vi "StrainElectrical.vi"(4 "Use Switching Matrix":bool=TRUE, 6 "Use Parameter Analyzer":bool=TRUE, 8 "Use Stress Control":bool=TRUE, 9 "Switching Matrix VISA Session":refnum<visa-resource-name>="GPIB0::18::INSTR", 10 "Pameter Analyzer VISA Session":refnum<visa-resource-name>="GPIB0::27::INSTR", 11 "Stress Controller VISA Session":refnum<visa-resource-name>="COM7") -> ()   [LabVIEW 2014]
uses:
  Measurements/Instrument Sequence/Instrument Steps.ctl
  Measurements/Instrument Sequence/Action.ctl
  Measurements/Instrument Sequence/Instrument List.ctl
  Measurements/Plot Data/Chooseplot.ctl
  support/Instrument Status.ctl
  Measurements/Instrument Sequence/Instrument Stequence - Which Program.ctl
  Hardware Control/Spectrometer/Spectrometer Config.ctl
  Hardware Control/Spectrometer/Laser Settings.ctl
  Hardware Control/Spectrometer/Laser.ctl
  Hardware Control/Spectrometer/Filter.ctl
  Hardware Control/Spectrometer/Grating Detector Settings.ctl
  Hardware Control/Spectrometer/Grating.ctl
  Hardware Control/Spectrometer/Detector.ctl
  Hardware Control/Spectrometer/Acquisition Settings.ctl
  Hardware Control/Spectrometer/Spectrometer Refnum.ctl
  Measurements/Plot Data/Optical Spectrum Plot Refnum.ctl
  Hardware Control/Switches and Mirrors/SwitchesMirrors Config.ctl
  Hardware Control/Switches and Mirrors/SwitchesMirrors Status.ctl
  Hardware Control/Camera/Camera Config.ctl
  Hardware Control/Camera/Camera Settings.ctl
  Hardware Control/Stress Control/StressControl Config.ctl
  Hardware Control/Stress Control/StressControl Refnums.ctl
  Hardware Control/Parameter Analyzer/Parameter Analyzer Config.ctl
  Hardware Control/Parameter Analyzer/Parameter Analyzer Integration Parameters.ctl
  Hardware Control/Parameter Analyzer/Parameter Analyzer SMU Sweeping.ctl
  Hardware Control/Parameter Analyzer/Parameter Analyzer Sweep Spacing.ctl
  Hardware Control/Parameter Analyzer/Parameter Analyzer SMU Range.ctl
  Hardware Control/Parameter Analyzer/Parameter Analyzer SMU Sampling.ctl
  Hardware Control/Parameter Analyzer/Parameter Analyzer Sampling Parameters.ctl
  Hardware Control/Parameter Analyzer/Parameter Analyzer Stop Sampling Conditions.ctl
  Hardware Control/Parameter Analyzer/Parameter Analyzer Refnums.ctl
  Measurements/Plot Data/Electrical Data Plot Refnums.ctl
  Hardware Control/Switching Matrix/Switching Matrix Config.ctl
  Hardware Control/Switching Matrix/Switching Matrix Refnums.ctl
  Hardware Control/XYZ Stage/XYZ Config.ctl
  Hardware Control/XYZ Stage/XYZ Connection Settings.ctl
  Hardware Control/XYZ Stage/XYZ Stage Control.ctl
  Hardware Control/XYZ Stage/XYZ Coordinate Control.ctl
  Hardware Control/Autofocus/AutoFocus Config.ctl
  Hardware Control/Autofocus/ZScan.ctl
  <vilib>/Analysis/Matrix/Datatypes/RealMatrix.ctl
  Measurements/Instrument Sequence/Instrument Sequence Refnums.ctl
  Measurements/Strain Measurement/Strain Measurement Config.ctl
  Measurements/Strain Measurement/Strain Measurement Refnums.ctl
  Measurements/Plot Data/PlotData Config.ctl
  Measurements/Plot Data/Measurement.ctl
  Measurements/Plot Data/WhichInstrument.ctl
  Hardware Control/Parameter Analyzer/Electrical Data.ctl
  Hardware Control/Spectrometer/Spectral Data.ctl
  Measurements/Plot Data/PlotData Refnums.ctl
  support/User Event - Stop/User Event - Stop.lvlib
  support/Message Queue/Message Queue.lvlib
  <vilib>/Analysis/Matrix/NI_Matrix.lvlib
panel:
  out "Strain Measurement - Device ID":string caption="Device ID"
  out "Strain Measurement - Device Information":string caption="Device Information"
  out "Instrument Sequence - Status":T2={"Parameter Analyzer"=TRUE, "Switching Matrix"=FALSE, "Stress Control"=FALSE} caption="Instrument Status"
  in  "Opto Electro Mechanics Functions":T3(tab)
  out "Strain Measurement - Steps":T4 caption="Instrument Sequence"
  in  "Strain Measurement - New Sequence":bool
  in  "Strain Measurement - Add Step":bool
  in  "Strain Measurement - Delete Step":bool
  in  "Strain Measurement - Save Sequence":bool
  in  "Strain Measurement - Load Sequence":bool
  in  "Measurement Choice":T7(tab)
  in  "Instrument Sequence - Start":bool
  in  "Instrument Sequence - Pause":bool
  in  "Instrument Sequence - Stop":bool
  in  "Strain Measurement - Start":bool
  in  "Strain Measurement - Pause":bool
  in  "Strain Measurement - Stop":bool
  out "Strain Measurement - Sequence Progress":cluster{i32[], "Y":dbl[]}[](graph)=[{[], "Y"=[]}, {[0], "Y"=[0.0]}, {[1, 2, 3, 4], "Y"=[0.0, 0.0, 0.0, 0.0]}] caption="Measurement Progress"
  in  "Strain Measurement - Stress Sequence Parameters":T8 caption="Stress Parameters" {"# Points" max=1390}
  out "PlotData - Configuration":string caption="Configuration"
  in  "PlotData - Strain Sequence":i32(slide) caption="Strain Sequence" scale=0.0..84.0
  in  "PlotData - Instrument Sequence":i32(slide) caption="Instrument Sequence" scale=0.0..5.0
  out "PlotData - Choose Plot":T9
  in  "PlotData - Electrical Plot List":T10(tab)
  out "PlotData - Current Plot":cluster{"Time":dbl[], "SMU4":dbl[]}[](graph)=[{"Time"=[0.0, 0.30000000000000004, 0.6000000000000001, 0.9, 1.2000000000000002, 1.5, 1.8, 2.1, 2.4000000000000004, 2.7, 3.0, 3.3000000000000003, 3.6, 3.9000000000000004, 4.2, 4.5, 4.800000000000001, 5.1000000000000005, 5.4, 5.7, 6.0, 6.300000000000001, 6.6000000000000005, 6.9, 7.2, 7.5, 7.800000000000001, 8.1, 8.4, 8.700000000000001, 9.0, 9.3, 9.600000000000001, 9.9, 10.200000000000001, 10.5, 10.8, 11.100000000000001, 11.4, 11.700000000000001, 12.0, 12.3, 12.600000000000001, 12.9, 13.200000000000001, 13.5, 13.8, 14.100000000000001, 14.4, 14.700000000000001, 15.0, 15.3, 15.600000000000001, 15.9, 16.2, 16.5, 16.8, 17.1, 17.400000000000002, 17.7], "SMU4"=[9.99995e-06, 9.99995e-06, 9.99995e-06, 9.99997e-06, 9.99997e-06, 9.99997e-06, 9.99997e-06, 9.999980000000001e-06, 9.99997e-06, 9.999980000000001e-06, 9.99997e-06, 9.999980000000001e-06, 9.99997e-06, 9.99997e-06, 9.99997e-06, 9.99996e-06, 9.99996e-06, 9.99996e-06, 9.99996e-06, 9.99997e-06, 9.99997e-06, 9.999980000000001e-06, 9.99997e-06, 9.99997e-06, 9.99997e-06, 9.99997e-06, 9.99997e-06, 9.999980000000001e-06, 9.999980000000001e-06, 9.99996e-06, 9.99997e-06, 9.99996e-06, 9.99997e-06, 9.99997e-06, 9.99997e-06, 9.99997e-06, 9.999980000000001e-06, 9.99997e-06, 9.999980000000001e-06, 9.999980000000001e-06, 9.99997e-06, 9.99997e-06, 9.99997e-06, 9.99996e-06, 9.99996e-06, 9.99997e-06, 9.99997e-06, 9.99996e-06, 9.99996e-06, 9.99997e-06, 9.99997e-06, 9.99997e-06, 9.99997e-06, 9.99997e-06, 9.99996e-06, 9.99997e-06, 9.99997e-06, 9.99997e-06, 9.99997e-06, 9.99996e-06]}, {"Time"=[0.0, 0.30000000000000004, 0.6000000000000001, 0.9, 1.2000000000000002, 1.5, 1.8, 2.1, 2.4000000000000004, 2.7, 3.0, 3.3000000000000003, 3.6, 3.9000000000000004, 4.2, 4.5, 4.800000000000001, 5.1000000000000005, 5.4, 5.7, 6.0, 6.300000000000001, 6.6000000000000005, 6.9, 7.2, 7.5, 7.800000000000001, 8.1, 8.4, 8.700000000000001, 9.0, 9.3, 9.600000000000001, 9.9, 10.200000000000001, 10.5, 10.8, 11.100000000000001, 11.4, 11.700000000000001, 12.0, 12.3, 12.600000000000001, 12.9, 13.200000000000001, 13.5, 13.8, 14.100000000000001, 14.4, 14.700000000000001, 15.0, 15.3, 15.600000000000001, 15.9, 16.2, 16.5, 16.8, 17.1, 17.400000000000002, 17.7], "SMU4"=[-1.00004e-05, -1.000039e-05, -1.000039e-05, -1.0000409999999999e-05, -1.000039e-05, -1.000039e-05, -1.00004e-05, -1.000043e-05, -1.000042e-05, -1.0000409999999999e-05, -1.000039e-05, -1.000039e-05, -1.0000409999999999e-05, -1.00004e-05, -1.000038e-05, -1.000038e-05, -1.000039e-05, -1.000037e-05, -1.000038e-05, -1.000039e-05, -1.000039e-05, -1.000039e-05, -1.000039e-05, -1.000039e-05, -1.00004e-05, -1.000037e-05, -1.000038e-05, -1.000039e-05, -1.00004e-05, -1.00004e-05, -1.00004e-05, -1.000037e-05, -1.000037e-05, -1.000037e-05, -1.000036e-05, -1.000039e-05, -1.000038e-05, -1.000037e-05, -1.000036e-05, -1.000037e-05, -1.000038e-05, -1.000037e-05, -1.000038e-05, -1.000036e-05, -1.000037e-05, -1.000037e-05, -1.000037e-05, -1.000039e-05, -1.000038e-05, -1.000036e-05, -1.000037e-05, -1.000039e-05, -1.000036e-05, -1.000037e-05, -1.000038e-05, -1.00004e-05, -1.0000409999999999e-05, -1.000038e-05, -1.000038e-05, -1.00004e-05]}]
  out "PlotData - Voltage Plot":cluster{"Time":dbl[], "SMU4":dbl[]}[](graph)=[{"Time"=[0.0, 0.30000000000000004, 0.6000000000000001, 0.9, 1.2000000000000002, 1.5, 1.8, 2.1, 2.4000000000000004, 2.7, 3.0, 3.3000000000000003, 3.6, 3.9000000000000004, 4.2, 4.5, 4.800000000000001, 5.1000000000000005, 5.4, 5.7, 6.0, 6.300000000000001, 6.6000000000000005, 6.9, 7.2, 7.5, 7.800000000000001, 8.1, 8.4, 8.700000000000001, 9.0, 9.3, 9.600000000000001, 9.9, 10.200000000000001, 10.5, 10.8, 11.100000000000001, 11.4, 11.700000000000001, 12.0, 12.3, 12.600000000000001, 12.9, 13.200000000000001, 13.5, 13.8, 14.100000000000001, 14.4, 14.700000000000001, 15.0, 15.3, 15.600000000000001, 15.9, 16.2, 16.5, 16.8, 17.1, 17.400000000000002, 17.7], "SMU4"=[9.99995e-06, 9.99995e-06, 9.99995e-06, 9.99997e-06, 9.99997e-06, 9.99997e-06, 9.99997e-06, 9.999980000000001e-06, 9.99997e-06, 9.999980000000001e-06, 9.99997e-06, 9.999980000000001e-06, 9.99997e-06, 9.99997e-06, 9.99997e-06, 9.99996e-06, 9.99996e-06, 9.99996e-06, 9.99996e-06, 9.99997e-06, 9.99997e-06, 9.999980000000001e-06, 9.99997e-06, 9.99997e-06, 9.99997e-06, 9.99997e-06, 9.99997e-06, 9.999980000000001e-06, 9.999980000000001e-06, 9.99996e-06, 9.99997e-06, 9.99996e-06, 9.99997e-06, 9.99997e-06, 9.99997e-06, 9.99997e-06, 9.999980000000001e-06, 9.99997e-06, 9.999980000000001e-06, 9.999980000000001e-06, 9.99997e-06, 9.99997e-06, 9.99997e-06, 9.99996e-06, 9.99996e-06, 9.99997e-06, 9.99997e-06, 9.99996e-06, 9.99996e-06, 9.99997e-06, 9.99997e-06, 9.99997e-06, 9.99997e-06, 9.99997e-06, 9.99996e-06, 9.99997e-06, 9.99997e-06, 9.99997e-06, 9.99997e-06, 9.99996e-06]}, {"Time"=[0.0, 0.30000000000000004, 0.6000000000000001, 0.9, 1.2000000000000002, 1.5, 1.8, 2.1, 2.4000000000000004, 2.7, 3.0, 3.3000000000000003, 3.6, 3.9000000000000004, 4.2, 4.5, 4.800000000000001, 5.1000000000000005, 5.4, 5.7, 6.0, 6.300000000000001, 6.6000000000000005, 6.9, 7.2, 7.5, 7.800000000000001, 8.1, 8.4, 8.700000000000001, 9.0, 9.3, 9.600000000000001, 9.9, 10.200000000000001, 10.5, 10.8, 11.100000000000001, 11.4, 11.700000000000001, 12.0, 12.3, 12.600000000000001, 12.9, 13.200000000000001, 13.5, 13.8, 14.100000000000001, 14.4, 14.700000000000001, 15.0, 15.3, 15.600000000000001, 15.9, 16.2, 16.5, 16.8, 17.1, 17.400000000000002, 17.7], "SMU4"=[-1.00004e-05, -1.000039e-05, -1.000039e-05, -1.0000409999999999e-05, -1.000039e-05, -1.000039e-05, -1.00004e-05, -1.000043e-05, -1.000042e-05, -1.0000409999999999e-05, -1.000039e-05, -1.000039e-05, -1.0000409999999999e-05, -1.00004e-05, -1.000038e-05, -1.000038e-05, -1.000039e-05, -1.000037e-05, -1.000038e-05, -1.000039e-05, -1.000039e-05, -1.000039e-05, -1.000039e-05, -1.000039e-05, -1.00004e-05, -1.000037e-05, -1.000038e-05, -1.000039e-05, -1.00004e-05, -1.00004e-05, -1.00004e-05, -1.000037e-05, -1.000037e-05, -1.000037e-05, -1.000036e-05, -1.000039e-05, -1.000038e-05, -1.000037e-05, -1.000036e-05, -1.000037e-05, -1.000038e-05, -1.000037e-05, -1.000038e-05, -1.000036e-05, -1.000037e-05, -1.000037e-05, -1.000037e-05, -1.000039e-05, -1.000038e-05, -1.000036e-05, -1.000037e-05, -1.000039e-05, -1.000036e-05, -1.000037e-05, -1.000038e-05, -1.00004e-05, -1.0000409999999999e-05, -1.000038e-05, -1.000038e-05, -1.00004e-05]}]
  out "PlotData - dI/dV-V Characteristic":cluster{"V3":dbl[], "I1":dbl[]}[](graph) caption="Differential Resistance"
  out "PlotData - IV Characteristic":cluster{"V3":dbl[], "I1":dbl[]}[](graph) caption="Current Voltage Characteristic"
  out "PlotData - Optical Spectrum":cluster{"data":dbl[], "data":dbl[]}(graph)
  in  "Acquisition Mode":enum32{"Sweeping Mode", "Sampling Mode"}(tab)
  in  "SMU 4 - Sweeping":T11={"Start / Offset"=0.0, "Stop / Ratio"=1.0, "Step \n(linear only)"=0.01, "Compliance"=0.1, "Power \nCompliance"=0.0, "Mode"=4, "Function"=4, "Sweep Mode"=FALSE} caption="SMU 4" {"Function" items=["Disabled", "Var 1", "Var 2", "Var 1'", "Constant"]; "Mode" items=["V", "I", "V pulse", "I  pulse", "Common"]; "Power \nCompliance" format="%^.2e"; "Compliance" format="%^.2e"; "Step \n(linear only)" format="%^.4e"; "Stop / Ratio" format="%^.4e"; "Start / Offset" format="%^.4e"}
  in  "SMU 3 - Sweeping":T11={"Start / Offset"=0.0, "Stop / Ratio"=1.0, "Step \n(linear only)"=0.01, "Compliance"=0.1, "Power \nCompliance"=0.0, "Mode"=1, "Function"=4, "Sweep Mode"=FALSE} caption="SMU 3" {"Function" items=["Disabled", "Var 1", "Var 2", "Var 1'", "Constant"]; "Mode" items=["V", "I", "V pulse", "I  pulse", "Common"]; "Power \nCompliance" format="%^.2e"; "Compliance" format="%^.2e"; "Step \n(linear only)" format="%^.4e"; "Stop / Ratio" format="%^.4e"; "Start / Offset" format="%^.4e"}
  in  "SMU 2 - Sweeping":T11={"Start / Offset"=0.0, "Stop / Ratio"=1.0, "Step \n(linear only)"=0.01, "Compliance"=0.1, "Power \nCompliance"=0.0, "Mode"=1, "Function"=4, "Sweep Mode"=FALSE} caption="SMU 2" {"Function" items=["Disabled", "Var 1", "Var 2", "Var 1'", "Constant"]; "Mode" items=["V", "I", "V pulse", "I  pulse", "Common"]; "Power \nCompliance" format="%^.2e"; "Compliance" format="%^.2e"; "Step \n(linear only)" format="%^.4e"; "Stop / Ratio" format="%^.4e"; "Start / Offset" format="%^.4e"}
  in  "SMU 1 - Sweeping":T11={"Start / Offset"=0.0, "Stop / Ratio"=0.15, "Step \n(linear only)"=0.01, "Compliance"=0.1, "Power \nCompliance"=0.0, "Mode"=0, "Function"=1, "Sweep Mode"=TRUE} caption="SMU 1" {"Function" items=["Disabled", "Var 1", "Var 2", "Var 1'", "Constant"]; "Mode" items=["V", "I", "V pulse", "I  pulse", "Common"]; "Power \nCompliance" format="%^.2e"; "Compliance" format="%^.2e"; "Step \n(linear only)" format="%^.4e"; "Stop / Ratio" format="%^.4e"; "Start / Offset" format="%^.4e"}
  in  "Sweep Spacing":u16(ring) items=["linear", "log 10", "log 25", "log 50"]
  in  "Range":u16(ring) items=["auto", "fixed", "limited"]
  in  "Apply Sweeping Settings":bool
  in  "SMU4 - Sampling":T12={"Source"=0.1, "Compliance"=60.0, "Mode"=2, "Function"=TRUE} caption="SMU 4" {"Mode" items=["V", "I", "Common"]; "Compliance" format="%^.2e"; "Source" format="%^.3e"}
  in  "SMU2 - Sampling":T12={"Source"=0.0, "Compliance"=0.15, "Mode"=1, "Function"=TRUE} caption="SMU 2" {"Mode" items=["V", "I", "Common"]; "Compliance" format="%^.2e"; "Source" format="%^.3e"}
  in  "SMU3 - Sampling":T12={"Source"=0.0, "Compliance"=0.15, "Mode"=1, "Function"=TRUE} caption="SMU 3" {"Mode" items=["V", "I", "Common"]; "Compliance" format="%^.2e"; "Source" format="%^.3e"}
  in  "SMU1 - Sampling":T12={"Source"=0.15, "Compliance"=0.1, "Mode"=0, "Function"=TRUE} caption="SMU 1" {"Mode" items=["V", "I", "Common"]; "Compliance" format="%^.2e"; "Source" format="%^.3e"}
  in  "Stop Condition":T13={"Enable Delay (s)"=0.0, "Name"="", "Threshold"=0.0, "num. of events"=1, "Event"=0, "Stop Condition Enable"=FALSE} {"Event" items=["Value > Threshold", "Value < Threshold", "| Value | > | Threshold |", "| Value | < | Threshold |"]; "Threshold" format="%^.2e"; "Enable Delay (s)" format="%.1f"}
  in  "Sampling Parameters":T14={"Initial Interval (s)"=0.1, "Number of Samples"=60, "Total Sampling Time (s)"=10.0, "Hold Time (s)"=0.0, "Sampling Mode"=0, "Sampling Time"=0} {"Sampling Time" items=["Auto (linear only)", "No Limit", "Set Limit"]; "Sampling Mode" items=["Linear", "Log10", "Log25", "Log50", "Thinned Out"]; "Hold Time (s)" format="%.4f"; "Total Sampling Time (s)" format="%.1f"; "Initial Interval (s)" format="%^.3e"}
  in  "Apply Sampling Settings":bool
  in  "User Integration Time":T15={"Integration Time"=0, "Short Integration Time (s)"=8e-05, "Long Integration Time (s)"=0.0, "Wait Time Parameter"=1.0} caption="Input Integration Time" {"Long Integration Time (s)" scale=0.02..2.0; "Short Integration Time (s)" scale=8e-05..0.00192; "Integration Time" items=["Short", "Long"]; "Wait Time Parameter" format="%.1f"}
  in  "Plot List":T10(tab)
  out "Current Plot":cluster{"Time":dbl[], "SMU4":dbl[]}[](graph)=[{"Time"=[0.0, 0.30000000000000004, 0.6000000000000001, 0.9, 1.2000000000000002, 1.5, 1.8, 2.1, 2.4000000000000004, 2.7, 3.0, 3.3000000000000003, 3.6, 3.9000000000000004, 4.2, 4.5, 4.800000000000001, 5.1000000000000005, 5.4, 5.7, 6.0, 6.300000000000001, 6.6000000000000005, 6.9, 7.2, 7.5, 7.800000000000001, 8.1, 8.4, 8.700000000000001, 9.0, 9.3, 9.600000000000001, 9.9, 10.200000000000001, 10.5, 10.8, 11.100000000000001, 11.4, 11.700000000000001, 12.0, 12.3, 12.600000000000001, 12.9, 13.200000000000001, 13.5, 13.8, 14.100000000000001, 14.4, 14.700000000000001, 15.0, 15.3, 15.600000000000001, 15.9, 16.2, 16.5, 16.8, 17.1, 17.400000000000002, 17.7], "SMU4"=[9.99995e-06, 9.99995e-06, 9.99995e-06, 9.99997e-06, 9.99997e-06, 9.99997e-06, 9.99997e-06, 9.999980000000001e-06, 9.99997e-06, 9.999980000000001e-06, 9.99997e-06, 9.999980000000001e-06, 9.99997e-06, 9.99997e-06, 9.99997e-06, 9.99996e-06, 9.99996e-06, 9.99996e-06, 9.99996e-06, 9.99997e-06, 9.99997e-06, 9.999980000000001e-06, 9.99997e-06, 9.99997e-06, 9.99997e-06, 9.99997e-06, 9.99997e-06, 9.999980000000001e-06, 9.999980000000001e-06, 9.99996e-06, 9.99997e-06, 9.99996e-06, 9.99997e-06, 9.99997e-06, 9.99997e-06, 9.99997e-06, 9.999980000000001e-06, 9.99997e-06, 9.999980000000001e-06, 9.999980000000001e-06, 9.99997e-06, 9.99997e-06, 9.99997e-06, 9.99996e-06, 9.99996e-06, 9.99997e-06, 9.99997e-06, 9.99996e-06, 9.99996e-06, 9.99997e-06, 9.99997e-06, 9.99997e-06, 9.99997e-06, 9.99997e-06, 9.99996e-06, 9.99997e-06, 9.99997e-06, 9.99997e-06, 9.99997e-06, 9.99996e-06]}, {"Time"=[0.0, 0.30000000000000004, 0.6000000000000001, 0.9, 1.2000000000000002, 1.5, 1.8, 2.1, 2.4000000000000004, 2.7, 3.0, 3.3000000000000003, 3.6, 3.9000000000000004, 4.2, 4.5, 4.800000000000001, 5.1000000000000005, 5.4, 5.7, 6.0, 6.300000000000001, 6.6000000000000005, 6.9, 7.2, 7.5, 7.800000000000001, 8.1, 8.4, 8.700000000000001, 9.0, 9.3, 9.600000000000001, 9.9, 10.200000000000001, 10.5, 10.8, 11.100000000000001, 11.4, 11.700000000000001, 12.0, 12.3, 12.600000000000001, 12.9, 13.200000000000001, 13.5, 13.8, 14.100000000000001, 14.4, 14.700000000000001, 15.0, 15.3, 15.600000000000001, 15.9, 16.2, 16.5, 16.8, 17.1, 17.400000000000002, 17.7], "SMU4"=[-1.00004e-05, -1.000039e-05, -1.000039e-05, -1.0000409999999999e-05, -1.000039e-05, -1.000039e-05, -1.00004e-05, -1.000043e-05, -1.000042e-05, -1.0000409999999999e-05, -1.000039e-05, -1.000039e-05, -1.0000409999999999e-05, -1.00004e-05, -1.000038e-05, -1.000038e-05, -1.000039e-05, -1.000037e-05, -1.000038e-05, -1.000039e-05, -1.000039e-05, -1.000039e-05, -1.000039e-05, -1.000039e-05, -1.00004e-05, -1.000037e-05, -1.000038e-05, -1.000039e-05, -1.00004e-05, -1.00004e-05, -1.00004e-05, -1.000037e-05, -1.000037e-05, -1.000037e-05, -1.000036e-05, -1.000039e-05, -1.000038e-05, -1.000037e-05, -1.000036e-05, -1.000037e-05, -1.000038e-05, -1.000037e-05, -1.000038e-05, -1.000036e-05, -1.000037e-05, -1.000037e-05, -1.000037e-05, -1.000039e-05, -1.000038e-05, -1.000036e-05, -1.000037e-05, -1.000039e-05, -1.000036e-05, -1.000037e-05, -1.000038e-05, -1.00004e-05, -1.0000409999999999e-05, -1.000038e-05, -1.000038e-05, -1.00004e-05]}]
  out "Voltage Plot":cluster{"Time":dbl[], "SMU4":dbl[]}[](graph)=[{"Time"=[0.0, 0.30000000000000004, 0.6000000000000001, 0.9, 1.2000000000000002, 1.5, 1.8, 2.1, 2.4000000000000004, 2.7, 3.0, 3.3000000000000003, 3.6, 3.9000000000000004, 4.2, 4.5, 4.800000000000001, 5.1000000000000005, 5.4, 5.7, 6.0, 6.300000000000001, 6.6000000000000005, 6.9, 7.2, 7.5, 7.800000000000001, 8.1, 8.4, 8.700000000000001, 9.0, 9.3, 9.600000000000001, 9.9, 10.200000000000001, 10.5, 10.8, 11.100000000000001, 11.4, 11.700000000000001, 12.0, 12.3, 12.600000000000001, 12.9, 13.200000000000001, 13.5, 13.8, 14.100000000000001, 14.4, 14.700000000000001, 15.0, 15.3, 15.600000000000001, 15.9, 16.2, 16.5, 16.8, 17.1, 17.400000000000002, 17.7], "SMU4"=[9.99995e-06, 9.99995e-06, 9.99995e-06, 9.99997e-06, 9.99997e-06, 9.99997e-06, 9.99997e-06, 9.999980000000001e-06, 9.99997e-06, 9.999980000000001e-06, 9.99997e-06, 9.999980000000001e-06, 9.99997e-06, 9.99997e-06, 9.99997e-06, 9.99996e-06, 9.99996e-06, 9.99996e-06, 9.99996e-06, 9.99997e-06, 9.99997e-06, 9.999980000000001e-06, 9.99997e-06, 9.99997e-06, 9.99997e-06, 9.99997e-06, 9.99997e-06, 9.999980000000001e-06, 9.999980000000001e-06, 9.99996e-06, 9.99997e-06, 9.99996e-06, 9.99997e-06, 9.99997e-06, 9.99997e-06, 9.99997e-06, 9.999980000000001e-06, 9.99997e-06, 9.999980000000001e-06, 9.999980000000001e-06, 9.99997e-06, 9.99997e-06, 9.99997e-06, 9.99996e-06, 9.99996e-06, 9.99997e-06, 9.99997e-06, 9.99996e-06, 9.99996e-06, 9.99997e-06, 9.99997e-06, 9.99997e-06, 9.99997e-06, 9.99997e-06, 9.99996e-06, 9.99997e-06, 9.99997e-06, 9.99997e-06, 9.99997e-06, 9.99996e-06]}, {"Time"=[0.0, 0.30000000000000004, 0.6000000000000001, 0.9, 1.2000000000000002, 1.5, 1.8, 2.1, 2.4000000000000004, 2.7, 3.0, 3.3000000000000003, 3.6, 3.9000000000000004, 4.2, 4.5, 4.800000000000001, 5.1000000000000005, 5.4, 5.7, 6.0, 6.300000000000001, 6.6000000000000005, 6.9, 7.2, 7.5, 7.800000000000001, 8.1, 8.4, 8.700000000000001, 9.0, 9.3, 9.600000000000001, 9.9, 10.200000000000001, 10.5, 10.8, 11.100000000000001, 11.4, 11.700000000000001, 12.0, 12.3, 12.600000000000001, 12.9, 13.200000000000001, 13.5, 13.8, 14.100000000000001, 14.4, 14.700000000000001, 15.0, 15.3, 15.600000000000001, 15.9, 16.2, 16.5, 16.8, 17.1, 17.400000000000002, 17.7], "SMU4"=[-1.00004e-05, -1.000039e-05, -1.000039e-05, -1.0000409999999999e-05, -1.000039e-05, -1.000039e-05, -1.00004e-05, -1.000043e-05, -1.000042e-05, -1.0000409999999999e-05, -1.000039e-05, -1.000039e-05, -1.0000409999999999e-05, -1.00004e-05, -1.000038e-05, -1.000038e-05, -1.000039e-05, -1.000037e-05, -1.000038e-05, -1.000039e-05, -1.000039e-05, -1.000039e-05, -1.000039e-05, -1.000039e-05, -1.00004e-05, -1.000037e-05, -1.000038e-05, -1.000039e-05, -1.00004e-05, -1.00004e-05, -1.00004e-05, -1.000037e-05, -1.000037e-05, -1.000037e-05, -1.000036e-05, -1.000039e-05, -1.000038e-05, -1.000037e-05, -1.000036e-05, -1.000037e-05, -1.000038e-05, -1.000037e-05, -1.000038e-05, -1.000036e-05, -1.000037e-05, -1.000037e-05, -1.000037e-05, -1.000039e-05, -1.000038e-05, -1.000036e-05, -1.000037e-05, -1.000039e-05, -1.000036e-05, -1.000037e-05, -1.000038e-05, -1.00004e-05, -1.0000409999999999e-05, -1.000038e-05, -1.000038e-05, -1.00004e-05]}]
  out "Differential Resistance":cluster{"V3":dbl[], "I1":dbl[]}[](graph)
  out "Current Voltage Characteristic":cluster{"V3":dbl[], "I1":dbl[]}[](graph)
  in  "Parameter Analyzer - Measure":bool
  in  "Parameter Analyzer - Save Measurement":bool
  in  "Switching Matrix":enum32{"Switching Matrix"}(tab)
  in  "Switching Matrix Connections":T16(array[cluster])=[{"Connections"=[FALSE, FALSE, FALSE, FALSE, FALSE, FALSE, FALSE, FALSE, FALSE, FALSE, FALSE, FALSE], "Connection Type"=enum."Make - Break"}, {"Connections"=[FALSE, FALSE, FALSE, FALSE, FALSE, FALSE, FALSE, FALSE, FALSE, FALSE, FALSE, FALSE], "Connection Type"=enum."Make - Break"}, {"Connections"=[FALSE, FALSE, FALSE, FALSE, FALSE, FALSE, FALSE, FALSE, FALSE, FALSE, FALSE, FALSE], "Connection Type"=enum."Make - Break"}, {"Connections"=[FALSE, FALSE, FALSE, FALSE, FALSE, FALSE, FALSE, FALSE, FALSE, FALSE, FALSE, FALSE], "Connection Type"=enum."Make - Break"}, {"Connections"=[TRUE, TRUE, TRUE, TRUE, TRUE, TRUE, TRUE, TRUE, TRUE, TRUE, TRUE, TRUE], "Connection Type"=enum."Make - Break"}, {"Connections"=[FALSE, FALSE, FALSE, FALSE, FALSE, FALSE, FALSE, FALSE, FALSE, FALSE, FALSE, FALSE], "Connection Type"=enum."Make - Break"}, {"Connections"=[FALSE, FALSE, FALSE, FALSE, FALSE, FALSE, FALSE, FALSE, FALSE, FALSE, FALSE, FALSE], "Connection Type"=enum."Make - Break"}, {"Connections"=[FALSE, FALSE, FALSE, FALSE, FALSE, FALSE, FALSE, FALSE, FALSE, FALSE, FALSE, FALSE], "Connection Type"=enum."Make - Break"}]
  in  "Disconnect All":bool
  in  "Ground All":bool
  in  "Uniaxial Stress Controller":enum32{"Uniaxial Stress Controller"}(tab)
  in  "Destination (°)":dbl min=-2000000000.0 max=2000000000.0 format="%.6f"
  out "Position (°)":dbl format="%.6g"
  in  "Mechanism Motion":u16(ring) items=["Absolute", "Relative"]
  in  "Apply Stress":bool
  in  "Stop":bool
  in  "Speed (°/s)":dbl=4.0 min=0.0 max=4.0 format="%.6f"
  in  "Status Polling Time (ms)":u32=500
  out "Status Log":string
  out "Last Operation":string="Camera Settings Updated"
  # "SMU1"
  # "SMU2"
  # "SMU3"
  # "SMU4"
  # "GND"
  # "L1"
  # "R1"
  # "L2"
  # "R2"
  # "L3"
  # "R3"
  # "L6"
  # "R6"
  # "L7"
  # "R7"
  # "L8"
  # "R8"
  # "LICENSED MATERIALS – PROPERTY OF IBM\nCopyright IBM Corp. 2016,\nALL RIGHTS RESERVED"
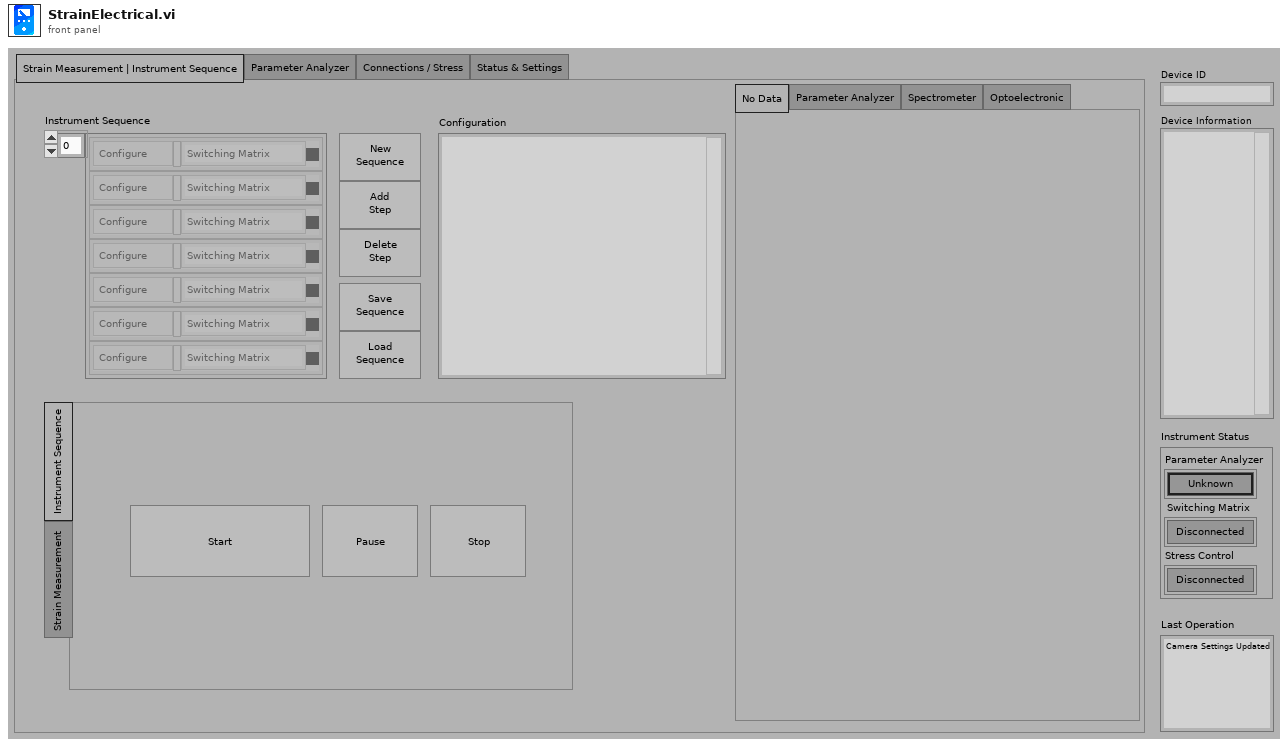
[diagram p1: front panel]
types:
  T1 = typedef "Instrument Status.ctl" = bool
  T2 = cluster{"Parameter Analyzer":T1, "Switching Matrix":T1, "Stress Control":T1}
  T3 = enum32{"Strain Measurement | Instrument Sequence", "Parameter Analyzer", "Connections / Stress", "Status & Settings"}
  T4 = typedef "Instrument Steps.ctl" = cluster{"Action":T5, "Configuration":variant, "Instrument":T6, "Status":enum8{"False", "True", "Mixed"}}[]
  T5 = typedef "Action.ctl" = enum32{"Configure", "Measure"}
  T6 = typedef "Instrument List.ctl" = enum32{"Unknown Instrument", "Switching Matrix", "Parameter Analyzer", "Optical Spectrometer", "Optoelectronic", "Autofocus"}
  T7 = enum32{"Instrument Sequence", "Strain Measurement "}
  T8 = cluster{"Max Stress":ext, "# Points":u32, "Initial Direction":enum16{"Tension", "Compression"}}
  T9 = typedef "Chooseplot.ctl" = enum32{"No Data", "Parameter Analyzer", "Spectrometer", "Optoelectronic"}
  T10 = enum32{"Current & Voltage Traces", "Four | Two Probe"}
  T11 = cluster{"Start / Offset":dbl, "Stop / Ratio":dbl, "Step \n(linear only)":dbl, "Compliance":dbl, "Power \nCompliance":dbl, "Mode":u32, "Function":i32, "Sweep Mode":bool}
  T12 = cluster{"Source":dbl, "Compliance":dbl, "Mode":u32, "Function":bool}
  T13 = cluster{"Enable Delay (s)":dbl, "Name":string, "Threshold":dbl, "num. of events":i32, "Event":i32, "Stop Condition Enable":bool}
  T14 = cluster{"Initial Interval (s)":dbl, "Number of Samples":i32, "Total Sampling Time (s)":dbl, "Hold Time (s)":dbl, "Sampling Mode":i32, "Sampling Time":i32}
  T15 = cluster{"Integration Time":u32, "Short Integration Time (s)":dbl, "Long Integration Time (s)":dbl, "Wait Time Parameter":dbl}
  T16 = cluster{"Connections":bool[], "Connection Type":enum16{"Disconnected", "Make - Break", "Break - Make"}}[]
  T17 = typedef "Instrument Stequence - Which Program.ctl" = enum16{"Full Instrument Palette", "Strain Electrical"}
  T18 = typedef "Message Queue.lvlib/All Message Queues.ctl" = cluster{"Message Handler Loop":refnum<queue>, "Parameter Analyzer":refnum<queue>, "Switching Matrix":refnum<queue>, "Stress Control":refnum<queue>, "Optical Spectrometer":refnum<queue>, "Switches & Mirrors":refnum<queue>, "Camera":refnum<queue>, "XYZ Stage":refnum<queue>, "AutoFocus":refnum<queue>, "Optoelectronic":refnum<queue>, "Save Data":refnum<queue>, "Plot Data":refnum<queue>, "Instrument Sequence":refnum<queue>, "Strain Measurement":refnum<queue>}
  T19 = typedef "Notifiers.ctl" = cluster{"Message Handler Loop":T20, "Parameter Analyzer":T21, "Switching Matrix":T22, "Stress Control":T23, "Optical Spectrometer":T24, "Switches & Mirrors":T25, "Camera":T26, "XYZ Stage":T27, "AutoFocus":T28, "Optoelectronic":T29, "Save Data":T30, "Plot Data":T30, "Instrument Sequence":T31, "Strain Measurement":cluster{"Status":refnum<notifier>, "Exit":refnum<notifier>, "Ready":refnum<notifier>}}
  T20 = typedef "Message Handler Loop Notifiers.ctl" = cluster{"Status":refnum<notifier>, "Instrument Data":refnum<notifier>, "Exit":refnum<notifier>, "Ready":refnum<notifier>}
  T21 = typedef "Parameter Analyzer Notifiers.ctl" = cluster{"Status":refnum<notifier>, "Instrument Data":refnum<notifier>, "Measurement":refnum<notifier>, "Exit":refnum<notifier>, "Ready":refnum<notifier>}
  T22 = typedef "Switching Matrix Notifiers.ctl" = cluster{"Status":refnum<notifier>, "Instrument Data":refnum<notifier>, "Measurement":refnum<notifier>, "Exit":refnum<notifier>, "Ready":refnum<notifier>}
  T23 = typedef "StressControl Notifiers.ctl" = cluster{"Status":refnum<notifier>, "Instrument Data":refnum<notifier>, "Measurement":refnum<notifier>, "Exit":refnum<notifier>, "Ready":refnum<notifier>}
  T24 = typedef "Spectrometer Notifiers.ctl" = cluster{"Status":refnum<notifier>, "Instrument Data":refnum<notifier>, "Measurement":refnum<notifier>, "Exit":refnum<notifier>, "Ready":refnum<notifier>}
  T25 = typedef "SwitchesMirrors Notifiers.ctl" = cluster{"Status":refnum<notifier>, "Instrument Data":refnum<notifier>, "Exit":refnum<notifier>, "Ready":refnum<notifier>}
  T26 = typedef "Camera Notifiers.ctl" = cluster{"Status":refnum<notifier>, "Instrument Data":refnum<notifier>, "Measurement":refnum<notifier>, "Exit":refnum<notifier>, "Ready":refnum<notifier>}
  T27 = typedef "XYZ Notifications.ctl" = cluster{"Status":refnum<notifier>, "Instrument Data":refnum<notifier>, "Measurement":refnum<notifier>, "Exit":refnum<notifier>, "Ready":refnum<notifier>}
  T28 = typedef "Autofocus Notifiers.ctl" = cluster{"Status":refnum<notifier>, "Instrument Data":refnum<notifier>, "Measurement":refnum<notifier>, "Exit":refnum<notifier>, "Ready":refnum<notifier>}
  T29 = typedef "Optoelectronic Notifiers.ctl" = cluster{"Status":refnum<notifier>, "Instrument Data":refnum<notifier>, "Measurement":refnum<notifier>, "Exit":refnum<notifier>, "Ready":refnum<notifier>}
  T30 = typedef "SaveData Notifiers.ctl" = cluster{"Status":refnum<notifier>, "Exit":refnum<notifier>, "Ready":refnum<notifier>}
  T31 = typedef "Instrument Sequence Notifiers.ctl" = cluster{"Status":refnum<notifier>, "Instrument Data":refnum<notifier>, "Measurement":refnum<notifier>, "Exit":refnum<notifier>, "Ready":refnum<notifier>}
  T32 = typedef "Configuration.ctl" = cluster{"Parameter Analizer":T33, "Switching Matrix":T41, "Stress Control":T42, "Optical Spectrometer":T43, "Switches & Mirrors":T51, "Camera":T53, "XYZ Stage":T55, "AutoFocus":T59, "Sava Data":T62, "PlotData":T66, "Instrument Sequence":T70, "Strain Measurement":T71}
  T33 = typedef "Parameter Analyzer Config.ctl" = cluster{"Parameter Analyzer VISA Session":refnum<visa-resource-name>, "Sweeping Time Parameters":T34, "Acquisition Mode":enum32{"Sweeping Mode", "Sampling Mode"}, "Status Polling Time (ms)":u32, "Comment":string, "SMU 1 - Sweeping":T35, "SMU 2 - Sweeping":T35, "SMU 3 - Sweeping":T35, "SMU 4 - Sweeping":T35, "Sweep Spacing":T36, "Range":T37, "SMU1 - Sampling":T38, "SMU2 - Sampling":T38, "SMU3 - Sampling":T38, "SMU4 - Sampling":T38, "Sampling Time Parameters":T39, "Stop Condition":T40}
  T34 = typedef "Parameter Analyzer Integration Parameters.ctl" = cluster{"Integration Time":u32, "Short Integration Time (s)":dbl, "Long Integration Time (s)":dbl, "Wait Time Parameter":dbl}
  T35 = typedef "Parameter Analyzer SMU Sweeping.ctl" = cluster{"Start / Offset":dbl, "Stop / Ratio":dbl, "Step \n(linear only)":dbl, "Compliance":dbl, "Power \nCompliance":dbl, "Mode":u32, "Function":i32, "Sweep Mode":bool}
  T36 = typedef "Parameter Analyzer Sweep Spacing.ctl" = u16
  T37 = typedef "Parameter Analyzer SMU Range.ctl" = u16
  T38 = typedef "Parameter Analyzer SMU Sampling.ctl" = cluster{"Source":dbl, "Compliance":dbl, "Mode":u32, "Function":bool}
  T39 = typedef "Parameter Analyzer Sampling Parameters.ctl" = cluster{"Initial Interval (s)":dbl, "Number of Samples":i32, "Total Sampling Time (s)":dbl, "Hold Time (s)":dbl, "Sampling Mode":i32, "Sampling Time":i32}
  T40 = typedef "Parameter Analyzer Stop Sampling Conditions.ctl" = cluster{"Enable Delay (s)":dbl, "Name":string, "Threshold":dbl, "num. of events":i32, "Event":i32, "Stop Condition Enable":bool}
  T41 = typedef "Switching Matrix Config.ctl" = cluster{"Switching Matrix VISA Session":refnum<visa-resource-name>, "Connections":cluster{"Connections":bool[], "Connection Type":enum16{"Disconnected", "Make - Break", "Break - Make"}}[]}
  T42 = typedef "StressControl Config.ctl" = cluster{"Stress Control VISA Session":refnum<visa-resource-name>, "Axis":i32, "Motion":u16, "Destination (°)":dbl, "Speed (°/s)":dbl, "Position (°)":dbl}
  T43 = typedef "Spectrometer Config.ctl" = cluster{"Laser Settings":T44, "Spectrometer Settings":T47, "Acquisition Settings":T50, "Path":path}
  T44 = typedef "Laser Settings.ctl" = cluster{"Laser Wavelength":T45, "Neutral Density Filter":T46}
  T45 = typedef "Laser.ctl" = enum16{"633 nm", "784 nm", "532 nm", "365 nm"}
  T46 = typedef "Filter.ctl" = enum16{"100%", "50%", "25%", "10%", "1%", "0.1%", "0.01%"}
  T47 = typedef "Grating Detector Settings.ctl" = cluster{"Confocal Hole Size (µm)":dbl, "Grating":T48, "Detector":T49}
  T48 = typedef "Grating.ctl" = u16
  T49 = typedef "Detector.ctl" = enum16{"InGaAs Array", "Silicon CCD"}
  T50 = typedef "Acquisition Settings.ctl" = cluster{"Acquisition Mode":enum16{"Single Window", "Multi-Window"}, "Spectal Position (nm)":dbl, "From (nm)":dbl, "To (nm)":dbl, "Integration Time (s)":dbl, "Number of Accumulations":i32, "AutoScanning":bool, "Spike Removal":bool}
  T51 = typedef "SwitchesMirrors Config.ctl" = cluster{"Relay VISA Session":refnum<visa-resource-name>, "Switches":T52, "Delays (ms)":cluster{"Laser":u32, "Video":u32}}
  T52 = typedef "SwitchesMirrors Status.ctl" = cluster{"Laser":bool, "Video":bool}
  T53 = typedef "Camera Config.ctl" = cluster{"Settings":T54}
  T54 = typedef "Camera Settings.ctl" = cluster{"Pixel clock":i32, "Frame rate":dbl, "Exposure time":dbl, "Master Gain":i32, "Red Gain":i32, "Green Gain":i32, "Blue Gain":i32, "Auto Gain":bool, "White-balance":bool, "Color Correction":bool}
  T55 = typedef "XYZ Config.ctl" = cluster{"Connection Settings":T56, "Manual Control":T57, "Coordinate Control":T58}
  T56 = typedef "XYZ Connection Settings.ctl" = cluster{"Tango VISA":refnum<visa-resource-name>, "Baudrate":i32, "Show Protocol?":bool}
  T57 = typedef "XYZ Stage Control.ctl" = cluster{"North":bool, "South":bool, "West":bool, "East":bool, "Up":bool, "Down":bool, "Stop":bool, "XY Step":dbl, "Z step":dbl}
  T58 = typedef "XYZ Coordinate Control.ctl" = cluster{"Motion Mode":enum16{"Absolute", "Relative"}, "Destination [mm]":dbl[]}
  T59 = typedef "AutoFocus Config.ctl" = cluster{"Matching Criteria":cluster{"Minimum Score":sgl, "Color Score Weight":sgl, "Minimum Contrast":i32, "Match Mode":u32, "Match Feature Mode":u32, "Subpixel Accuracy":bool, "Color Sensitivity":u32, "Search Strategy":u32}, "Z Scan Parameters":T60, "Displacement":dbl, "Transformation Matrix":T61}
  T60 = typedef "ZScan.ctl" = cluster{"Z Range":ext, "Resolution":dbl, "Initial Direction":enum16{"Up", "Down"}, "Focus Threshold":dbl, "Ascent Constant":dbl}
  T61 = typedef "NI_Matrix.lvlib/RealMatrix.ctl" = dbl[][]
  T62 = typedef "SaveData Config.ctl" = cluster{"Workspace Info":T63, "Instrument Configuration":T64, "Stress Motor Position":dbl, "Electrical Measurement":cluster{"Sequence":dbl[], "V1":dbl[], "V2":dbl[], "V3":dbl[], "V4":dbl[], "I1":dbl[], "I2":dbl[], "I3":dbl[], "I4":dbl[]}, "Optical Spectrum":T65}
  T63 = typedef "SaveData Workspace Info.ctl" = cluster{"Device Name":string, "Device Info":string, "Path":path}
  T64 = typedef "SaveData Instrument Configuration.ctl" = cluster{"Instrument":T6, "Configuration":string}
  T65 = typedef "Spectral Data.ctl" = cluster{"Intensity":dbl[], "Wavelength":dbl[], "Energy":dbl[], "Raman Shift":dbl[], "Detector Temperature":dbl}
  T66 = typedef "PlotData Config.ctl" = cluster{"Sliders":cluster{"Strain Sequence":i32, "Instrument Sequence":i32}, "Measurement":T67, "Instrument Steps":T4, "Strain Points":dbl[]}
  T67 = typedef "Measurement.ctl" = cluster{"Which Instrument?":T68, "Electrical Measurement":T69, "Measurement Mode":enum16{"Sweeping Mode", "Sampling Mode"}, "Optical Spectrum":T65}
  T68 = typedef "WhichInstrument.ctl" = enum16{"No Plot", "Spectrometer", "Parameter Analyzer", "Optoelectronic"}
  T69 = typedef "Electrical Data.ctl" = cluster{"Sequence":dbl[], "V1":dbl[], "V2":dbl[], "V3":dbl[], "V4":dbl[], "I1":dbl[], "I2":dbl[], "I3":dbl[], "I4":dbl[]}
  T70 = typedef "Instrument Sequence Config.ctl" = cluster{"Caller VI":enum16{"User", "Stress Measurement VI"}}
  T71 = typedef "Strain Measurement Config.ctl" = cluster{"Stress Sequence ":cluster{"Max Motor Position":ext, "# Intermediate Points":u32, "Initial Direction":enum16{"Tension", "Compression"}}, "Track?":bool}
  T72 = typedef "Spectrometer Refnum.ctl" = cluster{"Instrument Status":refnum<vi>, "Optical Spectrum Plot":T73, "Laser":refnum<vi>, "Filter":refnum<vi>, "Laser ON?":refnum<vi>, "Hole":refnum<vi>, "Grating":refnum<vi>, "Detector":refnum<vi>, "Acquisition Mode":refnum<vi>, "Spectal Position":refnum<vi>, "From":refnum<vi>, "To":refnum<vi>, "Integration Time":refnum<vi>, "Accumulations":refnum<vi>, "AutoScanning":refnum<vi>, "Spike Removal":refnum<vi>, "Acquisition Mode Panel":refnum<vi>}
  T73 = typedef "Optical Spectrum Plot Refnum.ctl" = cluster{"Plot List":refnum<vi>, "Optical Spectrum vs Energy":refnum<vi>, "Optical Spectrum vs Wavelength":refnum<vi>, "Optical Spectrum vs Raman Shift":refnum<vi>, "Detector Temperature":refnum<vi>}
  T74 = typedef "StressControl Refnums.ctl" = cluster{"Instrument Status":refnum<vi>, "Position":refnum<vi>, "Mecahnism Motion":refnum<vi>, "Destination":refnum<vi>, "Apply Stress":refnum<vi>, "Stop":refnum<vi>, "Stress Control VISA":refnum<vi>}
  T75 = typedef "Parameter Analyzer Refnums.ctl" = cluster{"Status":refnum<vi>, "Electrical Measurement":refnum<vi>, "Plots":T76, "HP Integration Time":refnum<vi>, "VISA":refnum<vi>, "Sweeping Time Parameters":refnum<vi>, "Acquisition Mode":refnum<vi>, "SMU 1 - Sweeping":refnum<vi>, "SMU 2 - Sweeping":refnum<vi>, "SMU 3 - Sweeping":refnum<vi>, "SMU 4 - Sweeping":refnum<vi>, "Sweep Spacing":refnum<vi>, "Range":refnum<vi>, "SMU1 - Sampling":refnum<vi>, "SMU2 - Sampling":refnum<vi>, "SMU3 - Sampling":refnum<vi>, "SMU4 - Sampling":refnum<vi>, "Sampling Time Parameters":refnum<vi>, "Stop Condition":refnum<vi>, "Instrument Status":refnum<vi>}
  T76 = typedef "Electrical Data Plot Refnums.ctl" = cluster{"Plot List":refnum<vi>, "Voltage Plot":refnum<vi>, "Current Plot":refnum<vi>, "IV Characteristic":refnum<vi>, "dI/dV-V Characteristic":refnum<vi>}
  T77 = cluster{"SMU 1 - Sweeping":cluster{"Start / Offset":dbl, "Stop / Ratio":dbl, "Step (linear only)":dbl, "Compliance":dbl, "Power Compliance":dbl, "Mode":u32, "Function":i32, "Sweep Mode":bool}, "SMU 2 - Sweeping":cluster{"Start / Offset":dbl, "Stop / Ratio":dbl, "Step (linear only)":dbl, "Compliance":dbl, "Power Compliance":dbl, "Mode":u32, "Function":i32, "Sweep Mode":bool}, "SMU 3 - Sweeping":cluster{"Start / Offset":dbl, "Stop / Ratio":dbl, "Step (linear only)":dbl, "Compliance":dbl, "Power Compliance":dbl, "Mode":u32, "Function":i32, "Sweep Mode":bool}, "SMU 4 - Sweeping":cluster{"Start / Offset":dbl, "Stop / Ratio":dbl, "Step (linear only)":dbl, "Compliance":dbl, "Power Compliance":dbl, "Mode":u32, "Function":i32, "Sweep Mode":bool}, "Sweep Spacing":u16, "Range":u16}
  T78 = cluster{"SMU1 - Sampling":cluster{"Source":dbl, "Compliance":dbl, "Mode":u32, "Function":bool}, "SMU2 - Sampling":cluster{"Source":dbl, "Compliance":dbl, "Mode":u32, "Function":bool}, "SMU3 - Sampling":cluster{"Source":dbl, "Compliance":dbl, "Mode":u32, "Function":bool}, "SMU4 - Sampling":cluster{"Source":dbl, "Compliance":dbl, "Mode":u32, "Function":bool}, "Sampling Parameters":cluster{"Initial Interval (s)":dbl, "Number of Samples":i32, "Total Sampling Time (s)":dbl, "Hold Time (s)":dbl, "Sampling Mode":i32, "Sampling Time":i32}, "Stop Condition":cluster{"Enable Delay (s)":dbl, "Name":string, "Threshold":dbl, "num. of events":i32, "Event":i32, "Stop Condition Enable":bool}}
  T79 = typedef "Switching Matrix Refnums.ctl" = cluster{"Connections":refnum<vi>, "Instrument Status":refnum<vi>}
  T80 = typedef "Instrument Sequence Refnums.ctl" = cluster{"Instrument Steps":refnum<vi>, "Instruments Status":refnum<vi>, "Device ID":refnum<vi>, "Device Information":refnum<vi>, "Pause-Resume":refnum<vi>, "Plot":T76}
  T81 = typedef "Strain Measurement Refnums.ctl" = cluster{"Instrument Steps":refnum<vi>, "Sequence Progress":refnum<vi>, "Device ID":refnum<vi>, "Device Information":refnum<vi>, "Pause-Resume":refnum<vi>, "Track":refnum<vi>, "Plot":T76}
  T82 = typedef "PlotData Refnums.ctl" = cluster{"Choose Plot":refnum<vi>, "Instrument Sequence":refnum<vi>, "Strain Sequence":refnum<vi>, "Configuration":refnum<vi>, "Electrical Data Plot":T76, "Optical Spectrum Plot":T73, "Optoelectronic Plot":cluster{"Optical Spectrum Plot":T73, "Electrical Data Plot":T76}}
  T83 = cluster{"PlotData - Instrument Sequence":i32, "PlotData - Strain Sequence":i32}
  T84 = cluster{"Start / Offset":dbl, "Stop / Ratio":dbl, "Step (linear only)":dbl, "Compliance":dbl, "Power Compliance":dbl, "Mode":u32, "Function":i32, "Sweep Mode":bool}
  T85 = cluster{"Minimum Score":sgl, "Color Score Weight":sgl, "Minimum Contrast":i32, "Match Mode":u32, "Match Feature Mode":u32, "Subpixel Accuracy":bool, "Color Sensitivity":u32, "Search Strategy":u32}
  T86 = cluster{"Max Motor Position":ext, "# Intermediate Points":u32, "Initial Direction":enum16{"Tension", "Compression"}}
  T87 = cluster{"SMU 1 - Sweeping":cluster{"Start / Offset":dbl, "Stop / Ratio":dbl, "Step \n(linear only)":dbl, "Compliance":dbl, "Power \nCompliance":dbl, "Mode":u32, "Function":i32, "Sweep Mode":bool}, "SMU 2 - Sweeping":cluster{"Start / Offset":dbl, "Stop / Ratio":dbl, "Step \n(linear only)":dbl, "Compliance":dbl, "Power \nCompliance":dbl, "Mode":u32, "Function":i32, "Sweep Mode":bool}, "SMU 3 - Sweeping":cluster{"Start / Offset":dbl, "Stop / Ratio":dbl, "Step \n(linear only)":dbl, "Compliance":dbl, "Power \nCompliance":dbl, "Mode":u32, "Function":i32, "Sweep Mode":bool}, "SMU 4 - Sweeping":cluster{"Start / Offset":dbl, "Stop / Ratio":dbl, "Step \n(linear only)":dbl, "Compliance":dbl, "Power \nCompliance":dbl, "Mode":u32, "Function":i32, "Sweep Mode":bool}, "Sweep Spacing":u16, "Range":u16}
  T88 = enum32{"invalid app kind", "Development System", "Run Time System", "Student Edition", "Embedded LabVIEW", "Evaluation", "Custom"}
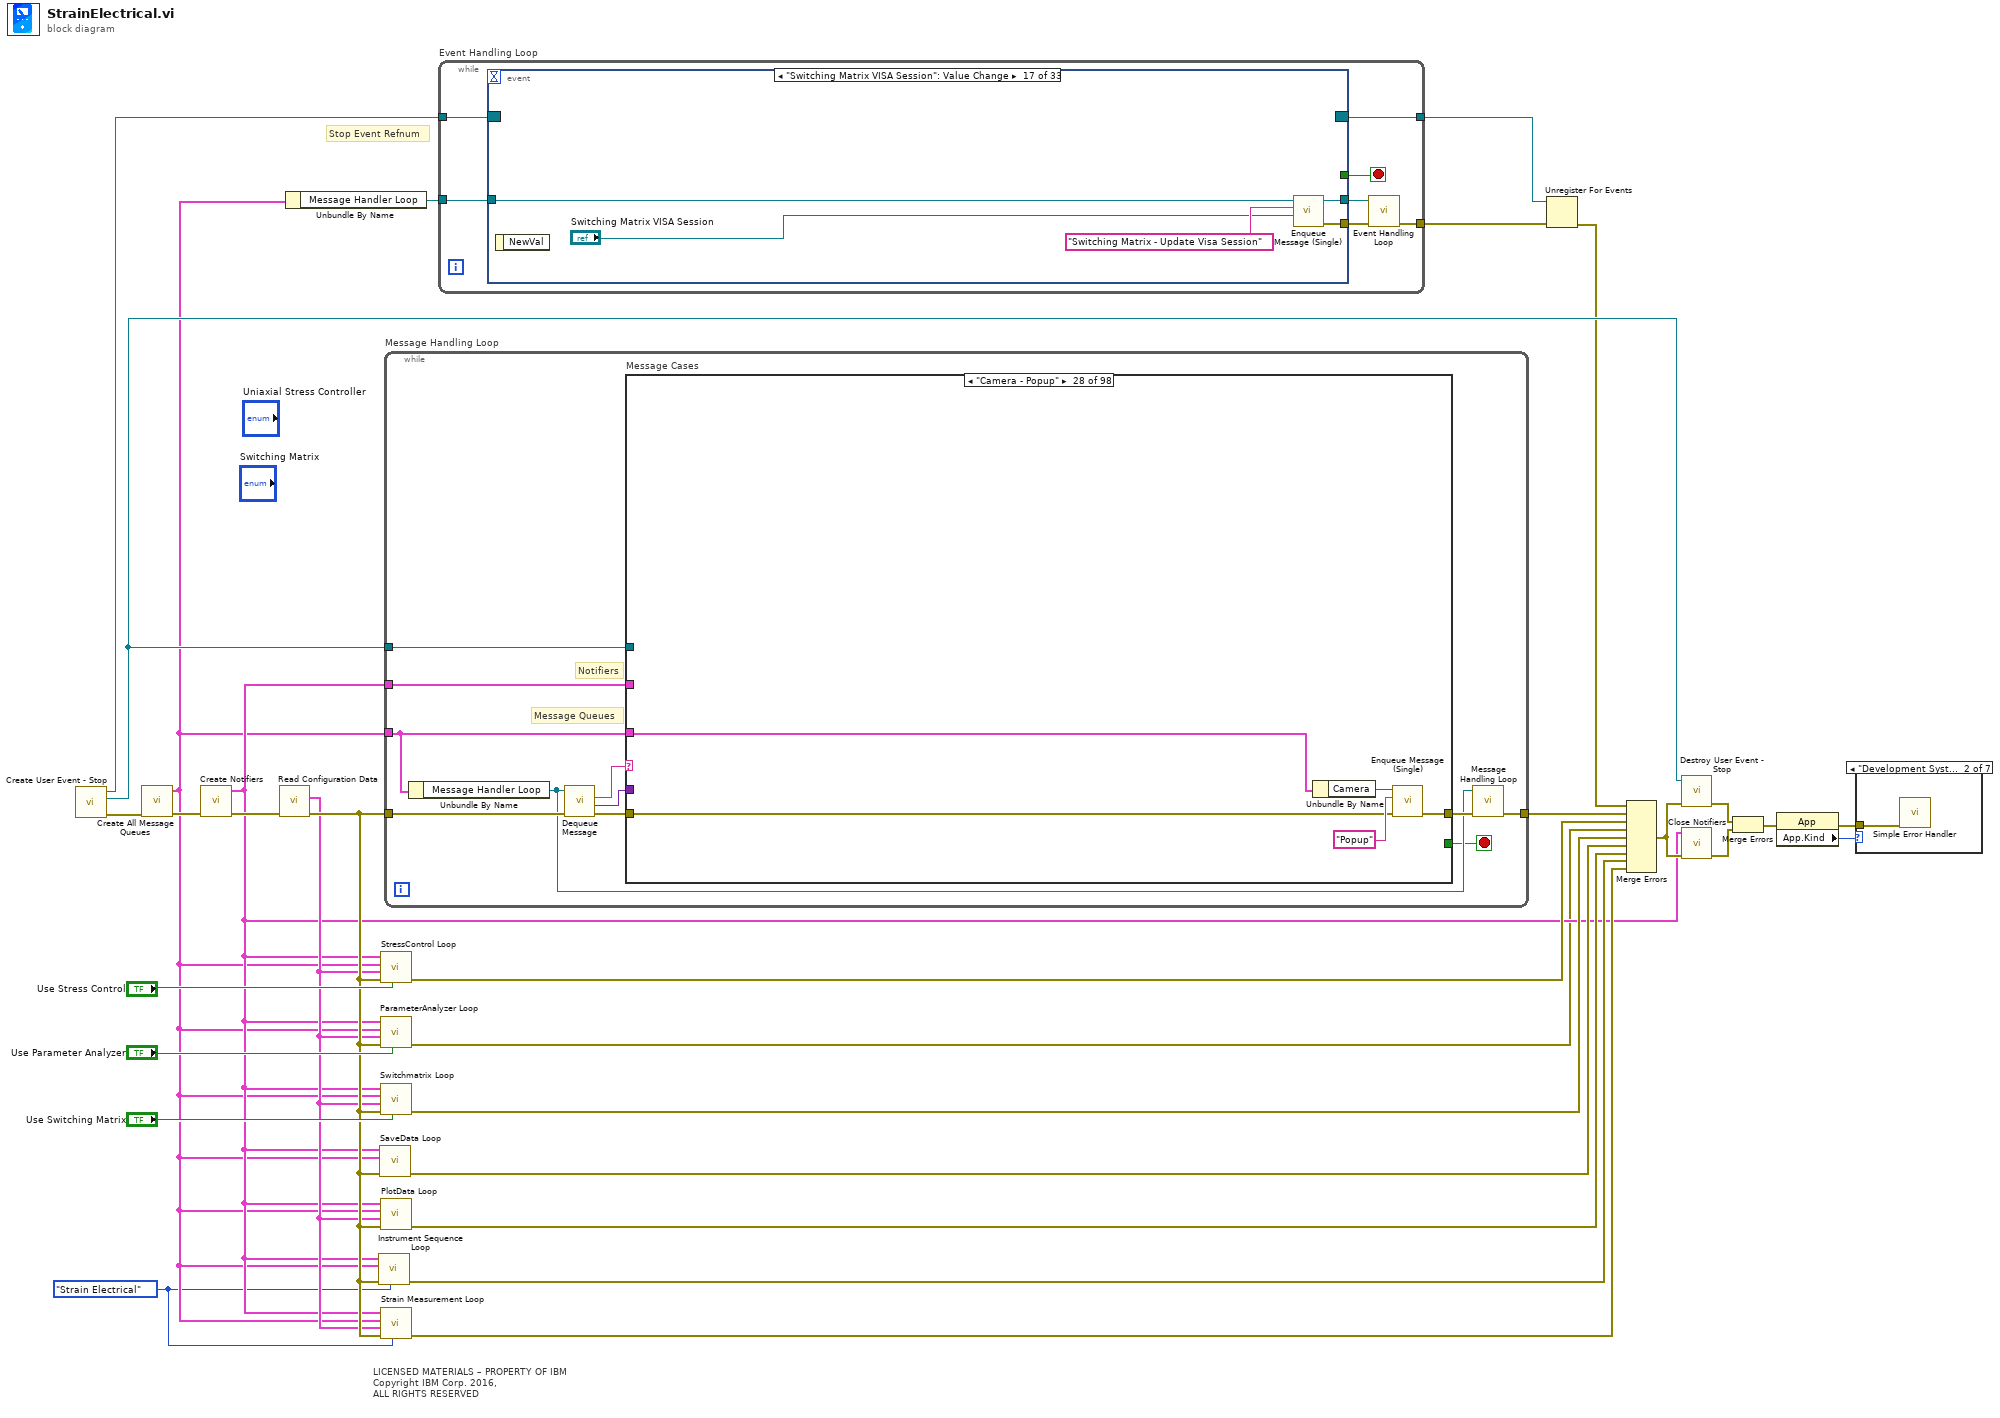
[diagram p0: block diagram]
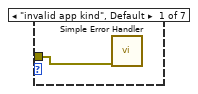
[diagram p2: hidden frame]
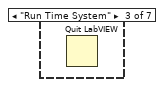
[diagram p3: hidden frame]
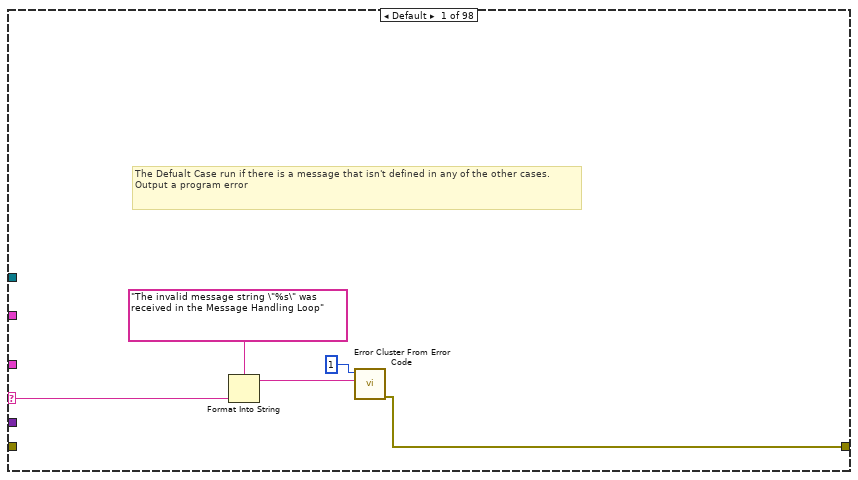
[diagram p8: hidden frame]
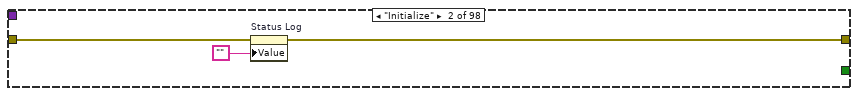
[diagram p9: hidden frame]
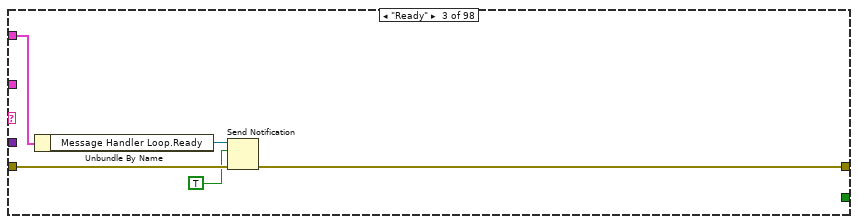
[diagram p10: hidden frame]
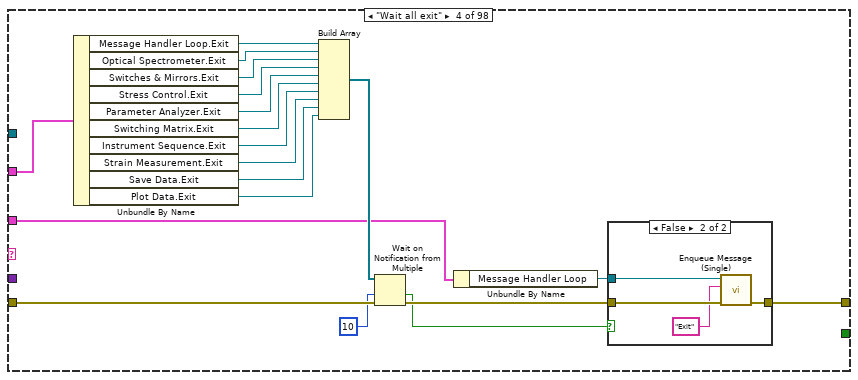
[diagram p11: hidden frame]
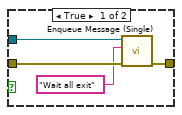
[diagram p12: hidden frame]
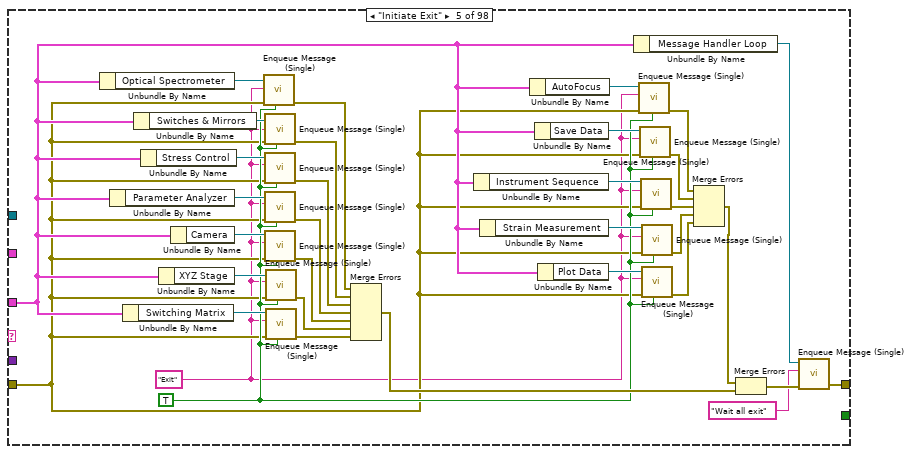
[diagram p13: hidden frame]
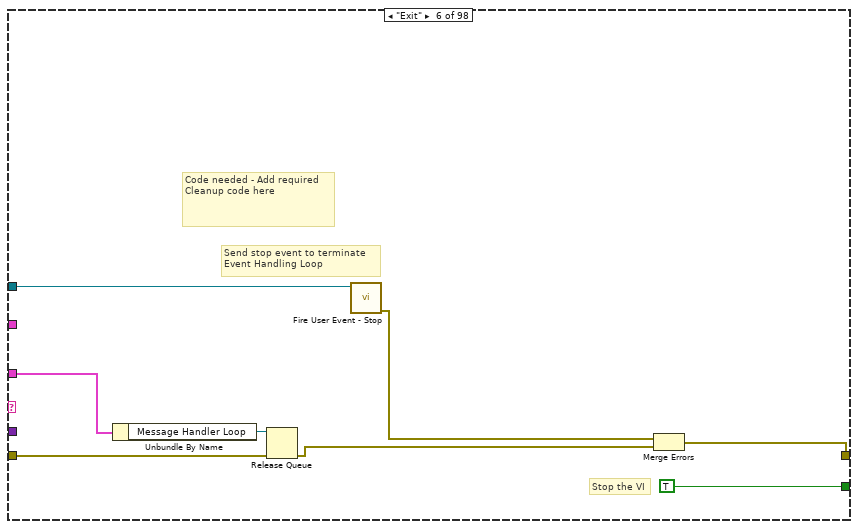
[diagram p14: hidden frame]
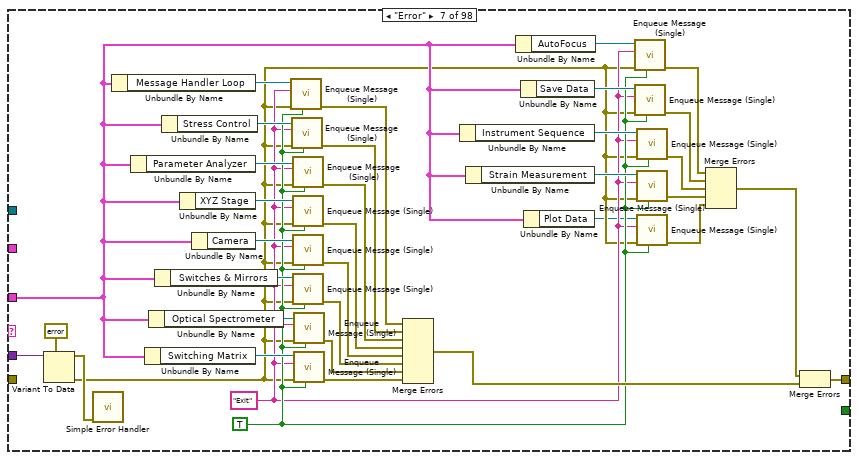
[diagram p15: hidden frame]
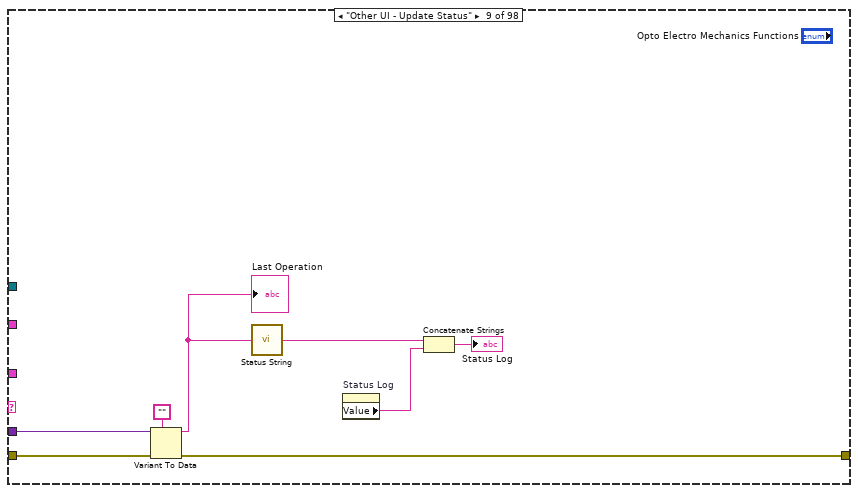
[diagram p17: hidden frame]
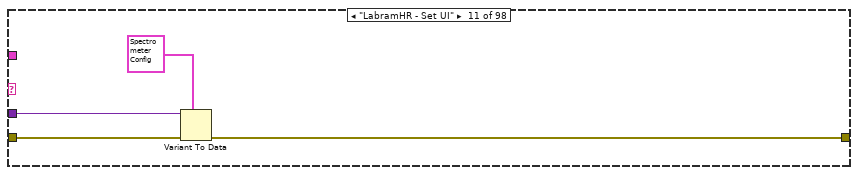
[diagram p19: hidden frame]
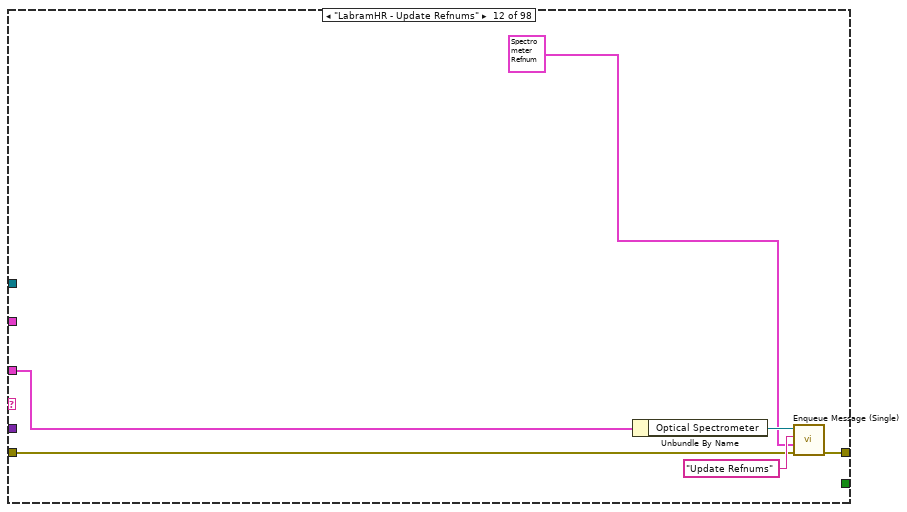
[diagram p20: hidden frame]
diagram:
  w2 = Instrument_Stequence_-_Which_Program."Strain Electrical" ("Which Program?")
  # "LICENSED MATERIALS – PROPERTY OF IBM\nCopyright IBM Corp. 2016,\nALL RIGHTS RESERVED"
  # "Stop Event Refnum"
  n1 = call "Create User Event - Stop.vi"() -> ("error out"=w24:errorcluster, "User Event - Stop"=w25:refnum<user-event>, "Stop Event Registration Refnum"=w31:refnum<event-registration>)  [unwired: 1 in, 8 out]
  n2 = call "Create All Message Queues.vi"("error in (no error)"=w24) -> ("error out"=w23:errorcluster, "Message Queues out"=w3:T18)  [unwired: 9 out]
  n3 = call "Create Notifiers.vi"("error in"=w23) -> ("error out"=w7:errorcluster, "Notifiers"=w4:T19)  [unwired: 9 out]
  n4 = call "Read Configuration Data.vi"("error in"=w7) -> ("error out"=w6:errorcluster, "System Configuration"=w5:T32)  [unwired: 9 out]
  n5 = Unbundle By Name(w3) -> ("Message Handler Loop"=w29:refnum<queue>)
  n6 = call "Instrument Sequence Loop.vi"("Which Program?"=w2, "error in"=w6, "Message Queues out"=w3, "Notifiers"=w4) -> ("error out"=w15:errorcluster)  [unwired: 1 in, 6 out]
  n7 = call "SaveData Loop.vi"("error in"=w6, "Message Queues out"=w3, "Notifiers"=w4) -> ("error out"=w17:errorcluster)  [unwired: 1 in, 7 out]
  n8 = call "StressControl Loop.vi"("Used functions"="Use Stress Control", "error in"=w6, "IBM OptoElectroMechanics Configuration"=w5, "Message Queues out"=w3, "Notifiers"=w4) -> ("error out"=w20:errorcluster)  [unwired: 6 out]
  n9 = call "ParameterAnalyzer Loop.vi"("Used functions"="Use Parameter Analyzer", "error in"=w6, "IBM OptoElectroMechanics Configuration"=w5, "Message Queues out"=w3, "Notifiers"=w4) -> ("error out"=w1:errorcluster)  [unwired: 6 out]
  n10 = call "Switchmatrix Loop.vi"("Used functions"="Use Switching Matrix", "error in"=w6, "IBM OptoElectroMechanics Configuration"=w5, "Message Queues out"=w3, "Notifiers"=w4) -> ("error out"=w18:errorcluster)  [unwired: 6 out]
  n11 = call "PlotData Loop.vi"("error in"=w6, "IBM OptoElectroMechanics Configuration"=w5, "Message Queues"=w3, "Notifiers"=w4) -> ("error out"=w16:errorcluster)  [unwired: 7 out]
  n12 = call "Strain Measurement Loop.vi"("Which Program?"=w2, "error in"=w6, "IBM OptoElectroMechanics Configuration"=w5, "Message Queues out"=w3, "Notifiers"=w4) -> ("error out"=w19:errorcluster)  [unwired: 6 out]
  n13 = while "Message Handling Loop" {
    tunnel: w6 -> [w42]
    tunnel: [w39] -> w21
    tunnel: w3 -> [w33]
    tunnel: w25 -> [w35]
    tunnel: w4 -> [w32]
    stop <- w34 stop-if-true
    # "Notifiers"
    # "Message Queues"
    n14 = Unbundle By Name(w33) -> ("Message Handler Loop"=w38:refnum<queue>)
    n15 = call "Dequeue Message.vi"("error in (no error)"=w42, "Message Queue"=w38) -> ("error out"=w41:errorcluster, "Message Data"=w36:variant, "Message"=w37:string)  [unwired: 7 out]
    n16 = case "Message Cases" shown="\"Camera - Popup\"" w37 {
      selector: w37 -> [w47 _ _ _ _ _ _ _ _ _ _ _ _ _ _ _ _ _ _ _ _ _ _ _ _ _ _ _ _ _ _ _ _ _ _ _ _ _ _ _ _ _ _ _ _ _ _ _ _ _ _ _ _ _ _ _ _ _ _ _ _ _ _ _ _ _ _ _ _ _ _ _ _ _ _ _ _ _ _ _ _ _ _ _ _ _ _ _ _ _ _ _ _ _ _ _ _ _]
      tunnel: w41 -> [_ w49 w54 w73 w86 w123 _ w161 w169 w170 w174 w176 w186 w201 w212 w223 w234 w245 w256 w260 w265 w267 w275 w288 w299 w301 w311 w313 w318 w323 w328 w334 w347 w361 w372 w383 w394 w395 w400 w421 w425 w436 w446 w472 w485 w502 w519 w523 w528 w533 w540 w548 w557 w568 w572 w577 w582 w593 w604 w605 w616 w627 w638 w639 w644 w649 w654 w659 w664 w669 w674 w679 w687 w693 w698 w703 w708 w713 w716 w721 w726 w731 w737 w746 w760 w765 w770 w775 w778 w783 w788 w793 w798 w801 w808 w821 w837 w838]
      tunnel: [w43 w48 w55 w62 w102 w124 w158 w161 w166 w170 w173 w176 w184 w197 w208 w220 w231 w241 w254 w257 w262 w267 w278 w287 w298 w301 w310 w317 w322 w327 w328 w333 w346 w360 w371 w382 w393 w399 w400 w418 w424 w430 w445 w469 w480 w491 w511 w525 w530 w533 w537 w551 w560 w571 w576 w581 w582 w588 w600 w605 w611 w622 w633 w642 w647 w652 w657 w662 w667 w672 w677 w679 w688 w692 w697 w702 w707 w712 w718 w723 w728 w731 w736 w745 w757 w764 w769 w774 w777 w782 w787 w792 w797 w801 w807 w824 w832 w838] -> w40
      tunnel: w36 -> [_ _ _ _ _ _ w160 _ w168 _ w172 _ w190 w200 w211 w222 w233 w244 w255 _ _ _ w271 w289 w300 _ w312 _ _ _ _ w332 _ w354 w366 w377 w388 _ _ w417 w423 w435 _ w471 w484 w501 w518 _ _ _ w536 w545 _ w565 _ _ _ w592 w603 _ w615 w626 w637 _ _ _ _ _ _ _ _ _ _ _ _ _ _ _ _ _ _ _ w735 _ w759 _ _ _ _ _ _ _ _ _ w806 _ w836 _]
      tunnel: w35 -> [_ _ _ _ _ w121 _ _ _ _ _ _ _ _ _ _ _ _ _ _ _ _ _ _ _ _ _ _ _ _ _ _ _ _ _ _ _ _ _ _ _ _ _ _ _ _ _ _ _ _ _ _ _ _ _ _ _ _ _ _ _ _ _ _ _ _ _ _ _ _ _ _ _ _ _ _ _ _ _ _ _ _ _ _ _ _ _ _ _ _ _ _ _ _ _ _ _ _]
      tunnel: [_ _ _ _ _ TRUE _ _ _ _ _ _ _ _ _ _ _ _ _ _ _ _ _ _ _ _ _ _ _ _ _ _ _ _ _ _ _ _ _ _ _ _ _ _ _ _ _ _ _ _ _ _ _ _ _ _ _ _ _ _ _ _ _ _ _ _ _ _ _ _ _ _ _ _ _ _ _ _ _ _ _ _ _ _ _ _ _ _ _ _ _ _ _ _ _ _ _ _] -> w34
      tunnel: w33 -> [_ _ _ w61 w89 w118 w131 _ _ _ _ w179 w189 w196 w205 w218 w229 w238 w250 w258 w263 _ w276 w284 w295 _ w308 w315 w320 w325 _ _ w343 w357 w368 w379 w390 w397 _ _ _ w432 w447 w465 w479 w490 w510 w524 w529 _ _ w549 w558 w569 w574 w579 _ w587 w599 _ w610 w621 w632 w641 w646 w651 w656 w661 w666 w671 w676 _ w686 w695 w700 w705 w710 w715 w720 w725 w730 _ _ w747 w754 w761 w766 w771 w780 w785 w790 w795 w800 _ _ w822 w831 _]
      tunnel: w32 -> [_ _ w53 w74 _ _ _ _ _ _ _ _ _ _ _ _ _ _ _ _ _ _ _ _ _ _ _ _ _ _ _ _ _ _ _ _ _ _ _ _ _ _ _ _ _ _ _ _ _ _ _ _ _ _ _ _ _ _ _ _ _ _ _ _ _ _ _ _ _ _ _ _ _ _ _ _ _ _ _ _ _ _ _ _ _ _ _ _ _ _ _ _ _ _ _ _ _ _]
      frame Default {
        # "The Defualt Case run if there is a message that isn't defined in any of the other cases.\nOutput a program error"
        n17 = Format Into String(format string="The invalid message string \"%s\" was  received in the Message Handling Loop", w47) -> (resulting string=w45:string)  [unwired: 2 in, 1 out]
        n18 = call <vilib>:"Error Cluster From Error Code.vi"("error message (\"\")"=w45, "error code (0)"=1) -> ("error out"=w43:errorcluster)  [unwired: 2 in, 5 out]
      }
      frame "Initialize" {
        n19 = property on="Status Log" class="Str"(error in=w49, "Value"="") -> (error out=w48:errorcluster)  [unwired: 1 in, 1 out]
      }
      frame "Ready" {
        n20 = Unbundle By Name(w53) -> ("Message Handler Loop.Ready"=w52:refnum<notifier>)
        n21 = Send Notification(notification=TRUE, notifier=w52, error in (no error)=w54) -> (error out=w55:errorcluster)  [unwired: 1 out]
      }
      frame "Wait all exit" {
        n22 = Unbundle By Name(w74) -> ("Message Handler Loop.Exit"=w71:refnum<notifier>, "Optical Spectrometer.Exit"=w70:refnum<notifier>, "Switches & Mirrors.Exit"=w69:refnum<notifier>, "Stress Control.Exit"=w68:refnum<notifier>, "Parameter Analyzer.Exit"=w67:refnum<notifier>, "Switching Matrix.Exit"=w66:refnum<notifier>, "Instrument Sequence.Exit"=w59:refnum<notifier>, "Strain Measurement.Exit"=w58:refnum<notifier>, "Save Data.Exit"=w57:refnum<notifier>, "Plot Data.Exit"=w56:refnum<notifier>)
        n23 = Build Array(w71, w70, w69, w68, w67, w66, w59, w58, w57, w56) -> (w65:refnum<notifier>[])
        n24 = Wait on Notification from Multiple(0:w65, 2:10 ("timeout in ms (-1)"), 3:w73) -> (10:w60:bool, 11:w63:errorcluster)  [unwired: 3 out]
        n25 = Unbundle By Name(w61) -> ("Message Handler Loop"=w64:refnum<queue>)
        n26 = case shown="False" w60 {
          tunnel: w64 -> [w78 w82]
          tunnel: w63 -> [w77 w81]
          tunnel: [w76 w80] -> w62
          frame True {
            n27 = call "Enqueue Message (Single).vi"("error in (no error)"=w77, "Message"="Wait all exit", "Message Queue"=w78) -> ("error out"=w76:errorcluster)  [unwired: 1 in, 7 out]
          }
          frame False {
            n28 = call "Enqueue Message (Single).vi"("error in (no error)"=w81, "Message"="Exit", "Message Queue"=w82) -> ("error out"=w80:errorcluster)  [unwired: 1 in, 7 out]
          }
        }
      }
      frame "Initiate Exit" {
        w87 = TRUE ("Priority Message? (F)")
        w84 = "Exit" ("Message")
        n29 = Unbundle By Name(w89) -> ("Optical Spectrometer"=w106:refnum<queue>)
        n30 = Unbundle By Name(w89) -> ("Parameter Analyzer"=w103:refnum<queue>)
        n31 = Unbundle By Name(w89) -> ("Switching Matrix"=w98:refnum<queue>)
        n32 = Unbundle By Name(w89) -> ("Switches & Mirrors"=w105:refnum<queue>)
        n33 = Unbundle By Name(w89) -> ("Stress Control"=w104:refnum<queue>)
        n34 = Unbundle By Name(w89) -> ("XYZ Stage"=w116:refnum<queue>)
        n35 = Unbundle By Name(w89) -> ("Camera"=w107:refnum<queue>)
        n36 = call "Enqueue Message (Single).vi"("Priority Message? (F)"=w87, "error in (no error)"=w86, "Message"=w84, "Message Queue"=w106) -> ("error out"=w108:errorcluster)  [unwired: 1 in, 6 out]
        n37 = call "Enqueue Message (Single).vi"("Priority Message? (F)"=w87, "error in (no error)"=w86, "Message"=w84, "Message Queue"=w105) -> ("error out"=w109:errorcluster)  [unwired: 1 in, 6 out]
        n38 = call "Enqueue Message (Single).vi"("Priority Message? (F)"=w87, "error in (no error)"=w86, "Message"=w84, "Message Queue"=w104) -> ("error out"=w110:errorcluster)  [unwired: 1 in, 6 out]
        n39 = call "Enqueue Message (Single).vi"("Priority Message? (F)"=w87, "error in (no error)"=w86, "Message"=w84, "Message Queue"=w103) -> ("error out"=w111:errorcluster)  [unwired: 1 in, 6 out]
        n40 = call "Enqueue Message (Single).vi"("Priority Message? (F)"=w87, "error in (no error)"=w86, "Message"=w84, "Message Queue"=w107) -> ("error out"=w112:errorcluster)  [unwired: 1 in, 6 out]
        n41 = call "Enqueue Message (Single).vi"("Priority Message? (F)"=w87, "error in (no error)"=w86, "Message"=w84, "Message Queue"=w116) -> ("error out"=w113:errorcluster)  [unwired: 1 in, 6 out]
        n42 = call "Enqueue Message (Single).vi"("Priority Message? (F)"=w87, "error in (no error)"=w86, "Message"=w84, "Message Queue"=w98) -> ("error out"=w114:errorcluster)  [unwired: 1 in, 6 out]
        n43 = Merge Errors(w108, w109, w110, w111, w112, w113, w114) -> (w115:errorcluster)
        n44 = Unbundle By Name(w89) -> ("Instrument Sequence"=w95:refnum<queue>)
        n45 = Unbundle By Name(w89) -> ("Strain Measurement"=w91:refnum<queue>)
        n46 = Unbundle By Name(w89) -> ("AutoFocus"=w97:refnum<queue>)
        n47 = Unbundle By Name(w89) -> ("Save Data"=w96:refnum<queue>)
        n48 = Unbundle By Name(w89) -> ("Plot Data"=w88:refnum<queue>)
        n49 = Unbundle By Name(w89) -> ("Message Handler Loop"=w100:refnum<queue>)
        n50 = call "Enqueue Message (Single).vi"("Priority Message? (F)"=w87, "error in (no error)"=w86, "Message"=w84, "Message Queue"=w97) -> ("error out"=w94:errorcluster)  [unwired: 1 in, 6 out]
        n51 = call "Enqueue Message (Single).vi"("Priority Message? (F)"=w87, "error in (no error)"=w86, "Message"=w84, "Message Queue"=w96) -> ("error out"=w93:errorcluster)  [unwired: 1 in, 6 out]
        n52 = call "Enqueue Message (Single).vi"("Priority Message? (F)"=w87, "error in (no error)"=w86, "Message"=w84, "Message Queue"=w95) -> ("error out"=w92:errorcluster)  [unwired: 1 in, 6 out]
        n53 = call "Enqueue Message (Single).vi"("Priority Message? (F)"=w87, "error in (no error)"=w86, "Message"=w84, "Message Queue"=w91) -> ("error out"=w90:errorcluster)  [unwired: 1 in, 6 out]
        n54 = call "Enqueue Message (Single).vi"("Priority Message? (F)"=w87, "error in (no error)"=w86, "Message"=w84, "Message Queue"=w88) -> ("error out"=w85:errorcluster)  [unwired: 1 in, 6 out]
        n55 = Merge Errors(w94, w93, w92, w90, w85) -> (w83:errorcluster)
        n56 = Merge Errors(w83, w115) -> (w101:errorcluster)
        n57 = call "Enqueue Message (Single).vi"("error in (no error)"=w101, "Message"="Wait all exit", "Message Queue"=w100) -> ("error out"=w102:errorcluster)  [unwired: 1 in, 7 out]
      }
      frame "Exit" {
        # "Send stop event to terminate \nEvent Handling Loop"
        # "Stop the VI"
        # "Code needed - Add required Cleanup code here"
        n58 = Unbundle By Name(w118) -> ("Message Handler Loop"=w117:refnum<queue>)
        n59 = Release Queue(queue=w117, error in (no error)=w123) -> (error out=w122:errorcluster)  [unwired: 3 out]
        n60 = call "Fire User Event - Stop.vi"("User Event - Stop"=w121) -> ("error out"=w120:errorcluster)  [unwired: 1 in, 9 out]
        n61 = Merge Errors(w120, w122) -> (w124:errorcluster)
      }
      frame "Error" {
        w130 = TRUE ("Priority Message? (F)")
        w129 = "Exit" ("Message")
        n62 = Variant To Data(type=errorcluster {"status"=FALSE, "code"=0, "source"=""} ("error out"), Variant=w160) -> (data=w157:errorcluster, error out=w127:errorcluster)  [unwired: 1 in]
        n63 = call <vilib>:"Simple Error Handler.vi"("error in (no error)"=w157) -> ()  [unwired: 1 in, 8 out]
        n64 = Unbundle By Name(w131) -> ("Message Handler Loop"=w141:refnum<queue>)
        n65 = Unbundle By Name(w131) -> ("Parameter Analyzer"=w155:refnum<queue>)
        n66 = Unbundle By Name(w131) -> ("Switching Matrix"=w150:refnum<queue>)
        n67 = Unbundle By Name(w131) -> ("Optical Spectrometer"=w151:refnum<queue>)
        n68 = Unbundle By Name(w131) -> ("Switches & Mirrors"=w142:refnum<queue>)
        n69 = Unbundle By Name(w131) -> ("Stress Control"=w154:refnum<queue>)
        n70 = Unbundle By Name(w131) -> ("XYZ Stage"=w156:refnum<queue>)
        n71 = Unbundle By Name(w131) -> ("Camera"=w143:refnum<queue>)
        n72 = call "Enqueue Message (Single).vi"("Priority Message? (F)"=w130, "error in (no error)"=w127, "Message"=w129, "Message Queue"=w141) -> ("error out"=w140:errorcluster)  [unwired: 1 in, 6 out]
        n73 = call "Enqueue Message (Single).vi"("Priority Message? (F)"=w130, "error in (no error)"=w127, "Message"=w129, "Message Queue"=w154) -> ("error out"=w149:errorcluster)  [unwired: 1 in, 6 out]
        n74 = call "Enqueue Message (Single).vi"("Priority Message? (F)"=w130, "error in (no error)"=w127, "Message"=w129, "Message Queue"=w155) -> ("error out"=w148:errorcluster)  [unwired: 1 in, 6 out]
        n75 = call "Enqueue Message (Single).vi"("Priority Message? (F)"=w130, "error in (no error)"=w127, "Message"=w129, "Message Queue"=w156) -> ("error out"=w147:errorcluster)  [unwired: 1 in, 6 out]
        n76 = call "Enqueue Message (Single).vi"("Priority Message? (F)"=w130, "error in (no error)"=w127, "Message"=w129, "Message Queue"=w143) -> ("error out"=w146:errorcluster)  [unwired: 1 in, 6 out]
        n77 = call "Enqueue Message (Single).vi"("Priority Message? (F)"=w130, "error in (no error)"=w127, "Message"=w129, "Message Queue"=w142) -> ("error out"=w145:errorcluster)  [unwired: 1 in, 6 out]
        n78 = call "Enqueue Message (Single).vi"("Priority Message? (F)"=w130, "error in (no error)"=w127, "Message"=w129, "Message Queue"=w151) -> ("error out"=w153:errorcluster)  [unwired: 1 in, 6 out]
        n79 = call "Enqueue Message (Single).vi"("Priority Message? (F)"=w130, "error in (no error)"=w127, "Message"=w129, "Message Queue"=w150) -> ("error out"=w152:errorcluster)  [unwired: 1 in, 6 out]
        n80 = Merge Errors(w140, w149, w148, w147, w146, w145, w153, w152) -> (w144:errorcluster)
        n81 = Unbundle By Name(w131) -> ("Instrument Sequence"=w137:refnum<queue>)
        n82 = Unbundle By Name(w131) -> ("Strain Measurement"=w133:refnum<queue>)
        n83 = Unbundle By Name(w131) -> ("AutoFocus"=w139:refnum<queue>)
        n84 = Unbundle By Name(w131) -> ("Save Data"=w138:refnum<queue>)
        n85 = Unbundle By Name(w131) -> ("Plot Data"=w126:refnum<queue>)
        n86 = call "Enqueue Message (Single).vi"("Priority Message? (F)"=w130, "error in (no error)"=w127, "Message"=w129, "Message Queue"=w139) -> ("error out"=w134:errorcluster)  [unwired: 1 in, 6 out]
        n87 = call "Enqueue Message (Single).vi"("Priority Message? (F)"=w130, "error in (no error)"=w127, "Message"=w129, "Message Queue"=w138) -> ("error out"=w135:errorcluster)  [unwired: 1 in, 6 out]
        n88 = call "Enqueue Message (Single).vi"("Priority Message? (F)"=w130, "error in (no error)"=w127, "Message"=w129, "Message Queue"=w137) -> ("error out"=w136:errorcluster)  [unwired: 1 in, 6 out]
        n89 = call "Enqueue Message (Single).vi"("Priority Message? (F)"=w130, "error in (no error)"=w127, "Message"=w129, "Message Queue"=w133) -> ("error out"=w132:errorcluster)  [unwired: 1 in, 6 out]
        n90 = call "Enqueue Message (Single).vi"("Priority Message? (F)"=w130, "error in (no error)"=w127, "Message"=w129, "Message Queue"=w126) -> ("error out"=w128:errorcluster)  [unwired: 1 in, 6 out]
        n91 = Merge Errors(w134, w135, w136, w132, w128) -> (w125:errorcluster)
        n92 = Merge Errors(w125, w144) -> (w158:errorcluster)
      }
      frame "----- Other UI Events -----" {
        # "Other UI Events"
      }
      frame "Other UI - Update Status" {
        n93 = Variant To Data(error in=w169, type="", Variant=w168) -> (data=w162:string, error out=w166:errorcluster)
        "Last Operation" <- w162
        n94 = call "Status String.vi"("Message"=w162) -> ("Status String"=w165:string)
        n95 = property on="Status Log" class="Str"() -> ("Value"=w163:string)  [unwired: 2 in, 2 out]
        n96 = Concatenate Strings(w165, w163) -> (→"Status Log":string)
      }
      frame "----- Labram HR Events -----" {
        # "Labram HR Events"
      }
      frame "LabramHR - Set UI" {
        n97 = Variant To Data(error in=w174, type=T43 {"Laser Settings"={"Laser Wavelength"=enum."633 nm", "Neutral Density Filter"=enum."1%"}, "Spectrometer Settings"={"Confocal Hole Size (µm)"=150.0, "Grating"=1, "Detector"=enum."InGaAs Array"}, "Acquisition Settings"={"Acquisition Mode"=enum."Single Window", "Spectal Position (nm)"=480.0, "From (nm)"=632.0, "To (nm)"=1000.0, "Integration Time (s)"=3.0, "Number of Accumulations"=3, "AutoScanning"=FALSE, "Spike Removal"=FALSE}, "Path"=path ""} ("LabramHR"), Variant=w172) -> (error out=w173:errorcluster)  [unwired: 1 out]
      }
      frame "LabramHR - Update Refnums" {
        n98 = Unbundle By Name(w179) -> ("Optical Spectrometer"=w177:refnum<queue>)
        n99 = call "Enqueue Message (Single).vi"("Message Data"=T72 {"Instrument Status"=refnum, "Optical Spectrum Plot"={"Plot List"=refnum, "Optical Spectrum vs Energy"=refnum, "Optical Spectrum vs Wavelength"=refnum, "Optical Spectrum vs Raman Shift"=refnum, "Detector Temperature"=refnum}, "Laser"=refnum, "Filter"=refnum, "Laser ON?"=refnum, "Hole"=refnum, "Grating"=refnum, "Detector"=refnum, "Acquisition Mode"=refnum, "Spectal Position"=refnum, "From"=refnum, "To"=refnum, "Integration Time"=refnum, "Accumulations"=refnum, "AutoScanning"=refnum, "Spike Removal"=refnum, "Acquisition Mode Panel"=refnum} ("LabramHR"), "Message"="Update Refnums", "Message Queue"=w177) -> ()  [unwired: 1 in, 8 out]
      }
      frame "LabramHR - Set Laser" {
        # "Handle the change of Excitation Wavelength"
        n100 = Variant To Data(error in=w186, type=Laser."633 nm" ("NewVal"), Variant=w190) -> (data=w181:T45, error out=w185:errorcluster)
        n101 = Bundle By Name(cluster=T43 {"Laser Settings"={"Laser Wavelength"=enum."633 nm", "Neutral Density Filter"=enum."1%"}, "Spectrometer Settings"={"Confocal Hole Size (µm)"=150.0, "Grating"=1, "Detector"=enum."InGaAs Array"}, "Acquisition Settings"={"Acquisition Mode"=enum."Single Window", "Spectal Position (nm)"=480.0, "From (nm)"=632.0, "To (nm)"=1000.0, "Integration Time (s)"=3.0, "Number of Accumulations"=3, "AutoScanning"=FALSE, "Spike Removal"=FALSE}, "Path"=path ""} ("LabramHR"), "Laser Settings.Laser Wavelength"=w181) -> (w183:T43)
        n102 = Unbundle By Name(w189) -> ("Optical Spectrometer"=w188:refnum<queue>)
        n103 = call "Enqueue Message (Single).vi"("error in (no error)"=w185, "Message Data"=w183, "Message"="Set Laser", "Message Queue"=w188) -> ("error out"=w184:errorcluster)  [unwired: 7 out]
      }
      frame "LabramHR - Set Filter" {
        # "Handle the change of Neutral Density Filter"
        n104 = Variant To Data(error in=w201, type=Filter."1%" ("NewVal"), Variant=w200) -> (data=w192:T46, error out=w198:errorcluster)
        n105 = Bundle By Name(cluster=T43 {"Laser Settings"={"Laser Wavelength"=enum."633 nm", "Neutral Density Filter"=enum."1%"}, "Spectrometer Settings"={"Confocal Hole Size (µm)"=150.0, "Grating"=1, "Detector"=enum."InGaAs Array"}, "Acquisition Settings"={"Acquisition Mode"=enum."Single Window", "Spectal Position (nm)"=480.0, "From (nm)"=632.0, "To (nm)"=1000.0, "Integration Time (s)"=3.0, "Number of Accumulations"=3, "AutoScanning"=FALSE, "Spike Removal"=FALSE}, "Path"=path ""} ("LabramHR"), "Laser Settings.Neutral Density Filter"=w192) -> (w194:T43)
        n106 = Unbundle By Name(w196) -> ("Optical Spectrometer"=w199:refnum<queue>)
        n107 = call "Enqueue Message (Single).vi"("error in (no error)"=w198, "Message Data"=w194, "Message"="Set Filter", "Message Queue"=w199) -> ("error out"=w197:errorcluster)  [unwired: 7 out]
      }
      frame "LabramHR - Set Hole" {
        # "Handle the change in Confocal hole size"
        n108 = Variant To Data(error in=w212, type=150.0 ("Confocal Hole Size (µm) 2"), Variant=w211) -> (data=w204:dbl, error out=w207:errorcluster)
        n109 = Bundle By Name(cluster=T43 {"Laser Settings"={"Laser Wavelength"=enum."633 nm", "Neutral Density Filter"=enum."1%"}, "Spectrometer Settings"={"Confocal Hole Size (µm)"=150.0, "Grating"=1, "Detector"=enum."InGaAs Array"}, "Acquisition Settings"={"Acquisition Mode"=enum."Single Window", "Spectal Position (nm)"=480.0, "From (nm)"=632.0, "To (nm)"=1000.0, "Integration Time (s)"=3.0, "Number of Accumulations"=3, "AutoScanning"=FALSE, "Spike Removal"=FALSE}, "Path"=path ""} ("LabramHR"), "Spectrometer Settings.Confocal Hole Size (µm)"=w204) -> (w203:T43)
        n110 = Unbundle By Name(w205) -> ("Optical Spectrometer"=w209:refnum<queue>)
        n111 = call "Enqueue Message (Single).vi"("error in (no error)"=w207, "Message Data"=w203, "Message"="Set Hole", "Message Queue"=w209) -> ("error out"=w208:errorcluster)  [unwired: 7 out]
      }
      frame "LabramHR - Set Grating" {
        w214 = T48 1 items=["1800 l/mm", "150 l/mm"] ("NewVal")
        # "Handle the change of grating"
        n112 = Variant To Data(error in=w223, type=w214, Variant=w222) -> (data=w216:T48, error out=w219:errorcluster)
        n113 = Bundle By Name(cluster=T43 {"Laser Settings"={"Laser Wavelength"=enum."633 nm", "Neutral Density Filter"=enum."1%"}, "Spectrometer Settings"={"Confocal Hole Size (µm)"=150.0, "Grating"=1, "Detector"=enum."InGaAs Array"}, "Acquisition Settings"={"Acquisition Mode"=enum."Single Window", "Spectal Position (nm)"=480.0, "From (nm)"=632.0, "To (nm)"=1000.0, "Integration Time (s)"=3.0, "Number of Accumulations"=3, "AutoScanning"=FALSE, "Spike Removal"=FALSE}, "Path"=path ""} ("LabramHR"), "Spectrometer Settings.Grating"=w216) -> (w215:T43)
        n114 = Unbundle By Name(w218) -> ("Optical Spectrometer"=w221:refnum<queue>)
        n115 = call "Enqueue Message (Single).vi"("error in (no error)"=w219, "Message Data"=w215, "Message"="Set Grating", "Message Queue"=w221) -> ("error out"=w220:errorcluster)  [unwired: 7 out]
      }
      frame "LabramHR - Set Detector" {
        # "Handle the change of grating"
        n116 = Variant To Data(error in=w234, type=Detector."Silicon CCD" ("NewVal"), Variant=w233) -> (data=w227:T49, error out=w230:errorcluster)
        n117 = Bundle By Name(cluster=T43 {"Laser Settings"={"Laser Wavelength"=enum."633 nm", "Neutral Density Filter"=enum."1%"}, "Spectrometer Settings"={"Confocal Hole Size (µm)"=150.0, "Grating"=1, "Detector"=enum."InGaAs Array"}, "Acquisition Settings"={"Acquisition Mode"=enum."Single Window", "Spectal Position (nm)"=480.0, "From (nm)"=632.0, "To (nm)"=1000.0, "Integration Time (s)"=3.0, "Number of Accumulations"=3, "AutoScanning"=FALSE, "Spike Removal"=FALSE}, "Path"=path ""} ("LabramHR"), "Spectrometer Settings.Detector"=w227) -> (w226:T43)
        n118 = Unbundle By Name(w229) -> ("Optical Spectrometer"=w232:refnum<queue>)
        n119 = call "Enqueue Message (Single).vi"("error in (no error)"=w230, "Message Data"=w226, "Message"="Set Detector", "Message Queue"=w232) -> ("error out"=w231:errorcluster)  [unwired: 7 out]
      }
      frame "LabramHR - Set Spectal Position" {
        # "Handle the change of Spetrometer position"
        n120 = Variant To Data(error in=w245, type=480.0 ("Spectal Position (nm) 2"), Variant=w244) -> (data=w237:dbl, error out=w239:errorcluster)
        n121 = Bundle By Name(cluster=T43 {"Laser Settings"={"Laser Wavelength"=enum."633 nm", "Neutral Density Filter"=enum."1%"}, "Spectrometer Settings"={"Confocal Hole Size (µm)"=150.0, "Grating"=1, "Detector"=enum."InGaAs Array"}, "Acquisition Settings"={"Acquisition Mode"=enum."Single Window", "Spectal Position (nm)"=480.0, "From (nm)"=632.0, "To (nm)"=1000.0, "Integration Time (s)"=3.0, "Number of Accumulations"=3, "AutoScanning"=FALSE, "Spike Removal"=FALSE}, "Path"=path ""} ("LabramHR"), "Acquisition Settings.Spectal Position (nm)"=w237) -> (w236:T43)
        n122 = Unbundle By Name(w238) -> ("Optical Spectrometer"=w242:refnum<queue>)
        n123 = call "Enqueue Message (Single).vi"("error in (no error)"=w239, "Message Data"=w236, "Message"="Set Spectal Position", "Message Queue"=w242) -> ("error out"=w241:errorcluster)  [unwired: 7 out]
      }
      frame "LabramHR - Set Acquisition Settings" {
        # "Handle the change of integration time"
        n124 = Variant To Data(error in=w256, type=T50 {"Acquisition Mode"=enum."Single Window", "Spectal Position (nm)"=480.0, "From (nm)"=632.0, "To (nm)"=1000.0, "Integration Time (s)"=3.0, "Number of Accumulations"=3, "AutoScanning"=FALSE, "Spike Removal"=FALSE} ("Acquisition Settings 2"), Variant=w255) -> (data=w249:T50, error out=w253:errorcluster)
        n125 = Bundle By Name(cluster=T43 {"Laser Settings"={"Laser Wavelength"=enum."633 nm", "Neutral Density Filter"=enum."1%"}, "Spectrometer Settings"={"Confocal Hole Size (µm)"=150.0, "Grating"=1, "Detector"=enum."InGaAs Array"}, "Acquisition Settings"={"Acquisition Mode"=enum."Single Window", "Spectal Position (nm)"=480.0, "From (nm)"=632.0, "To (nm)"=1000.0, "Integration Time (s)"=3.0, "Number of Accumulations"=3, "AutoScanning"=FALSE, "Spike Removal"=FALSE}, "Path"=path ""} ("LabramHR"), "Acquisition Settings"=w249) -> (w248:T43)
        n126 = Unbundle By Name(w250) -> ("Optical Spectrometer"=w251:refnum<queue>)
        n127 = call "Enqueue Message (Single).vi"("error in (no error)"=w253, "Message Data"=w248, "Message"="Set Acquisition Settings", "Message Queue"=w251) -> ("error out"=w254:errorcluster)  [unwired: 7 out]
      }
      frame "LabramHR - Acquire Spectrum" {
        n128 = Unbundle By Name(w258) -> ("Optical Spectrometer"=w259:refnum<queue>)
        n129 = call "Enqueue Message (Single).vi"("error in (no error)"=w260, "Message"="Acquire Spectrum", "Message Queue"=w259) -> ("error out"=w257:errorcluster)  [unwired: 1 in, 7 out]
      }
      frame "LabramHR - Save Spectrum" {
        n130 = Unbundle By Name(w263) -> ("Optical Spectrometer"=w264:refnum<queue>)
        n131 = call "Enqueue Message (Single).vi"("error in (no error)"=w265, "Message"="Save Optical Spectrum", "Message Queue"=w264) -> ("error out"=w262:errorcluster)  [unwired: 1 in, 7 out]
      }
      frame "----- Switches & Mirrors Events -----" {
        # "Switches & Mirrors EVENTS"
      }
      frame "Switches & Mirrors - Update Visa Session" {
        n132 = Variant To Data(error in=w275, type=refnum<visa-resource-name> "COM1" ("Laser Video VISA Session 2"), Variant=w271) -> (data=w270:refnum<visa-resource-name>, error out=w273:errorcluster)
        n133 = Bundle By Name(cluster=T51 {"Relay VISA Session"="COM1", "Switches"={"Laser"=FALSE, "Video"=FALSE}, "Delays (ms)"={"Laser"=500, "Video"=1500}} ("Laser-Video Config"), "Relay VISA Session"=w270) -> (w269:T51)
        n134 = Unbundle By Name(w276) -> ("Switches & Mirrors"=w277:refnum<queue>)
        n135 = call "Enqueue Message (Single).vi"("error in (no error)"=w273, "Message Data"=w269, "Message"="Update VISA Session", "Message Queue"=w277) -> ("error out"=w278:errorcluster)  [unwired: 7 out]
      }
      frame "Switches & Mirrors - Update Laser" {
        n136 = Variant To Data(error in=w288, type=FALSE ("Laser"), Variant=w289) -> (data=w279:bool, error out=w286:errorcluster)
        n137 = Bundle By Name(cluster=T51 {"Relay VISA Session"="COM1", "Switches"={"Laser"=FALSE, "Video"=FALSE}, "Delays (ms)"={"Laser"=500, "Video"=1500}} ("Laser-Video Config"), "Switches.Laser"=w279) -> (w282:T51)
        n138 = Unbundle By Name(w284) -> ("Switches & Mirrors"=w285:refnum<queue>)
        n139 = call "Enqueue Message (Single).vi"("error in (no error)"=w286, "Message Data"=w282, "Message"="Update Laser", "Message Queue"=w285) -> ("error out"=w287:errorcluster)  [unwired: 7 out]
      }
      frame "Switches & Mirrors - Update Video" {
        n140 = Variant To Data(error in=w299, type=FALSE ("Laser"), Variant=w300) -> (data=w290:bool, error out=w297:errorcluster)
        n141 = Bundle By Name(cluster=T51 {"Relay VISA Session"="COM1", "Switches"={"Laser"=FALSE, "Video"=FALSE}, "Delays (ms)"={"Laser"=500, "Video"=1500}} ("Laser-Video Config"), "Switches.Video"=w290) -> (w293:T51)
        n142 = Unbundle By Name(w295) -> ("Switches & Mirrors"=w296:refnum<queue>)
        n143 = call "Enqueue Message (Single).vi"("error in (no error)"=w297, "Message Data"=w293, "Message"="Update Video", "Message Queue"=w296) -> ("error out"=w298:errorcluster)  [unwired: 7 out]
      }
      frame "----- Camera Events -----" {
        # "uEye Camera EVENTS"
      }
      frame "Camera - Update Settings" {
        w304 = T53 {"Settings"={"Pixel clock"=20, "Frame rate"=30.0, "Exposure time"=33.21525, "Master Gain"=0, "Red Gain"=0, "Green Gain"=0, "Blue Gain"=0, "Auto Gain"=FALSE, "White-balance"=FALSE, "Color Correction"=FALSE}} ("Camera Configuration")
        n144 = Unbundle By Name(w304) -> ("Settings"=w305:T54)
        n145 = Variant To Data(error in=w311, type=w305, Variant=w312) -> (data=w302:T54, error out=w306:errorcluster)
        n146 = Bundle By Name(cluster=w304, "Settings"=w302) -> (w303:T53)
        n147 = Unbundle By Name(w308) -> ("Camera"=w309:refnum<queue>)
        n148 = call "Enqueue Message (Single).vi"("error in (no error)"=w306, "Message Data"=w303, "Message"="Update Settings", "Message Queue"=w309) -> ("error out"=w310:errorcluster)  [unwired: 7 out]
      }
      frame "Camera - Popup" {
        n149 = Unbundle By Name(w315) -> ("Camera"=w316:refnum<queue>)
        n150 = call "Enqueue Message (Single).vi"("error in (no error)"=w313, "Message"="Popup", "Message Queue"=w316) -> ("error out"=w317:errorcluster)  [unwired: 1 in, 7 out]
      }
      frame "Camera - Start Live" {
        n151 = Unbundle By Name(w320) -> ("Camera"=w321:refnum<queue>)
        n152 = call "Enqueue Message (Single).vi"("error in (no error)"=w318, "Message"="Start Live", "Message Queue"=w321) -> ("error out"=w322:errorcluster)  [unwired: 1 in, 7 out]
      }
      frame "Camera - Stop Live" {
        n153 = Unbundle By Name(w325) -> ("Camera"=w326:refnum<queue>)
        n154 = call "Enqueue Message (Single).vi"("error in (no error)"=w323, "Message"="Stop Live", "Message Queue"=w326) -> ("error out"=w327:errorcluster)  [unwired: 1 in, 7 out]
      }
      frame "----- Stress Control Events -----" {
        # "Stress Control Events"
      }
      frame "Stress Control - Set UI" {
        n155 = Variant To Data(error in=w334, type=T42 {"Stress Control VISA Session"="", "Axis"=1, "Motion"=0, "Destination (°)"=0.0, "Speed (°/s)"=4.0, "Position (°)"=0.0} ("Stress Control Configuration"), Variant=w332) -> (data=w331:T42, error out=w333:errorcluster)
        n156 = Unbundle By Name(w331) -> ("Stress Control VISA Session"=w338:refnum<visa-resource-name>, "Motion"=w337:u16, "Destination (°)"=w336:dbl, "Speed (°/s)"=w335:dbl, "Position (°)"=→"Position (°)":dbl)
        n157 = property on="Stress Controller VISA Session" class="VISAName"("Value"=w338) -> ()  [unwired: 2 in, 2 out]
        n158 = property on="Mechanism Motion" class="Ring (strict)"("Value"=w337) -> ()  [unwired: 2 in, 2 out]
        n159 = property on="Destination (°)" class="DigNum (strict)"("Value"=w336) -> ()  [unwired: 2 in, 2 out]
        n160 = property on="Speed (°/s)" class="DigNum (strict)"("Value"=w335) -> ()  [unwired: 2 in, 2 out]
      }
      frame "Stress Control - Update Refnums" {
        n161 = control-ref of="Stress Control"() -> (w340:refnum<vi>)
        n162 = control-ref of="Position (°)"() -> (w350:refnum<vi>)
        n163 = control-ref of="Mechanism Motion"() -> (w349:refnum<vi>)
        n164 = control-ref of="Destination (°)"() -> (w348:refnum<vi>)
        n165 = control-ref of="Stop"() -> (w342:refnum<vi>)
        n166 = Bundle By Name(cluster=T74 {"Instrument Status"=refnum, "Position"=refnum, "Mecahnism Motion"=refnum, "Destination"=refnum, "Apply Stress"=refnum, "Stop"=refnum, "Stress Control VISA"=refnum} ("Stress Control Refnums"), "Instrument Status"=w340, "Position"=w350, "Mecahnism Motion"=w349, "Destination"=w348, "Stop"=w342) -> (w341:T74)
        n167 = Unbundle By Name(w343) -> ("Stress Control"=w344:refnum<queue>)
        n168 = call "Enqueue Message (Single).vi"("error in (no error)"=w347, "Message Data"=w341, "Message"="Update Refnums", "Message Queue"=w344) -> ("error out"=w346:errorcluster)  [unwired: 7 out]
      }
      frame "Stress Control - Update VISA Session" {
        n169 = Variant To Data(error in=w361, type=refnum<visa-resource-name> "StrainMotor" ("Stress Controller VISA Session 2"), Variant=w354) -> (data=w353:refnum<visa-resource-name>, error out=w356:errorcluster)
        n170 = Bundle By Name(cluster=T42 {"Stress Control VISA Session"="", "Axis"=1, "Motion"=0, "Destination (°)"=0.0, "Speed (°/s)"=4.0, "Position (°)"=0.0} ("Stress Control Configuration"), "Stress Control VISA Session"=w353) -> (w352:T42)
        n171 = Unbundle By Name(w357) -> ("Stress Control"=w358:refnum<queue>)
        n172 = call "Enqueue Message (Single).vi"("error in (no error)"=w356, "Message Data"=w352, "Message"="Update Visa Session", "Message Queue"=w358) -> ("error out"=w360:errorcluster)  [unwired: 7 out]
      }
      frame "Stress Control - Update Configuration" {
        n173 = Variant To Data(error in=w372, type=4.0 ("Speed (°/s) 2"), Variant=w366) -> (data=w364:dbl, error out=w367:errorcluster)
        n174 = Bundle By Name(cluster=T42 {"Stress Control VISA Session"="", "Axis"=1, "Motion"=0, "Destination (°)"=0.0, "Speed (°/s)"=4.0, "Position (°)"=0.0} ("Stress Control Configuration"), "Speed (°/s)"=w364) -> (w363:T42)
        n175 = Unbundle By Name(w368) -> ("Stress Control"=w369:refnum<queue>)
        n176 = call "Enqueue Message (Single).vi"("error in (no error)"=w367, "Message Data"=w363, "Message"="Update Configuration", "Message Queue"=w369) -> ("error out"=w371:errorcluster)  [unwired: 7 out]
      }
      frame "Stress Control - Update Motion Mode" {
        w376 = u16 0 items=["Absolute", "Relative"] ("Motion 2")
        n177 = Variant To Data(error in=w383, type=w376, Variant=w377) -> (data=w375:u16, error out=w378:errorcluster)
        n178 = Bundle By Name(cluster=T42 {"Stress Control VISA Session"="", "Axis"=1, "Motion"=0, "Destination (°)"=0.0, "Speed (°/s)"=4.0, "Position (°)"=0.0} ("Stress Control Configuration"), "Motion"=w375) -> (w374:T42)
        n179 = Unbundle By Name(w379) -> ("Stress Control"=w380:refnum<queue>)
        n180 = call "Enqueue Message (Single).vi"("error in (no error)"=w378, "Message Data"=w374, "Message"="Update Motion Mode", "Message Queue"=w380) -> ("error out"=w382:errorcluster)  [unwired: 7 out]
      }
      frame "Stress Control - Update Destination" {
        n181 = Variant To Data(error in=w394, type=0.0 ("Destination (°) 2"), Variant=w388) -> (data=w387:dbl, error out=w389:errorcluster)
        n182 = Bundle By Name(cluster=T42 {"Stress Control VISA Session"="", "Axis"=1, "Motion"=0, "Destination (°)"=0.0, "Speed (°/s)"=4.0, "Position (°)"=0.0} ("Stress Control Configuration"), "Destination (°)"=w387) -> (w385:T42)
        n183 = Unbundle By Name(w390) -> ("Stress Control"=w391:refnum<queue>)
        n184 = call "Enqueue Message (Single).vi"("error in (no error)"=w389, "Message Data"=w385, "Message"="Update Destination", "Message Queue"=w391) -> ("error out"=w393:errorcluster)  [unwired: 7 out]
      }
      frame "Stress Control - Change Stress" {
        n185 = Unbundle By Name(w397) -> ("Stress Control"=w398:refnum<queue>)
        n186 = call "Enqueue Message (Single).vi"("error in (no error)"=w395, "Message"="Change Stress", "Message Queue"=w398) -> ("error out"=w399:errorcluster)  [unwired: 1 in, 7 out]
      }
      frame "----- Parameter Analyzer Events -----" {
        # "Parameter Analyzer Events"
      }
      frame "Parameter Analyzer - Set UI" {
        n187 = Variant To Data(error in=w421, type=T33 {"Parameter Analyzer VISA Session"="COM1", "Sweeping Time Parameters"={"Integration Time"=0, "Short Integration Time (s)"=0.0, "Long Integration Time (s)"=0.0, "Wait Time Parameter"=1.0}, "Acquisition Mode"=enum."Sweeping Mode", "Status Polling Time (ms)"=1000, "Comment"="Test VI", "SMU 1 - Sweeping"={"Start / Offset"=0.0, "Stop / Ratio"=1.0, "Step \n(linear only)"=0.01, "Compliance"=0.1, "Power \nCompliance"=0.0, "Mode"=0, "Function"=0, "Sweep Mode"=FALSE}, "SMU 2 - Sweeping"={"Start / Offset"=0.0, "Stop / Ratio"=1.0, "Step \n(linear only)"=0.01, "Compliance"=0.1, "Power \nCompliance"=0.0, "Mode"=0, "Function"=0, "Sweep Mode"=FALSE}, "SMU 3 - Sweeping"={"Start / Offset"=0.0, "Stop / Ratio"=1.0, "Step \n(linear only)"=0.01, "Compliance"=0.1, "Power \nCompliance"=0.0, "Mode"=0, "Function"=0, "Sweep Mode"=FALSE}, "SMU 4 - Sweeping"={"Start / Offset"=0.0, "Stop / Ratio"=1.0, "Step \n(linear only)"=0.01, "Compliance"=0.1, "Power \nCompliance"=0.0, "Mode"=1, "Function"=0, "Sweep Mode"=FALSE}, "Sweep Spacing"=0, "Range"=0, "SMU1 - Sampling"={"Source"=10.0, "Compliance"=1e-05, "Mode"=0, "Function"=FALSE}, "SMU2 - Sampling"={"Source"=10.0, "Compliance"=1e-05, "Mode"=0, "Function"=FALSE}, "SMU3 - Sampling"={"Source"=10.0, "Compliance"=1e-05, "Mode"=0, "Function"=FALSE}, "SMU4 - Sampling"={"Source"=10.0, "Compliance"=1e-05, "Mode"=0, "Function"=FALSE}, "Sampling Time Parameters"={"Initial Interval (s)"=0.1, "Number of Samples"=60, "Total Sampling Time (s)"=10.0, "Hold Time (s)"=0.0, "Sampling Mode"=0, "Sampling Time"=0}, "Stop Condition"={"Enable Delay (s)"=0.0, "Name"="", "Threshold"=0.0, "num. of events"=1, "Event"=0, "Stop Condition Enable"=FALSE}} ("HP4155C Configuration"), Variant=w417) -> (data=w402:T33, error out=w418:errorcluster)
        n188 = Unbundle By Name(w402) -> ("Parameter Analyzer VISA Session"=w404:refnum<visa-resource-name>, "Status Polling Time (ms)"=w403:u32)
        n189 = Unbundle By Name(w402) -> ("Sweeping Time Parameters"=w416:T34, "Acquisition Mode"=w420:enum32{"Sweeping Mode", "Sampling Mode"}, "SMU 1 - Sweeping"=w415:T35, "SMU 2 - Sweeping"=w414:T35, "SMU 3 - Sweeping"=w413:T35, "SMU 4 - Sweeping"=w412:T35, "Sweep Spacing"=w419:T36, "Range"=w411:T37, "SMU1 - Sampling"=w410:T38, "SMU2 - Sampling"=w409:T38, "SMU3 - Sampling"=w408:T38, "SMU4 - Sampling"=w407:T38, "Sampling Time Parameters"=w406:T39, "Stop Condition"=w405:T40)
        n190 = property on="User Integration Time" class="Clust (strict)"("Value"=w416) -> ()  [unwired: 2 in, 2 out]
        n191 = property on="Acquisition Mode" class="TabCtl (strict)"("Value"=w420) -> ()  [unwired: 2 in, 2 out]
        n192 = property on="SMU 1 - Sweeping" class="Clust (strict)"("Value"=w415) -> ()  [unwired: 2 in, 2 out]
        n193 = property on="SMU 2 - Sweeping" class="Clust (strict)"("Value"=w414) -> ()  [unwired: 2 in, 2 out]
        n194 = property on="SMU 3 - Sweeping" class="Clust (strict)"("Value"=w413) -> ()  [unwired: 2 in, 2 out]
        n195 = property on="SMU 4 - Sweeping" class="Clust (strict)"("Value"=w412) -> ()  [unwired: 2 in, 2 out]
        n196 = property on="Sweep Spacing" class="Ring (strict)"("Value"=w419) -> ()  [unwired: 2 in, 2 out]
        n197 = property on="Range" class="Ring (strict)"("Value"=w411) -> ()  [unwired: 2 in, 2 out]
        n198 = property on="Pameter Analyzer VISA Session" class="VISAName"("Value"=w404) -> ()  [unwired: 2 in, 2 out]
        n199 = property on="Status Polling Time (ms)" class="DigNum (strict)"("Value"=w403) -> ()  [unwired: 2 in, 2 out]
        n200 = property on="SMU1 - Sampling" class="Clust (strict)"("Value"=w410) -> ()  [unwired: 2 in, 2 out]
        n201 = property on="SMU2 - Sampling" class="Clust (strict)"("Value"=w409) -> ()  [unwired: 2 in, 2 out]
        n202 = property on="SMU3 - Sampling" class="Clust (strict)"("Value"=w408) -> ()  [unwired: 2 in, 2 out]
        n203 = property on="SMU4 - Sampling" class="Clust (strict)"("Value"=w407) -> ()  [unwired: 2 in, 2 out]
        n204 = property on="Sampling Parameters" class="Clust (strict)"("Value"=w406) -> ()  [unwired: 2 in, 2 out]
        n205 = property on="Stop Condition" class="Clust (strict)"("Value"=w405) -> ()  [unwired: 2 in, 2 out]
      }
      frame "Parameter Analyzer - Set Settings" {
        n206 = Variant To Data(error in=w425, type=T33 {"Parameter Analyzer VISA Session"="COM1", "Sweeping Time Parameters"={"Integration Time"=0, "Short Integration Time (s)"=0.0, "Long Integration Time (s)"=0.0, "Wait Time Parameter"=1.0}, "Acquisition Mode"=enum."Sweeping Mode", "Status Polling Time (ms)"=1000, "Comment"="Test VI", "SMU 1 - Sweeping"={"Start / Offset"=0.0, "Stop / Ratio"=1.0, "Step \n(linear only)"=0.01, "Compliance"=0.1, "Power \nCompliance"=0.0, "Mode"=0, "Function"=0, "Sweep Mode"=FALSE}, "SMU 2 - Sweeping"={"Start / Offset"=0.0, "Stop / Ratio"=1.0, "Step \n(linear only)"=0.01, "Compliance"=0.1, "Power \nCompliance"=0.0, "Mode"=0, "Function"=0, "Sweep Mode"=FALSE}, "SMU 3 - Sweeping"={"Start / Offset"=0.0, "Stop / Ratio"=1.0, "Step \n(linear only)"=0.01, "Compliance"=0.1, "Power \nCompliance"=0.0, "Mode"=0, "Function"=0, "Sweep Mode"=FALSE}, "SMU 4 - Sweeping"={"Start / Offset"=0.0, "Stop / Ratio"=1.0, "Step \n(linear only)"=0.01, "Compliance"=0.1, "Power \nCompliance"=0.0, "Mode"=1, "Function"=0, "Sweep Mode"=FALSE}, "Sweep Spacing"=0, "Range"=0, "SMU1 - Sampling"={"Source"=10.0, "Compliance"=1e-05, "Mode"=0, "Function"=FALSE}, "SMU2 - Sampling"={"Source"=10.0, "Compliance"=1e-05, "Mode"=0, "Function"=FALSE}, "SMU3 - Sampling"={"Source"=10.0, "Compliance"=1e-05, "Mode"=0, "Function"=FALSE}, "SMU4 - Sampling"={"Source"=10.0, "Compliance"=1e-05, "Mode"=0, "Function"=FALSE}, "Sampling Time Parameters"={"Initial Interval (s)"=0.1, "Number of Samples"=60, "Total Sampling Time (s)"=10.0, "Hold Time (s)"=0.0, "Sampling Mode"=0, "Sampling Time"=0}, "Stop Condition"={"Enable Delay (s)"=0.0, "Name"="", "Threshold"=0.0, "num. of events"=1, "Event"=0, "Stop Condition Enable"=FALSE}} ("HP4155C Configuration"), Variant=w423) -> (error out=w424:errorcluster)  [unwired: 1 out]
      }
      frame "Parameter Analyzer - Update Visa Session" {
        w427 = T33 {"Parameter Analyzer VISA Session"="COM1", "Sweeping Time Parameters"={"Integration Time"=0, "Short Integration Time (s)"=0.0, "Long Integration Time (s)"=0.0, "Wait Time Parameter"=1.0}, "Acquisition Mode"=enum."Sweeping Mode", "Status Polling Time (ms)"=1000, "Comment"="Test VI", "SMU 1 - Sweeping"={"Start / Offset"=0.0, "Stop / Ratio"=1.0, "Step \n(linear only)"=0.01, "Compliance"=0.1, "Power \nCompliance"=0.0, "Mode"=0, "Function"=0, "Sweep Mode"=FALSE}, "SMU 2 - Sweeping"={"Start / Offset"=0.0, "Stop / Ratio"=1.0, "Step \n(linear only)"=0.01, "Compliance"=0.1, "Power \nCompliance"=0.0, "Mode"=0, "Function"=0, "Sweep Mode"=FALSE}, "SMU 3 - Sweeping"={"Start / Offset"=0.0, "Stop / Ratio"=1.0, "Step \n(linear only)"=0.01, "Compliance"=0.1, "Power \nCompliance"=0.0, "Mode"=0, "Function"=0, "Sweep Mode"=FALSE}, "SMU 4 - Sweeping"={"Start / Offset"=0.0, "Stop / Ratio"=1.0, "Step \n(linear only)"=0.01, "Compliance"=0.1, "Power \nCompliance"=0.0, "Mode"=1, "Function"=0, "Sweep Mode"=FALSE}, "Sweep Spacing"=0, "Range"=0, "SMU1 - Sampling"={"Source"=10.0, "Compliance"=1e-05, "Mode"=0, "Function"=FALSE}, "SMU2 - Sampling"={"Source"=10.0, "Compliance"=1e-05, "Mode"=0, "Function"=FALSE}, "SMU3 - Sampling"={"Source"=10.0, "Compliance"=1e-05, "Mode"=0, "Function"=FALSE}, "SMU4 - Sampling"={"Source"=10.0, "Compliance"=1e-05, "Mode"=0, "Function"=FALSE}, "Sampling Time Parameters"={"Initial Interval (s)"=0.1, "Number of Samples"=60, "Total Sampling Time (s)"=10.0, "Hold Time (s)"=0.0, "Sampling Mode"=0, "Sampling Time"=0}, "Stop Condition"={"Enable Delay (s)"=0.0, "Name"="", "Threshold"=0.0, "num. of events"=1, "Event"=0, "Stop Condition Enable"=FALSE}} ("HP4155C Configuration")
        n207 = Unbundle By Name(w427) -> ("Parameter Analyzer VISA Session"=w428:refnum<visa-resource-name>)
        n208 = Variant To Data(error in=w436, type=w428, Variant=w435) -> (data=w426:refnum<visa-resource-name>, error out=w431:errorcluster)
        n209 = Bundle By Name(cluster=w427, "Parameter Analyzer VISA Session"=w426) -> (w429:T33)
        n210 = Unbundle By Name(w432) -> ("Parameter Analyzer"=w433:refnum<queue>)
        n211 = call "Enqueue Message (Single).vi"("error in (no error)"=w431, "Message Data"=w429, "Message"="Update Visa Session", "Message Queue"=w433) -> ("error out"=w430:errorcluster)  [unwired: 7 out]
      }
      frame "Parameter Analyzer - Update Refnums" {
        n212 = control-ref of="Plot List"() -> (w442:refnum<vi>)
        n213 = control-ref of="Voltage Plot"() -> (w441:refnum<vi>)
        n214 = control-ref of="Current Plot"() -> (w440:refnum<vi>)
        n215 = control-ref of="Current Voltage Characteristic"() -> (w438:refnum<vi>)
        n216 = control-ref of="Differential Resistance"() -> (w439:refnum<vi>)
        n217 = control-ref of="Parameter Analyzer"() -> (w443:refnum<vi>)
        n218 = Bundle By Name(cluster=T75 {"Status"=refnum, "Electrical Measurement"=refnum, "Plots"={"Plot List"=refnum, "Voltage Plot"=refnum, "Current Plot"=refnum, "IV Characteristic"=refnum, "dI/dV-V Characteristic"=refnum}, "HP Integration Time"=refnum, "VISA"=refnum, "Sweeping Time Parameters"=refnum, "Acquisition Mode"=refnum, "SMU 1 - Sweeping"=refnum, "SMU 2 - Sweeping"=refnum, "SMU 3 - Sweeping"=refnum, "SMU 4 - Sweeping"=refnum, "Sweep Spacing"=refnum, "Range"=refnum, "SMU1 - Sampling"=refnum, "SMU2 - Sampling"=refnum, "SMU3 - Sampling"=refnum, "SMU4 - Sampling"=refnum, "Sampling Time Parameters"=refnum, "Stop Condition"=refnum, "Instrument Status"=refnum} ("HP4155C Refnums"), "Plots.Plot List"=w442, "Plots.Voltage Plot"=w441, "Plots.Current Plot"=w440, "Plots.IV Characteristic"=w438, "Plots.dI/dV-V Characteristic"=w439, "Instrument Status"=w443) -> (w444:T75)
        n219 = Unbundle By Name(w447) -> ("Parameter Analyzer"=w448:refnum<queue>)
        n220 = call "Enqueue Message (Single).vi"("error in (no error)"=w446, "Message Data"=w444, "Message"="Update Refnums", "Message Queue"=w448) -> ("error out"=w445:errorcluster)  [unwired: 7 out]
      }
      frame "Parameter Analyzer - Update Acquisition Mode" {
        n221 = Variant To Data(error in=w472, type=enum32{"Sweeping Mode", "Sampling Mode"}."Sweeping Mode" ("Acquisition Mode 2"), Variant=w471) -> (data=w467:enum32{"Sweeping Mode", "Sampling Mode"}, error out=w468:errorcluster)
        n222 = property on="Sampling Parameters" class="Clust (strict)"() -> ("Value"=w452:T14)  [unwired: 2 in, 2 out]
        n223 = property on="Stop Condition" class="Clust (strict)"() -> ("Value"=w451:T13)  [unwired: 2 in, 2 out]
        n224 = property on="SMU3 - Sampling" class="Clust (strict)"() -> ("Value"=w457:T12)  [unwired: 2 in, 2 out]
        n225 = property on="SMU1 - Sampling" class="Clust (strict)"() -> ("Value"=w458:T12)  [unwired: 2 in, 2 out]
        n226 = property on="SMU2 - Sampling" class="Clust (strict)"() -> ("Value"=w459:T12)  [unwired: 2 in, 2 out]
        n227 = property on="SMU4 - Sampling" class="Clust (strict)"() -> ("Value"=w460:T12)  [unwired: 2 in, 2 out]
        n228 = case shown="\"Sweeping Mode\", Default" w467 {
          tunnel: ["Configure Sweeping" ("Message") "Configure Sampling" ("Message")] -> w466
          frame "Sweeping Mode", Default {
          }
          frame "Sampling Mode" {
          }
        }
        n229 = property on="SMU 1 - Sweeping" class="Clust (strict)"() -> ("Value"=w453:T11)  [unwired: 2 in, 2 out]
        n230 = property on="SMU 2 - Sweeping" class="Clust (strict)"() -> ("Value"=w454:T11)  [unwired: 2 in, 2 out]
        n231 = property on="SMU 3 - Sweeping" class="Clust (strict)"() -> ("Value"=w455:T11)  [unwired: 2 in, 2 out]
        n232 = property on="SMU 4 - Sweeping" class="Clust (strict)"() -> ("Value"=w456:T11)  [unwired: 2 in, 2 out]
        n233 = property on="Sweep Spacing" class="Ring (strict)"() -> ("Value"=w462:u16)  [unwired: 2 in, 2 out]
        n234 = property on="Range" class="Ring (strict)"() -> ("Value"=w463:u16)  [unwired: 2 in, 2 out]
        n235 = Bundle By Name(cluster=T33 {"Parameter Analyzer VISA Session"="COM1", "Sweeping Time Parameters"={"Integration Time"=0, "Short Integration Time (s)"=0.0, "Long Integration Time (s)"=0.0, "Wait Time Parameter"=1.0}, "Acquisition Mode"=enum."Sweeping Mode", "Status Polling Time (ms)"=1000, "Comment"="Test VI", "SMU 1 - Sweeping"={"Start / Offset"=0.0, "Stop / Ratio"=1.0, "Step \n(linear only)"=0.01, "Compliance"=0.1, "Power \nCompliance"=0.0, "Mode"=0, "Function"=0, "Sweep Mode"=FALSE}, "SMU 2 - Sweeping"={"Start / Offset"=0.0, "Stop / Ratio"=1.0, "Step \n(linear only)"=0.01, "Compliance"=0.1, "Power \nCompliance"=0.0, "Mode"=0, "Function"=0, "Sweep Mode"=FALSE}, "SMU 3 - Sweeping"={"Start / Offset"=0.0, "Stop / Ratio"=1.0, "Step \n(linear only)"=0.01, "Compliance"=0.1, "Power \nCompliance"=0.0, "Mode"=0, "Function"=0, "Sweep Mode"=FALSE}, "SMU 4 - Sweeping"={"Start / Offset"=0.0, "Stop / Ratio"=1.0, "Step \n(linear only)"=0.01, "Compliance"=0.1, "Power \nCompliance"=0.0, "Mode"=1, "Function"=0, "Sweep Mode"=FALSE}, "Sweep Spacing"=0, "Range"=0, "SMU1 - Sampling"={"Source"=10.0, "Compliance"=1e-05, "Mode"=0, "Function"=FALSE}, "SMU2 - Sampling"={"Source"=10.0, "Compliance"=1e-05, "Mode"=0, "Function"=FALSE}, "SMU3 - Sampling"={"Source"=10.0, "Compliance"=1e-05, "Mode"=0, "Function"=FALSE}, "SMU4 - Sampling"={"Source"=10.0, "Compliance"=1e-05, "Mode"=0, "Function"=FALSE}, "Sampling Time Parameters"={"Initial Interval (s)"=0.1, "Number of Samples"=60, "Total Sampling Time (s)"=10.0, "Hold Time (s)"=0.0, "Sampling Mode"=0, "Sampling Time"=0}, "Stop Condition"={"Enable Delay (s)"=0.0, "Name"="", "Threshold"=0.0, "num. of events"=1, "Event"=0, "Stop Condition Enable"=FALSE}} ("HP4155C Configuration"), "SMU 1 - Sweeping"=w453, "SMU 2 - Sweeping"=w454, "SMU 3 - Sweeping"=w455, "SMU 4 - Sweeping"=w456, "Sweep Spacing"=w462, "Range"=w463, "SMU1 - Sampling"=w457, "SMU2 - Sampling"=w458, "SMU3 - Sampling"=w459, "SMU4 - Sampling"=w460, "Sampling Time Parameters"=w452, "Stop Condition"=w451) -> (w461:T33)
        n236 = Unbundle By Name(w465) -> ("Parameter Analyzer"=w464:refnum<queue>)
        n237 = call "Enqueue Message (Single).vi"("error in (no error)"=w468, "Message Data"=w461, "Message"=w466, "Message Queue"=w464) -> ("error out"=w469:errorcluster)  [unwired: 7 out]
      }
      frame "Parameter Analyzer - Configure Integration time" {
        w475 = T33 {"Parameter Analyzer VISA Session"="COM1", "Sweeping Time Parameters"={"Integration Time"=0, "Short Integration Time (s)"=0.0, "Long Integration Time (s)"=0.0, "Wait Time Parameter"=1.0}, "Acquisition Mode"=enum."Sweeping Mode", "Status Polling Time (ms)"=1000, "Comment"="Test VI", "SMU 1 - Sweeping"={"Start / Offset"=0.0, "Stop / Ratio"=1.0, "Step \n(linear only)"=0.01, "Compliance"=0.1, "Power \nCompliance"=0.0, "Mode"=0, "Function"=0, "Sweep Mode"=FALSE}, "SMU 2 - Sweeping"={"Start / Offset"=0.0, "Stop / Ratio"=1.0, "Step \n(linear only)"=0.01, "Compliance"=0.1, "Power \nCompliance"=0.0, "Mode"=0, "Function"=0, "Sweep Mode"=FALSE}, "SMU 3 - Sweeping"={"Start / Offset"=0.0, "Stop / Ratio"=1.0, "Step \n(linear only)"=0.01, "Compliance"=0.1, "Power \nCompliance"=0.0, "Mode"=0, "Function"=0, "Sweep Mode"=FALSE}, "SMU 4 - Sweeping"={"Start / Offset"=0.0, "Stop / Ratio"=1.0, "Step \n(linear only)"=0.01, "Compliance"=0.1, "Power \nCompliance"=0.0, "Mode"=1, "Function"=0, "Sweep Mode"=FALSE}, "Sweep Spacing"=0, "Range"=0, "SMU1 - Sampling"={"Source"=10.0, "Compliance"=1e-05, "Mode"=0, "Function"=FALSE}, "SMU2 - Sampling"={"Source"=10.0, "Compliance"=1e-05, "Mode"=0, "Function"=FALSE}, "SMU3 - Sampling"={"Source"=10.0, "Compliance"=1e-05, "Mode"=0, "Function"=FALSE}, "SMU4 - Sampling"={"Source"=10.0, "Compliance"=1e-05, "Mode"=0, "Function"=FALSE}, "Sampling Time Parameters"={"Initial Interval (s)"=0.1, "Number of Samples"=60, "Total Sampling Time (s)"=10.0, "Hold Time (s)"=0.0, "Sampling Mode"=0, "Sampling Time"=0}, "Stop Condition"={"Enable Delay (s)"=0.0, "Name"="", "Threshold"=0.0, "num. of events"=1, "Event"=0, "Stop Condition Enable"=FALSE}} ("HP4155C Configuration")
        n238 = Unbundle By Name(w475) -> ("Sweeping Time Parameters"=w476:T34)
        n239 = Variant To Data(error in=w485, type=w476, Variant=w484) -> (data=w477:T34, error out=w481:errorcluster)
        n240 = Bundle By Name(cluster=w475, "Sweeping Time Parameters"=w477) -> (w478:T33)
        n241 = Unbundle By Name(w479) -> ("Parameter Analyzer"=w482:refnum<queue>)
        n242 = call "Enqueue Message (Single).vi"("error in (no error)"=w481, "Message Data"=w478, "Message"="Configure Integration Time", "Message Queue"=w482) -> ("error out"=w480:errorcluster)  [unwired: 7 out]
      }
      frame "Parameter Analyzer - Configure Sweeping" {
        n243 = Variant To Data(error in=w502, type=T77 {"SMU 1 - Sweeping"={"Start / Offset"=0.0, "Stop / Ratio"=0.0, "Step (linear only)"=0.0, "Compliance"=0.0, "Power Compliance"=0.0, "Mode"=0, "Function"=0, "Sweep Mode"=FALSE}, "SMU 2 - Sweeping"={"Start / Offset"=0.0, "Stop / Ratio"=0.0, "Step (linear only)"=0.0, "Compliance"=0.0, "Power Compliance"=0.0, "Mode"=0, "Function"=0, "Sweep Mode"=FALSE}, "SMU 3 - Sweeping"={"Start / Offset"=0.0, "Stop / Ratio"=0.0, "Step (linear only)"=0.0, "Compliance"=0.0, "Power Compliance"=0.0, "Mode"=0, "Function"=0, "Sweep Mode"=FALSE}, "SMU 4 - Sweeping"={"Start / Offset"=0.0, "Stop / Ratio"=0.0, "Step (linear only)"=0.0, "Compliance"=0.0, "Power Compliance"=0.0, "Mode"=0, "Function"=0, "Sweep Mode"=FALSE}, "Sweep Spacing"=0, "Range"=0} ("output cluster"), Variant=w501) -> (data=w500:T77, error out=w492:errorcluster)
        n244 = Unbundle By Name(w500) -> ("SMU 1 - Sweeping"=w495:T84, "SMU 2 - Sweeping"=w496:T84, "SMU 3 - Sweeping"=w497:T84, "SMU 4 - Sweeping"=w498:T84, "Sweep Spacing"=w499:u16, "Range"=w489:u16)
        n245 = Bundle By Name(cluster=T33 {"Parameter Analyzer VISA Session"="COM1", "Sweeping Time Parameters"={"Integration Time"=0, "Short Integration Time (s)"=0.0, "Long Integration Time (s)"=0.0, "Wait Time Parameter"=1.0}, "Acquisition Mode"=enum."Sweeping Mode", "Status Polling Time (ms)"=1000, "Comment"="Test VI", "SMU 1 - Sweeping"={"Start / Offset"=0.0, "Stop / Ratio"=1.0, "Step \n(linear only)"=0.01, "Compliance"=0.1, "Power \nCompliance"=0.0, "Mode"=0, "Function"=0, "Sweep Mode"=FALSE}, "SMU 2 - Sweeping"={"Start / Offset"=0.0, "Stop / Ratio"=1.0, "Step \n(linear only)"=0.01, "Compliance"=0.1, "Power \nCompliance"=0.0, "Mode"=0, "Function"=0, "Sweep Mode"=FALSE}, "SMU 3 - Sweeping"={"Start / Offset"=0.0, "Stop / Ratio"=1.0, "Step \n(linear only)"=0.01, "Compliance"=0.1, "Power \nCompliance"=0.0, "Mode"=0, "Function"=0, "Sweep Mode"=FALSE}, "SMU 4 - Sweeping"={"Start / Offset"=0.0, "Stop / Ratio"=1.0, "Step \n(linear only)"=0.01, "Compliance"=0.1, "Power \nCompliance"=0.0, "Mode"=1, "Function"=0, "Sweep Mode"=FALSE}, "Sweep Spacing"=0, "Range"=0, "SMU1 - Sampling"={"Source"=10.0, "Compliance"=1e-05, "Mode"=0, "Function"=FALSE}, "SMU2 - Sampling"={"Source"=10.0, "Compliance"=1e-05, "Mode"=0, "Function"=FALSE}, "SMU3 - Sampling"={"Source"=10.0, "Compliance"=1e-05, "Mode"=0, "Function"=FALSE}, "SMU4 - Sampling"={"Source"=10.0, "Compliance"=1e-05, "Mode"=0, "Function"=FALSE}, "Sampling Time Parameters"={"Initial Interval (s)"=0.1, "Number of Samples"=60, "Total Sampling Time (s)"=10.0, "Hold Time (s)"=0.0, "Sampling Mode"=0, "Sampling Time"=0}, "Stop Condition"={"Enable Delay (s)"=0.0, "Name"="", "Threshold"=0.0, "num. of events"=1, "Event"=0, "Stop Condition Enable"=FALSE}} ("HP4155C Configuration"), "SMU 1 - Sweeping"=w495, "SMU 2 - Sweeping"=w496, "SMU 3 - Sweeping"=w497, "SMU 4 - Sweeping"=w498, "Sweep Spacing"=w499, "Range"=w489) -> (w488:T33)
        n246 = Unbundle By Name(w490) -> ("Parameter Analyzer"=w493:refnum<queue>)
        n247 = call "Enqueue Message (Single).vi"("error in (no error)"=w492, "Message Data"=w488, "Message"="Configure Sweeping", "Message Queue"=w493) -> ("error out"=w491:errorcluster)  [unwired: 7 out]
      }
      frame "Parameter Analyzer - Configure Sampling" {
        n248 = Variant To Data(error in=w519, type=T78 {"SMU1 - Sampling"={"Source"=0.0, "Compliance"=0.0, "Mode"=0, "Function"=FALSE}, "SMU2 - Sampling"={"Source"=0.0, "Compliance"=0.0, "Mode"=0, "Function"=FALSE}, "SMU3 - Sampling"={"Source"=0.0, "Compliance"=0.0, "Mode"=0, "Function"=FALSE}, "SMU4 - Sampling"={"Source"=0.0, "Compliance"=0.0, "Mode"=0, "Function"=FALSE}, "Sampling Parameters"={"Initial Interval (s)"=0.0, "Number of Samples"=0, "Total Sampling Time (s)"=0.0, "Hold Time (s)"=0.0, "Sampling Mode"=0, "Sampling Time"=0}, "Stop Condition"={"Enable Delay (s)"=0.0, "Name"="", "Threshold"=0.0, "num. of events"=0, "Event"=0, "Stop Condition Enable"=FALSE}} ("output cluster"), Variant=w518) -> (data=w517:T78, error out=w512:errorcluster)
        n249 = Unbundle By Name(w517) -> ("SMU1 - Sampling"=w508:T12, "SMU2 - Sampling"=w507:T12, "SMU3 - Sampling"=w506:T12, "SMU4 - Sampling"=w505:T12, "Sampling Parameters"=w516:T14, "Stop Condition"=w515:T13)
        n250 = Bundle By Name(cluster=T33 {"Parameter Analyzer VISA Session"="COM1", "Sweeping Time Parameters"={"Integration Time"=0, "Short Integration Time (s)"=0.0, "Long Integration Time (s)"=0.0, "Wait Time Parameter"=1.0}, "Acquisition Mode"=enum."Sweeping Mode", "Status Polling Time (ms)"=1000, "Comment"="Test VI", "SMU 1 - Sweeping"={"Start / Offset"=0.0, "Stop / Ratio"=1.0, "Step \n(linear only)"=0.01, "Compliance"=0.1, "Power \nCompliance"=0.0, "Mode"=0, "Function"=0, "Sweep Mode"=FALSE}, "SMU 2 - Sweeping"={"Start / Offset"=0.0, "Stop / Ratio"=1.0, "Step \n(linear only)"=0.01, "Compliance"=0.1, "Power \nCompliance"=0.0, "Mode"=0, "Function"=0, "Sweep Mode"=FALSE}, "SMU 3 - Sweeping"={"Start / Offset"=0.0, "Stop / Ratio"=1.0, "Step \n(linear only)"=0.01, "Compliance"=0.1, "Power \nCompliance"=0.0, "Mode"=0, "Function"=0, "Sweep Mode"=FALSE}, "SMU 4 - Sweeping"={"Start / Offset"=0.0, "Stop / Ratio"=1.0, "Step \n(linear only)"=0.01, "Compliance"=0.1, "Power \nCompliance"=0.0, "Mode"=1, "Function"=0, "Sweep Mode"=FALSE}, "Sweep Spacing"=0, "Range"=0, "SMU1 - Sampling"={"Source"=10.0, "Compliance"=1e-05, "Mode"=0, "Function"=FALSE}, "SMU2 - Sampling"={"Source"=10.0, "Compliance"=1e-05, "Mode"=0, "Function"=FALSE}, "SMU3 - Sampling"={"Source"=10.0, "Compliance"=1e-05, "Mode"=0, "Function"=FALSE}, "SMU4 - Sampling"={"Source"=10.0, "Compliance"=1e-05, "Mode"=0, "Function"=FALSE}, "Sampling Time Parameters"={"Initial Interval (s)"=0.1, "Number of Samples"=60, "Total Sampling Time (s)"=10.0, "Hold Time (s)"=0.0, "Sampling Mode"=0, "Sampling Time"=0}, "Stop Condition"={"Enable Delay (s)"=0.0, "Name"="", "Threshold"=0.0, "num. of events"=1, "Event"=0, "Stop Condition Enable"=FALSE}} ("HP4155C Configuration"), "SMU1 - Sampling"=w508, "SMU2 - Sampling"=w507, "SMU3 - Sampling"=w506, "SMU4 - Sampling"=w505, "Sampling Time Parameters"=w516, "Stop Condition"=w515) -> (w509:T33)
        n251 = Unbundle By Name(w510) -> ("Parameter Analyzer"=w513:refnum<queue>)
        n252 = call "Enqueue Message (Single).vi"("error in (no error)"=w512, "Message Data"=w509, "Message"="Configure Sampling", "Message Queue"=w513) -> ("error out"=w511:errorcluster)  [unwired: 7 out]
      }
      frame "Parameter Analyzer - Measure" {
        n253 = Bundle By Name(cluster=T33 {"Parameter Analyzer VISA Session"="COM1", "Sweeping Time Parameters"={"Integration Time"=0, "Short Integration Time (s)"=0.0, "Long Integration Time (s)"=0.0, "Wait Time Parameter"=1.0}, "Acquisition Mode"=enum."Sweeping Mode", "Status Polling Time (ms)"=1000, "Comment"="Test VI", "SMU 1 - Sweeping"={"Start / Offset"=0.0, "Stop / Ratio"=1.0, "Step \n(linear only)"=0.01, "Compliance"=0.1, "Power \nCompliance"=0.0, "Mode"=0, "Function"=0, "Sweep Mode"=FALSE}, "SMU 2 - Sweeping"={"Start / Offset"=0.0, "Stop / Ratio"=1.0, "Step \n(linear only)"=0.01, "Compliance"=0.1, "Power \nCompliance"=0.0, "Mode"=0, "Function"=0, "Sweep Mode"=FALSE}, "SMU 3 - Sweeping"={"Start / Offset"=0.0, "Stop / Ratio"=1.0, "Step \n(linear only)"=0.01, "Compliance"=0.1, "Power \nCompliance"=0.0, "Mode"=0, "Function"=0, "Sweep Mode"=FALSE}, "SMU 4 - Sweeping"={"Start / Offset"=0.0, "Stop / Ratio"=1.0, "Step \n(linear only)"=0.01, "Compliance"=0.1, "Power \nCompliance"=0.0, "Mode"=1, "Function"=0, "Sweep Mode"=FALSE}, "Sweep Spacing"=0, "Range"=0, "SMU1 - Sampling"={"Source"=10.0, "Compliance"=1e-05, "Mode"=0, "Function"=FALSE}, "SMU2 - Sampling"={"Source"=10.0, "Compliance"=1e-05, "Mode"=0, "Function"=FALSE}, "SMU3 - Sampling"={"Source"=10.0, "Compliance"=1e-05, "Mode"=0, "Function"=FALSE}, "SMU4 - Sampling"={"Source"=10.0, "Compliance"=1e-05, "Mode"=0, "Function"=FALSE}, "Sampling Time Parameters"={"Initial Interval (s)"=0.1, "Number of Samples"=60, "Total Sampling Time (s)"=10.0, "Hold Time (s)"=0.0, "Sampling Mode"=0, "Sampling Time"=0}, "Stop Condition"={"Enable Delay (s)"=0.0, "Name"="", "Threshold"=0.0, "num. of events"=1, "Event"=0, "Stop Condition Enable"=FALSE}} ("HP4155C Configuration"), "Status Polling Time (ms)"="Status Polling Time (ms)") -> (w521:T33)
        n254 = Unbundle By Name(w524) -> ("Parameter Analyzer"=w526:refnum<queue>)
        n255 = call "Enqueue Message (Single).vi"("error in (no error)"=w523, "Message Data"=w521, "Message"="Measure", "Message Queue"=w526) -> ("error out"=w525:errorcluster)  [unwired: 7 out]
      }
      frame "Parameter Analyzer - Save Measurement" {
        n256 = Unbundle By Name(w529) -> ("Parameter Analyzer"=w531:refnum<queue>)
        n257 = call "Enqueue Message (Single).vi"("error in (no error)"=w528, "Message"="Save Electrical Measurement", "Message Queue"=w531) -> ("error out"=w530:errorcluster)  [unwired: 1 in, 7 out]
      }
      frame "----- Switching Matrix Events ----- " {
        # "Switching Matrix Events"
      }
      frame "Switching Matrix - Set UI" {
        n258 = Variant To Data(error in=w540, type=T41 {"Switching Matrix VISA Session"="GPIB0::18::INSTR", "Connections"=[{"Connections"=[FALSE, FALSE, FALSE, FALSE, FALSE, FALSE, FALSE, FALSE, FALSE, FALSE, FALSE, FALSE], "Connection Type"=enum."Disconnected"}, {"Connections"=[FALSE, FALSE, FALSE, FALSE, FALSE, FALSE, FALSE, FALSE, FALSE, FALSE, FALSE, FALSE], "Connection Type"=enum."Disconnected"}, {"Connections"=[FALSE, FALSE, FALSE, FALSE, FALSE, FALSE, FALSE, FALSE, FALSE, FALSE, FALSE, FALSE], "Connection Type"=enum."Disconnected"}, {"Connections"=[FALSE, FALSE, FALSE, FALSE, FALSE, FALSE, FALSE, FALSE, FALSE, FALSE, FALSE, FALSE], "Connection Type"=enum."Disconnected"}, {"Connections"=[FALSE, FALSE, FALSE, FALSE, FALSE, FALSE, FALSE, FALSE, FALSE, FALSE, FALSE, FALSE], "Connection Type"=enum."Disconnected"}, {"Connections"=[FALSE, FALSE, FALSE, FALSE, FALSE, FALSE, FALSE, FALSE, FALSE, FALSE, FALSE, FALSE], "Connection Type"=enum."Disconnected"}, {"Connections"=[FALSE, FALSE, FALSE, FALSE, FALSE, FALSE, FALSE, FALSE, FALSE, FALSE, FALSE, FALSE], "Connection Type"=enum."Disconnected"}, {"Connections"=[FALSE, FALSE, FALSE, FALSE, FALSE, FALSE, FALSE, FALSE, FALSE, FALSE, FALSE, FALSE], "Connection Type"=enum."Disconnected"}]} ("Keythley 707A Switching Matrix Configuration"), Variant=w536) -> (data=w535:T41, error out=w537:errorcluster)
        n259 = Unbundle By Name(w535) -> ("Switching Matrix VISA Session"=w539:refnum<visa-resource-name>, "Connections"=w538:T16)
        n260 = property on="Switching Matrix VISA Session" class="VISAName"("Value"=w539) -> ()  [unwired: 2 in, 2 out]
        n261 = property on="Switching Matrix Connections" class="Arr (strict)"("Value"=w538) -> ()  [unwired: 2 in, 2 out]
      }
      frame "Switching Matrix - Update Visa Session" {
        w541 = T41 {"Switching Matrix VISA Session"="GPIB0::18::INSTR", "Connections"=[{"Connections"=[FALSE, FALSE, FALSE, FALSE, FALSE, FALSE, FALSE, FALSE, FALSE, FALSE, FALSE, FALSE], "Connection Type"=enum."Disconnected"}, {"Connections"=[FALSE, FALSE, FALSE, FALSE, FALSE, FALSE, FALSE, FALSE, FALSE, FALSE, FALSE, FALSE], "Connection Type"=enum."Disconnected"}, {"Connections"=[FALSE, FALSE, FALSE, FALSE, FALSE, FALSE, FALSE, FALSE, FALSE, FALSE, FALSE, FALSE], "Connection Type"=enum."Disconnected"}, {"Connections"=[FALSE, FALSE, FALSE, FALSE, FALSE, FALSE, FALSE, FALSE, FALSE, FALSE, FALSE, FALSE], "Connection Type"=enum."Disconnected"}, {"Connections"=[FALSE, FALSE, FALSE, FALSE, FALSE, FALSE, FALSE, FALSE, FALSE, FALSE, FALSE, FALSE], "Connection Type"=enum."Disconnected"}, {"Connections"=[FALSE, FALSE, FALSE, FALSE, FALSE, FALSE, FALSE, FALSE, FALSE, FALSE, FALSE, FALSE], "Connection Type"=enum."Disconnected"}, {"Connections"=[FALSE, FALSE, FALSE, FALSE, FALSE, FALSE, FALSE, FALSE, FALSE, FALSE, FALSE, FALSE], "Connection Type"=enum."Disconnected"}, {"Connections"=[FALSE, FALSE, FALSE, FALSE, FALSE, FALSE, FALSE, FALSE, FALSE, FALSE, FALSE, FALSE], "Connection Type"=enum."Disconnected"}]} ("Keythley 707A Switching Matrix Configuration")
        n262 = Unbundle By Name(w541) -> ("Switching Matrix VISA Session"=w542:refnum<visa-resource-name>)
        n263 = Variant To Data(error in=w548, type=w542, Variant=w545) -> (data=w544:refnum<visa-resource-name>, error out=w546:errorcluster)
        n264 = Bundle By Name(cluster=w541, "Switching Matrix VISA Session"=w544) -> (w543:T41)
        n265 = Unbundle By Name(w549) -> ("Switching Matrix"=w550:refnum<queue>)
        n266 = call "Enqueue Message (Single).vi"("error in (no error)"=w546, "Message Data"=w543, "Message"="Update Visa Session", "Message Queue"=w550) -> ("error out"=w551:errorcluster)  [unwired: 7 out]
      }
      frame "Switching Matrix - Update Refnums" {
        n267 = control-ref of="Switching Matrix Connections"() -> (w555:refnum<vi>)
        n268 = control-ref of="Switching Matrix"() -> (w553:refnum<vi>)
        n269 = Bundle By Name(cluster=T79 {"Connections"=refnum, "Instrument Status"=refnum} ("Keythley 707A SwitchMatrix Refnums"), "Connections"=w555, "Instrument Status"=w553) -> (w554:T79)
        n270 = Unbundle By Name(w558) -> ("Switching Matrix"=w559:refnum<queue>)
        n271 = call "Enqueue Message (Single).vi"("error in (no error)"=w557, "Message Data"=w554, "Message"="Update Refnums", "Message Queue"=w559) -> ("error out"=w560:errorcluster)  [unwired: 7 out]
      }
      frame "Switching Matrix - Set Connections" {
        w561 = T41 {"Switching Matrix VISA Session"="GPIB0::18::INSTR", "Connections"=[{"Connections"=[FALSE, FALSE, FALSE, FALSE, FALSE, FALSE, FALSE, FALSE, FALSE, FALSE, FALSE, FALSE], "Connection Type"=enum."Disconnected"}, {"Connections"=[FALSE, FALSE, FALSE, FALSE, FALSE, FALSE, FALSE, FALSE, FALSE, FALSE, FALSE, FALSE], "Connection Type"=enum."Disconnected"}, {"Connections"=[FALSE, FALSE, FALSE, FALSE, FALSE, FALSE, FALSE, FALSE, FALSE, FALSE, FALSE, FALSE], "Connection Type"=enum."Disconnected"}, {"Connections"=[FALSE, FALSE, FALSE, FALSE, FALSE, FALSE, FALSE, FALSE, FALSE, FALSE, FALSE, FALSE], "Connection Type"=enum."Disconnected"}, {"Connections"=[FALSE, FALSE, FALSE, FALSE, FALSE, FALSE, FALSE, FALSE, FALSE, FALSE, FALSE, FALSE], "Connection Type"=enum."Disconnected"}, {"Connections"=[FALSE, FALSE, FALSE, FALSE, FALSE, FALSE, FALSE, FALSE, FALSE, FALSE, FALSE, FALSE], "Connection Type"=enum."Disconnected"}, {"Connections"=[FALSE, FALSE, FALSE, FALSE, FALSE, FALSE, FALSE, FALSE, FALSE, FALSE, FALSE, FALSE], "Connection Type"=enum."Disconnected"}, {"Connections"=[FALSE, FALSE, FALSE, FALSE, FALSE, FALSE, FALSE, FALSE, FALSE, FALSE, FALSE, FALSE], "Connection Type"=enum."Disconnected"}]} ("Keythley 707A Switching Matrix Configuration")
        n272 = Unbundle By Name(w561) -> ("Connections"=w562:T16)
        n273 = Variant To Data(error in=w568, type=w562, Variant=w565) -> (data=w564:T16, error out=w566:errorcluster)
        n274 = Bundle By Name(cluster=w561, "Connections"=w564) -> (w563:T41)
        n275 = Unbundle By Name(w569) -> ("Switching Matrix"=w570:refnum<queue>)
        n276 = call "Enqueue Message (Single).vi"("error in (no error)"=w566, "Message Data"=w563, "Message"="Set Connections", "Message Queue"=w570) -> ("error out"=w571:errorcluster)  [unwired: 7 out]
      }
      frame "Switching Matrix - Disconnect All" {
        n277 = Unbundle By Name(w574) -> ("Switching Matrix"=w575:refnum<queue>)
        n278 = call "Enqueue Message (Single).vi"("error in (no error)"=w572, "Message"="Disconnect All", "Message Queue"=w575) -> ("error out"=w576:errorcluster)  [unwired: 1 in, 7 out]
      }
      frame "Switching Matrix - Ground All" {
        n279 = Unbundle By Name(w579) -> ("Switching Matrix"=w580:refnum<queue>)
        n280 = call "Enqueue Message (Single).vi"("error in (no error)"=w577, "Message"="Ground All", "Message Queue"=w580) -> ("error out"=w581:errorcluster)  [unwired: 1 in, 7 out]
      }
      frame "----- XYZ Stage Events -----" {
        # "NEW DEVICE EVENTS"
      }
      frame "XYZ Stage - Update Visa Session" {
        w583 = T55 {"Connection Settings"={"Tango VISA"="", "Baudrate"=57600, "Show Protocol?"=FALSE}, "Manual Control"={"North"=FALSE, "South"=FALSE, "West"=FALSE, "East"=FALSE, "Up"=FALSE, "Down"=FALSE, "Stop"=FALSE, "XY Step"=0.0, "Z step"=0.0}, "Coordinate Control"={"Motion Mode"=enum."Absolute", "Destination [mm]"=[]}} ("Configuration")
        n281 = Unbundle By Name(w583) -> ("Connection Settings.Tango VISA"=w591:refnum<visa-resource-name>)
        n282 = Variant To Data(error in=w593, type=w591, Variant=w592) -> (data=w584:refnum<visa-resource-name>, error out=w589:errorcluster)
        n283 = Bundle By Name(cluster=w583, "Connection Settings.Tango VISA"=w584) -> (w585:T55)
        n284 = Unbundle By Name(w587) -> ("XYZ Stage"=w586:refnum<queue>)
        n285 = call "Enqueue Message (Single).vi"("error in (no error)"=w589, "Message Data"=w585, "Message"="Manual Control", "Message Queue"=w586) -> ("error out"=w588:errorcluster)  [unwired: 7 out]
      }
      frame "XYZ Stage - Manual Control" {
        w595 = T55 {"Connection Settings"={"Tango VISA"="", "Baudrate"=57600, "Show Protocol?"=FALSE}, "Manual Control"={"North"=FALSE, "South"=FALSE, "West"=FALSE, "East"=FALSE, "Up"=FALSE, "Down"=FALSE, "Stop"=FALSE, "XY Step"=0.0, "Z step"=0.0}, "Coordinate Control"={"Motion Mode"=enum."Absolute", "Destination [mm]"=[]}} ("Configuration")
        n286 = Unbundle By Name(w595) -> ("Manual Control"=w594:T57)
        n287 = Variant To Data(error in=w604, type=w594, Variant=w603) -> (data=w596:T57, error out=w601:errorcluster)
        n288 = Bundle By Name(cluster=w595, "Manual Control"=w596) -> (w597:T55)
        n289 = Unbundle By Name(w599) -> ("XYZ Stage"=w598:refnum<queue>)
        n290 = call "Enqueue Message (Single).vi"("error in (no error)"=w601, "Message Data"=w597, "Message"="Manual Control", "Message Queue"=w598) -> ("error out"=w600:errorcluster)  [unwired: 7 out]
      }
      frame "----- AutoFocus Events -----" {
        # "NEW DEVICE EVENTS"
      }
      frame "AutoFocus - Set Match Criteria" {
        w606 = T59 {"Matching Criteria"={"Minimum Score"=700.0, "Color Score Weight"=57600.0, "Minimum Contrast"=50, "Match Mode"=0, "Match Feature Mode"=0, "Subpixel Accuracy"=TRUE, "Color Sensitivity"=1, "Search Strategy"=1}, "Z Scan Parameters"={"Z Range"=1380.0, "Resolution"=5000.0, "Initial Direction"=enum."Up", "Focus Threshold"=0.1, "Ascent Constant"=0.1}, "Displacement"=0.0, "Transformation Matrix"=[]} ("Configuration")
        n291 = Unbundle By Name(w606) -> ("Matching Criteria"=w614:T85)
        n292 = Variant To Data(error in=w616, type=w614, Variant=w615) -> (data=w607:T85, error out=w612:errorcluster)
        n293 = Bundle By Name(cluster=w606, "Matching Criteria"=w607) -> (w608:T59)
        n294 = Unbundle By Name(w610) -> ("AutoFocus"=w609:refnum<queue>)
        n295 = call "Enqueue Message (Single).vi"("error in (no error)"=w612, "Message Data"=w608, "Message"="Set Match Criteria", "Message Queue"=w609) -> ("error out"=w611:errorcluster)  [unwired: 7 out]
      }
      frame "AutoFocus - Link Stage & Camera" {
        w617 = T59 {"Matching Criteria"={"Minimum Score"=700.0, "Color Score Weight"=57600.0, "Minimum Contrast"=50, "Match Mode"=0, "Match Feature Mode"=0, "Subpixel Accuracy"=TRUE, "Color Sensitivity"=1, "Search Strategy"=1}, "Z Scan Parameters"={"Z Range"=1380.0, "Resolution"=5000.0, "Initial Direction"=enum."Up", "Focus Threshold"=0.1, "Ascent Constant"=0.1}, "Displacement"=0.0, "Transformation Matrix"=[]} ("Configuration")
        n296 = Unbundle By Name(w617) -> ("Displacement"=w625:dbl)
        n297 = Variant To Data(error in=w627, type=w625, Variant=w626) -> (data=w618:dbl, error out=w623:errorcluster)
        n298 = Bundle By Name(cluster=w617, "Displacement"=w618) -> (w619:T59)
        n299 = Unbundle By Name(w621) -> ("AutoFocus"=w620:refnum<queue>)
        n300 = call "Enqueue Message (Single).vi"("error in (no error)"=w623, "Message Data"=w619, "Message"="Link Stage & Camera", "Message Queue"=w620) -> ("error out"=w622:errorcluster)  [unwired: 7 out]
      }
      frame "AutoFocus - Focus" {
        w628 = T59 {"Matching Criteria"={"Minimum Score"=700.0, "Color Score Weight"=57600.0, "Minimum Contrast"=50, "Match Mode"=0, "Match Feature Mode"=0, "Subpixel Accuracy"=TRUE, "Color Sensitivity"=1, "Search Strategy"=1}, "Z Scan Parameters"={"Z Range"=1380.0, "Resolution"=5000.0, "Initial Direction"=enum."Up", "Focus Threshold"=0.1, "Ascent Constant"=0.1}, "Displacement"=0.0, "Transformation Matrix"=[]} ("Configuration")
        n301 = Unbundle By Name(w628) -> ("Z Scan Parameters"=w636:T60)
        n302 = Variant To Data(error in=w638, type=w636, Variant=w637) -> (data=w629:T60, error out=w634:errorcluster)
        n303 = Bundle By Name(cluster=w628, "Z Scan Parameters"=w629) -> (w630:T59)
        n304 = Unbundle By Name(w632) -> ("AutoFocus"=w631:refnum<queue>)
        n305 = call "Enqueue Message (Single).vi"("error in (no error)"=w634, "Message Data"=w630, "Message"="Focus", "Message Queue"=w631) -> ("error out"=w633:errorcluster)  [unwired: 7 out]
      }
      frame "AutoFocus - Set Target" {
        n306 = Unbundle By Name(w641) -> ("AutoFocus"=w640:refnum<queue>)
        n307 = call "Enqueue Message (Single).vi"("error in (no error)"=w639, "Message"="Set Target", "Message Queue"=w640) -> ("error out"=w642:errorcluster)  [unwired: 1 in, 7 out]
      }
      frame "AutoFocus - Find Target" {
        n308 = Unbundle By Name(w646) -> ("AutoFocus"=w645:refnum<queue>)
        n309 = call "Enqueue Message (Single).vi"("error in (no error)"=w644, "Message"="Find Target", "Message Queue"=w645) -> ("error out"=w647:errorcluster)  [unwired: 1 in, 7 out]
      }
      frame "AutoFocus - Align" {
        n310 = Unbundle By Name(w651) -> ("AutoFocus"=w650:refnum<queue>)
        n311 = call "Enqueue Message (Single).vi"("error in (no error)"=w649, "Message"="Align", "Message Queue"=w650) -> ("error out"=w652:errorcluster)  [unwired: 1 in, 7 out]
      }
      frame "AutoFocus - Grab Image" {
        n312 = Unbundle By Name(w656) -> ("AutoFocus"=w655:refnum<queue>)
        n313 = call "Enqueue Message (Single).vi"("error in (no error)"=w654, "Message"="Grab Image", "Message Queue"=w655) -> ("error out"=w657:errorcluster)  [unwired: 1 in, 7 out]
      }
      frame "AutoFocus - Set ROI" {
        n314 = Unbundle By Name(w661) -> ("AutoFocus"=w660:refnum<queue>)
        n315 = call "Enqueue Message (Single).vi"("error in (no error)"=w659, "Message"="Set ROI", "Message Queue"=w660) -> ("error out"=w662:errorcluster)  [unwired: 1 in, 7 out]
      }
      frame "AutoFocus - Get ROI" {
        n316 = Unbundle By Name(w666) -> ("AutoFocus"=w665:refnum<queue>)
        n317 = call "Enqueue Message (Single).vi"("error in (no error)"=w664, "Message"="Get ROI", "Message Queue"=w665) -> ("error out"=w667:errorcluster)  [unwired: 1 in, 7 out]
      }
      frame "AutoFocus - Start Tracking" {
        n318 = Unbundle By Name(w671) -> ("AutoFocus"=w670:refnum<queue>)
        n319 = call "Enqueue Message (Single).vi"("error in (no error)"=w669, "Message"="Start Tracking", "Message Queue"=w670) -> ("error out"=w672:errorcluster)  [unwired: 1 in, 7 out]
      }
      frame "AutoFocus - Stop Tracking" {
        n320 = Unbundle By Name(w676) -> ("AutoFocus"=w675:refnum<queue>)
        n321 = call "Enqueue Message (Single).vi"("error in (no error)"=w674, "Message"="Stop Tracking", "Message Queue"=w675) -> ("error out"=w677:errorcluster)  [unwired: 1 in, 7 out]
      }
      frame "----- Instrument Sequence Events -----" {
        # "NEW DEVICE EVENTS"
      }
      frame "Instrument Sequence - Update Refnums" {
        n322 = control-ref of="Strain Measurement - Steps"() -> (w681:refnum<vi>)
        n323 = control-ref of="Strain Measurement - Device ID"() -> (w683:refnum<vi>)
        n324 = control-ref of="Strain Measurement - Device Information"() -> (w682:refnum<vi>)
        n325 = control-ref of="Instrument Sequence - Pause"() -> (w684:refnum<vi>)
        n326 = Bundle By Name(cluster=T80 {"Instrument Steps"=refnum, "Instruments Status"=refnum, "Device ID"=refnum, "Device Information"=refnum, "Pause-Resume"=refnum, "Plot"={"Plot List"=refnum, "Voltage Plot"=refnum, "Current Plot"=refnum, "IV Characteristic"=refnum, "dI/dV-V Characteristic"=refnum}} ("Refnums"), "Instrument Steps"=w681, "Device ID"=w683, "Device Information"=w682, "Pause-Resume"=w684) -> (w685:T80)
        n327 = Unbundle By Name(w686) -> ("Instrument Sequence"=w689:refnum<queue>)
        n328 = call "Enqueue Message (Single).vi"("error in (no error)"=w687, "Message Data"=w685, "Message"="Update Refnums", "Message Queue"=w689) -> ("error out"=w688:errorcluster)  [unwired: 7 out]
      }
      frame "Instrument Sequence - Add Step" {
        n329 = Unbundle By Name(w695) -> ("Instrument Sequence"=w694:refnum<queue>)
        n330 = call "Enqueue Message (Single).vi"("error in (no error)"=w693, "Message"="Add Step", "Message Queue"=w694) -> ("error out"=w692:errorcluster)  [unwired: 1 in, 7 out]
      }
      frame "Instrument Sequence - Remove Step" {
        n331 = Unbundle By Name(w700) -> ("Instrument Sequence"=w699:refnum<queue>)
        n332 = call "Enqueue Message (Single).vi"("error in (no error)"=w698, "Message"="Remove Step", "Message Queue"=w699) -> ("error out"=w697:errorcluster)  [unwired: 1 in, 7 out]
      }
      frame "Instrument Sequence - Clear Sequence" {
        n333 = Unbundle By Name(w705) -> ("Instrument Sequence"=w704:refnum<queue>)
        n334 = call "Enqueue Message (Single).vi"("error in (no error)"=w703, "Message"="Clear Sequence", "Message Queue"=w704) -> ("error out"=w702:errorcluster)  [unwired: 1 in, 7 out]
      }
      frame "Instrument Sequence - Save Sequence" {
        n335 = Unbundle By Name(w710) -> ("Instrument Sequence"=w709:refnum<queue>)
        n336 = call "Enqueue Message (Single).vi"("error in (no error)"=w708, "Message"="Save Sequence", "Message Queue"=w709) -> ("error out"=w707:errorcluster)  [unwired: 1 in, 7 out]
      }
      frame "Instrument Sequence - Load Sequence" {
        n337 = Unbundle By Name(w715) -> ("Instrument Sequence"=w714:refnum<queue>)
        n338 = call "Enqueue Message (Single).vi"("error in (no error)"=w713, "Message"="Load Sequence", "Message Queue"=w714) -> ("error out"=w712:errorcluster)  [unwired: 1 in, 7 out]
      }
      frame "Instrument Sequence - Start Sequence" {
        n339 = Unbundle By Name(w720) -> ("Instrument Sequence"=w719:refnum<queue>)
        n340 = call "Enqueue Message (Single).vi"("error in (no error)"=w716, "Message"="Start Sequence", "Message Queue"=w719) -> ("error out"=w718:errorcluster)  [unwired: 1 in, 7 out]
      }
      frame "Instrument Sequence - Stop Sequence" {
        n341 = Unbundle By Name(w725) -> ("Instrument Sequence"=w724:refnum<queue>)
        n342 = call "Enqueue Message (Single).vi"("error in (no error)"=w721, "Message"="Measure Sequence", "Message Queue"=w724) -> ("error out"=w723:errorcluster)  [unwired: 1 in, 7 out]
      }
      frame "Instrument Sequence - Pause Sequence" {
        n343 = Unbundle By Name(w730) -> ("Instrument Sequence"=w729:refnum<queue>)
        n344 = call "Enqueue Message (Single).vi"("error in (no error)"=w726, "Message"="Pause Sequence", "Message Queue"=w729) -> ("error out"=w728:errorcluster)  [unwired: 1 in, 7 out]
      }
      frame "----- StrainElectrical Measurement Events -----" {
        # "NEW DEVICE EVENTS"
      }
      frame "Strain Measurement - Set UI" {
        n345 = Variant To Data(error in=w737, type=T71 {"Stress Sequence "={"Max Motor Position"=1380.0, "# Intermediate Points"=5000, "Initial Direction"=enum."Tension"}, "Track?"=FALSE} ("Strain Measurement"), Variant=w735) -> (data=w734:T71, error out=w736:errorcluster)
        n346 = Unbundle By Name(w734) -> ("Stress Sequence"=w733:T86)
        n347 = property on="Strain Measurement - Stress Sequence Parameters" class="Clust (strict)"("Value"=w733) -> ()  [unwired: 2 in, 2 out]
      }
      frame "Strain Measurement - Update Refnums" {
        n348 = control-ref of="Strain Measurement - Steps"() -> (w743:refnum<vi>)
        n349 = control-ref of="Strain Measurement - Sequence Progress"() -> (w742:refnum<vi>)
        n350 = control-ref of="Strain Measurement - Device ID"() -> (w741:refnum<vi>)
        n351 = control-ref of="Strain Measurement - Device Information"() -> (w740:refnum<vi>)
        n352 = control-ref of="Strain Measurement - Pause"() -> (w739:refnum<vi>)
        n353 = Bundle By Name(cluster=T81 {"Instrument Steps"=refnum, "Sequence Progress"=refnum, "Device ID"=refnum, "Device Information"=refnum, "Pause-Resume"=refnum, "Track"=refnum, "Plot"={"Plot List"=refnum, "Voltage Plot"=refnum, "Current Plot"=refnum, "IV Characteristic"=refnum, "dI/dV-V Characteristic"=refnum}} ("Strain-Electrical Measurement Refnums"), "Instrument Steps"=w743, "Sequence Progress"=w742, "Device ID"=w741, "Device Information"=w740, "Pause-Resume"=w739) -> (w744:T81)
        n354 = Unbundle By Name(w747) -> ("Strain Measurement"=w749:refnum<queue>)
        n355 = call "Enqueue Message (Single).vi"("error in (no error)"=w746, "Message Data"=w744, "Message"="Update Refnums", "Message Queue"=w749) -> ("error out"=w745:errorcluster)  [unwired: 7 out]
      }
      frame "Strain Measurement - Update Strain Sequence" {
        w750 = T71 {"Stress Sequence "={"Max Motor Position"=1380.0, "# Intermediate Points"=5000, "Initial Direction"=enum."Tension"}, "Track?"=FALSE} ("Strain Measurement")
        n356 = Unbundle By Name(w750) -> ("Stress Sequence"=w751:T86)
        n357 = Variant To Data(error in=w760, type=w751, Variant=w759) -> (data=w753:T86, error out=w758:errorcluster)
        n358 = Bundle By Name(cluster=w750, "Stress Sequence"=w753) -> (w752:T71)
        n359 = Unbundle By Name(w754) -> ("Strain Measurement"=w755:refnum<queue>)
        n360 = call "Enqueue Message (Single).vi"("error in (no error)"=w758, "Message Data"=w752, "Message"="Define Strain Sequence", "Message Queue"=w755) -> ("error out"=w757:errorcluster)  [unwired: 7 out]
      }
      frame "Strain Measurement - Start" {
        n361 = Unbundle By Name(w761) -> ("Strain Measurement"=w762:refnum<queue>)
        n362 = call "Enqueue Message (Single).vi"("error in (no error)"=w765, "Message"="Start Strain Measurement", "Message Queue"=w762) -> ("error out"=w764:errorcluster)  [unwired: 1 in, 7 out]
      }
      frame "Strain Measurement - Pause" {
        n363 = Unbundle By Name(w766) -> ("Strain Measurement"=w767:refnum<queue>)
        n364 = call "Enqueue Message (Single).vi"("error in (no error)"=w770, "Message"="Pause", "Message Queue"=w767) -> ("error out"=w769:errorcluster)  [unwired: 1 in, 7 out]
      }
      frame "Strain Measurement - Stop" {
        n365 = Unbundle By Name(w771) -> ("Strain Measurement"=w772:refnum<queue>)
        n366 = call "Enqueue Message (Single).vi"("error in (no error)"=w775, "Message"="Stop", "Message Queue"=w772) -> ("error out"=w774:errorcluster)  [unwired: 1 in, 7 out]
      }
      frame "Strain Measurement - New Sequence" {
        n367 = Unbundle By Name(w780) -> ("Strain Measurement"=w779:refnum<queue>)
        n368 = call "Enqueue Message (Single).vi"("error in (no error)"=w778, "Message"="Clear Instrument Sequence", "Message Queue"=w779) -> ("error out"=w777:errorcluster)  [unwired: 1 in, 7 out]
      }
      frame "Strain Measurement - Add Step" {
        n369 = Unbundle By Name(w785) -> ("Strain Measurement"=w784:refnum<queue>)
        n370 = call "Enqueue Message (Single).vi"("error in (no error)"=w783, "Message"="Add Instrument Sequence Step", "Message Queue"=w784) -> ("error out"=w782:errorcluster)  [unwired: 1 in, 7 out]
      }
      frame "Strain Measurement - Delete Step" {
        n371 = Unbundle By Name(w790) -> ("Strain Measurement"=w789:refnum<queue>)
        n372 = call "Enqueue Message (Single).vi"("error in (no error)"=w788, "Message"="Delete Instrument Sequence Step", "Message Queue"=w789) -> ("error out"=w787:errorcluster)  [unwired: 1 in, 7 out]
      }
      frame "Strain Measurement - Save Sequence" {
        n373 = Unbundle By Name(w795) -> ("Strain Measurement"=w794:refnum<queue>)
        n374 = call "Enqueue Message (Single).vi"("error in (no error)"=w793, "Message"="Save Instrument Sequence", "Message Queue"=w794) -> ("error out"=w792:errorcluster)  [unwired: 1 in, 7 out]
      }
      frame "Strain Measurement - Load Sequence" {
        n375 = Unbundle By Name(w800) -> ("Strain Measurement"=w799:refnum<queue>)
        n376 = call "Enqueue Message (Single).vi"("error in (no error)"=w798, "Message"="Load Instrument Sequence", "Message Queue"=w799) -> ("error out"=w797:errorcluster)  [unwired: 1 in, 7 out]
      }
      frame "----- PlotData Events -----" {
        # "NEW DEVICE EVENTS"
      }
      frame "PlotData - Set UI" {
        n377 = Variant To Data(error in=w808, type=T66 {"Sliders"={"Strain Sequence"=0, "Instrument Sequence"=0}, "Measurement"={"Which Instrument?"=enum."No Plot", "Electrical Measurement"={"Sequence"=[], "V1"=[], "V2"=[], "V3"=[], "V4"=[], "I1"=[], "I2"=[], "I3"=[], "I4"=[]}, "Measurement Mode"=enum."Sweeping Mode", "Optical Spectrum"={"Intensity"=[], "Wavelength"=[], "Energy"=[], "Raman Shift"=[], "Detector Temperature"=0.0}}, "Instrument Steps"=[], "Strain Points"=[]} ("PlotData Configuration"), Variant=w806) -> (data=w805:T66, error out=w807:errorcluster)
        n378 = Unbundle By Name(w805) -> ("Sliders.Strain Sequence"=w804:i32, "Sliders.Instrument Sequence"=w803:i32)
        n379 = property on="PlotData - Strain Sequence" class="Slide (strict)"("Value"=w804) -> ()  [unwired: 2 in, 2 out]
        n380 = property on="PlotData - Instrument Sequence" class="Slide (strict)"("Value"=w803) -> ()  [unwired: 2 in, 2 out]
      }
      frame "PlotData - Update Refnums" {
        n381 = control-ref of="PlotData - Choose Plot"() -> (w815:refnum<vi>)
        n382 = control-ref of="PlotData - Instrument Sequence"() -> (w818:refnum<vi>)
        n383 = control-ref of="PlotData - Strain Sequence"() -> (w817:refnum<vi>)
        n384 = control-ref of="PlotData - Configuration"() -> (w816:refnum<vi>)
        n385 = control-ref of="PlotData - Electrical Plot List"() -> (w814:refnum<vi>)
        n386 = control-ref of="PlotData - Voltage Plot"() -> (w813:refnum<vi>)
        n387 = control-ref of="PlotData - Current Plot"() -> (w812:refnum<vi>)
        n388 = control-ref of="PlotData - dI/dV-V Characteristic"() -> (w811:refnum<vi>)
        n389 = control-ref of="PlotData - IV Characteristic"() -> (w810:refnum<vi>)
        n390 = Bundle By Name(cluster=T82 {"Choose Plot"=refnum, "Instrument Sequence"=refnum, "Strain Sequence"=refnum, "Configuration"=refnum, "Electrical Data Plot"={"Plot List"=refnum, "Voltage Plot"=refnum, "Current Plot"=refnum, "IV Characteristic"=refnum, "dI/dV-V Characteristic"=refnum}, "Optical Spectrum Plot"={"Plot List"=refnum, "Optical Spectrum vs Energy"=refnum, "Optical Spectrum vs Wavelength"=refnum, "Optical Spectrum vs Raman Shift"=refnum, "Detector Temperature"=refnum}, "Optoelectronic Plot"={"Optical Spectrum Plot"={"Plot List"=refnum, "Optical Spectrum vs Energy"=refnum, "Optical Spectrum vs Wavelength"=refnum, "Optical Spectrum vs Raman Shift"=refnum, "Detector Temperature"=refnum}, "Electrical Data Plot"={"Plot List"=refnum, "Voltage Plot"=refnum, "Current Plot"=refnum, "IV Characteristic"=refnum, "dI/dV-V Characteristic"=refnum}}} ("All Plot Refnums"), "Choose Plot"=w815, "Instrument Sequence"=w818, "Strain Sequence"=w817, "Configuration"=w816, "Electrical Data Plot.Plot List"=w814, "Electrical Data Plot.Voltage Plot"=w813, "Electrical Data Plot.Current Plot"=w812, "Electrical Data Plot.IV Characteristic"=w810, "Electrical Data Plot.dI/dV-V Characteristic"=w811) -> (w819:T82)
        n391 = Unbundle By Name(w822) -> ("Plot Data"=w823:refnum<queue>)
        n392 = call "Enqueue Message (Single).vi"("error in (no error)"=w821, "Message Data"=w819, "Message"="Update Refnums", "Message Queue"=w823) -> ("error out"=w824:errorcluster)  [unwired: 7 out]
      }
      frame "PlotData - Update Plots" {
        n393 = Variant To Data(error in=w837, type=T83 {"PlotData - Instrument Sequence"=0, "PlotData - Strain Sequence"=0} ("output cluster"), Variant=w836) -> (data=w828:T83, error out=w833:errorcluster)
        n394 = Unbundle By Name(w828) -> ("PlotData - Strain Sequence"=w827:i32, "PlotData - Instrument Sequence"=w826:i32)
        n395 = Bundle By Name(cluster=T66 {"Sliders"={"Strain Sequence"=0, "Instrument Sequence"=0}, "Measurement"={"Which Instrument?"=enum."No Plot", "Electrical Measurement"={"Sequence"=[], "V1"=[], "V2"=[], "V3"=[], "V4"=[], "I1"=[], "I2"=[], "I3"=[], "I4"=[]}, "Measurement Mode"=enum."Sweeping Mode", "Optical Spectrum"={"Intensity"=[], "Wavelength"=[], "Energy"=[], "Raman Shift"=[], "Detector Temperature"=0.0}}, "Instrument Steps"=[], "Strain Points"=[]} ("PlotData Configuration"), "Sliders.Strain Sequence"=w827, "Sliders.Instrument Sequence"=w826) -> (w830:T66)
        n396 = Unbundle By Name(w831) -> ("Plot Data"=w834:refnum<queue>)
        n397 = call "Enqueue Message (Single).vi"("error in (no error)"=w833, "Message Data"=w830, "Message"="Plot Data", "Message Queue"=w834) -> ("error out"=w832:errorcluster)  [unwired: 7 out]
      }
      frame "----- Save Data Events -----" {
        # "Save Data Events"
      }
    }
    n398 = call "Message Handling Loop.vi"("error in (no error)"=w40, "Message Queue"=w38) -> ("dup error in"=w39:errorcluster)  [unwired: 9 out]
  }
  n399 = while "Event Handling Loop" {
    tunnel: w31 -> [w845]
    tunnel: [w844] -> w30
    tunnel: w29 -> [w842]
    tunnel: [w840] -> w28
    stop <- w839 stop-if-true
    n400 = event shown="[16] \"Switching Matrix VISA Session\": Value Change" {
      selector: w845 -> [_ _ _ _ _ _ _ _ _ _ _ _ _ _ _ _ _ _ _ _ _ _ _ _ _ _ _ _ _ _ _ _ _]
      dyn-events: [_ _ _ _ _ _ _ _ _ _ _ _ _ _ _ _ _ _ _ _ _ _ _ _ _ _ _ _ _ _ _ _ _] -> w840
      timeout: _ -> [_ _ _ _ _ _ _ _ _ _ _ _ _ _ _ _ _ _ _ _ _ _ _ _ _ _ _ _ _ _ _ _ _]
      tunnel: [w851 _ _ w869 w875 w880 w887 w889 _ w896 w902 w913 w924 w929 w933 w936 w941 w946 w950 w954 w958 w962 w966 w978 w982 w986 w990 w994 w998 w1002 w1006 w1010 w1017] -> w843
      tunnel: w842 -> [w852 w861 w866 w872 w877 w882 w885 w891 w892 w894 w900 w911 w922 w927 w931 w935 w939 w944 w948 w952 w957 w961 w965 w976 w980 w984 w988 w992 w996 w1000 w1004 w1008 w1015]
      tunnel: [w850 w861 w866 w871 w876 w881 w886 w890 w892 w895 w901 w912 w923 w928 w932 w937 w940 w945 w949 w953 w959 w963 w967 w977 w981 w985 w989 w993 w997 w1001 w1005 w1009 w1016] -> w841
      tunnel: [_ _ TRUE ("Priority Message? (F)") _ _ _ _ _ _ _ _ _ _ _ _ _ _ _ _ _ _ _ _ _ _ _ _ _ _ _ _ _ _] -> w839
      event Panel Close? {
        # "Send the \"Confirm Quit\" message if the user closes the panel of the VI. Discard the event so the \"Confirm Quit\" message has a chance to run."
        n401 = event-data() -> ()  [unwired: 2 out]
        n402 = Two Button Dialog(message="Do you really want to quit Swissknife?", 1:"No" ("F button name (\"Cancel\")"), 2:"Yes" ("T button name (\"OK\")")) -> (T button?=w846:bool)
        n403 = case shown="False" w846 {
          tunnel: w852 -> [w855 w860]
          tunnel: [errorcluster {"status"=FALSE, "code"=0, "source"=""} ("error out") w857] -> w851
          tunnel: [w855 w856] -> w850
          frame False {
          }
          frame True {
            n404 = call "Enqueue Message (Single).vi"("Priority Message? (F)"=TRUE, "Message"="Initiate Exit", "Message Queue"=w860) -> ("error out"=w857:errorcluster, "dup Message Queue"=w856:refnum<queue>)  [unwired: 2 in, 5 out]
          }
        }
        n405 = event-data("Discard?"=TRUE) -> ()  [unwired: 1 in, 1 out]
      }
      event Application Instance Close {
        # "#CodeRecommended - When a project closes, all VIs within that project are aborted and leave memory. However, any code placed in this event frame is guaranteed to run to completion, so add any cleanup code that absolutely must happen here."
        n406 = event-data() -> ()  [unwired: 2 out]
      }
      event User Event {
        n407 = event-data() -> ()  [unwired: 2 out]
        n408 = call "Status String.vi"("Message"="Program Terminated" ("Display <Replace Me>")) -> ("Status String"=w862:string)
        n409 = property on="Status Log" class="Str"() -> ("Value"=w864:string)  [unwired: 2 in, 2 out]
        n410 = Concatenate Strings(w862, w864) -> (w865:string)
        n411 = property on="Status Log" class="Str"("Value"=w865) -> ()  [unwired: 2 in, 2 out]
      }
      event "Stress Controller VISA Session": Value Change {
        n412 = event-data() -> ()  [unwired: 2 out]
        n413 = call "Enqueue Message (Single).vi"("Message Data"="Stress Controller VISA Session", "Message"="Stress Control - Update VISA Session", "Message Queue"=w872) -> ("error out"=w869:errorcluster, "dup Message Queue"=w871:refnum<queue>)  [unwired: 1 in, 6 out]
      }
      event "Mechanism Motion": Value Change {
        n414 = event-data() -> ()  [unwired: 2 out]
        n415 = call "Enqueue Message (Single).vi"("Message Data"="Mechanism Motion", "Message"="Stress Control - Update Motion Mode", "Message Queue"=w877) -> ("error out"=w875:errorcluster, "dup Message Queue"=w876:refnum<queue>)  [unwired: 1 in, 6 out]
      }
      event "Speed (°/s)": Value Change {
        n416 = event-data() -> ()  [unwired: 2 out]
        n417 = call "Enqueue Message (Single).vi"("Message Data"="Speed (°/s)", "Message"="Stress Control - Update Configuration", "Message Queue"=w882) -> ("error out"=w880:errorcluster, "dup Message Queue"=w881:refnum<queue>)  [unwired: 1 in, 6 out]
      }
      event "Destination (°)": Value Change {
        n418 = event-data() -> ()  [unwired: 2 out]
        n419 = call "Enqueue Message (Single).vi"("Message Data"="Destination (°)", "Message"="Stress Control - Update Destination", "Message Queue"=w885) -> ("error out"=w887:errorcluster, "dup Message Queue"=w886:refnum<queue>)  [unwired: 1 in, 6 out]
      }
      event "Apply Stress": Value Change {
        n420 = event-data() -> ()  [unwired: 2 out]
        n421 = call "Enqueue Message (Single).vi"("Message"="Stress Control - Change Stress", "Message Queue"=w891) -> ("error out"=w889:errorcluster, "dup Message Queue"=w890:refnum<queue>)  [unwired: 2 in, 6 out]
      }
      event "Stop": Value Change {
        n422 = event-data() -> ()  [unwired: 2 out]
      }
      event "Pameter Analyzer VISA Session": Value Change {
        n423 = event-data() -> ()  [unwired: 2 out]
        n424 = call "Enqueue Message (Single).vi"("Message Data"="Pameter Analyzer VISA Session", "Message"="Parameter Analyzer - Update Visa Session", "Message Queue"=w894) -> ("error out"=w896:errorcluster, "dup Message Queue"=w895:refnum<queue>)  [unwired: 1 in, 6 out]
      }
      event "User Integration Time.Integration Time", "User Integration Time.Short Integration Time (s)", "User Integration Time.Long Integration Time (s)", "User Integration Time.Wait Time Parameter": Value Change {
        n425 = event-data() -> ()  [unwired: 3 out]
        n426 = call "Enqueue Message (Single).vi"("Message Data"="User Integration Time", "Message"="Parameter Analyzer - Configure Integration time", "Message Queue"=w900) -> ("error out"=w902:errorcluster, "dup Message Queue"=w901:refnum<queue>)  [unwired: 1 in, 6 out]
      }
      event "Apply Sweeping Settings": Value Change {
        n427 = event-data() -> ()  [unwired: 3 out]
        n428 = Bundle("SMU 1 - Sweeping"="SMU 1 - Sweeping", "SMU 2 - Sweeping"="SMU 2 - Sweeping", "SMU 3 - Sweeping"="SMU 3 - Sweeping", "SMU 4 - Sweeping"="SMU 4 - Sweeping", "Sweep Spacing"="Sweep Spacing", "Range"="Range") -> (w908:T87)  [unwired: 1 out]
        n429 = call "Enqueue Message (Single).vi"("Message Data"=w908, "Message"="Parameter Analyzer - Configure Sweeping", "Message Queue"=w911) -> ("error out"=w913:errorcluster, "dup Message Queue"=w912:refnum<queue>)  [unwired: 1 in, 6 out]
      }
      event "Apply Sampling Settings": Value Change {
        n430 = event-data() -> ()  [unwired: 3 out]
        n431 = Bundle("SMU1 - Sampling"="SMU1 - Sampling", "SMU2 - Sampling"="SMU2 - Sampling", "SMU3 - Sampling"="SMU3 - Sampling", "SMU4 - Sampling"="SMU4 - Sampling", "Sampling Parameters"="Sampling Parameters", "Stop Condition"="Stop Condition") -> (w920:T78)  [unwired: 1 out]
        n432 = call "Enqueue Message (Single).vi"("Message Data"=w920, "Message"="Parameter Analyzer - Configure Sampling", "Message Queue"=w922) -> ("error out"=w924:errorcluster, "dup Message Queue"=w923:refnum<queue>)  [unwired: 1 in, 6 out]
      }
      event "Acquisition Mode": Value Change {
        n433 = event-data() -> ()  [unwired: 2 out]
        n434 = call "Enqueue Message (Single).vi"("Message Data"="Acquisition Mode", "Message"="Parameter Analyzer - Update Acquisition Mode", "Message Queue"=w927) -> ("error out"=w929:errorcluster, "dup Message Queue"=w928:refnum<queue>)  [unwired: 1 in, 6 out]
      }
      event "Parameter Analyzer - Measure": Value Change {
        n435 = event-data() -> ()  [unwired: 2 out]
        n436 = call "Enqueue Message (Single).vi"("Message"="Parameter Analyzer - Measure", "Message Queue"=w931) -> ("error out"=w933:errorcluster, "dup Message Queue"=w932:refnum<queue>)  [unwired: 2 in, 6 out]
      }
      event "Parameter Analyzer - Save Measurement": Value Change {
        n437 = event-data() -> ()  [unwired: 3 out]
        n438 = call "Enqueue Message (Single).vi"("Message"="Parameter Analyzer - Save Measurement", "Message Queue"=w935) -> ("error out"=w936:errorcluster, "dup Message Queue"=w937:refnum<queue>)  [unwired: 2 in, 6 out]
      }
      event "Switching Matrix VISA Session": Value Change {
        n439 = event-data() -> ()  [unwired: 2 out]
        n440 = call "Enqueue Message (Single).vi"("Message Data"="Switching Matrix VISA Session", "Message"="Switching Matrix - Update Visa Session", "Message Queue"=w939) -> ("error out"=w941:errorcluster, "dup Message Queue"=w940:refnum<queue>)  [unwired: 1 in, 6 out]
      }
      event "Switching Matrix Connections": Value Change {
        n441 = event-data() -> ()  [unwired: 2 out]
        n442 = call "Enqueue Message (Single).vi"("Message Data"="Switching Matrix Connections", "Message"="Switching Matrix - Set Connections", "Message Queue"=w944) -> ("error out"=w946:errorcluster, "dup Message Queue"=w945:refnum<queue>)  [unwired: 1 in, 6 out]
      }
      event "Disconnect All": Value Change {
        n443 = event-data() -> ()  [unwired: 2 out]
        n444 = call "Enqueue Message (Single).vi"("Message"="Switching Matrix - Disconnect All", "Message Queue"=w948) -> ("error out"=w950:errorcluster, "dup Message Queue"=w949:refnum<queue>)  [unwired: 2 in, 6 out]
      }
      event "Ground All": Value Change {
        n445 = event-data() -> ()  [unwired: 2 out]
        n446 = call "Enqueue Message (Single).vi"("Message"="Switching Matrix - Ground All", "Message Queue"=w952) -> ("error out"=w954:errorcluster, "dup Message Queue"=w953:refnum<queue>)  [unwired: 2 in, 6 out]
      }
      event "Instrument Sequence - Start": Value Change {
        n447 = event-data() -> ()  [unwired: 3 out]
        n448 = call "Enqueue Message (Single).vi"("Message"="Instrument Sequence - Start Sequence", "Message Queue"=w957) -> ("error out"=w958:errorcluster, "dup Message Queue"=w959:refnum<queue>)  [unwired: 2 in, 6 out]
      }
      event "Instrument Sequence - Stop": Value Change {
        n449 = event-data() -> ()  [unwired: 3 out]
        n450 = call "Enqueue Message (Single).vi"("Message"="Instrument Sequence - Stop Sequence", "Message Queue"=w961) -> ("error out"=w962:errorcluster, "dup Message Queue"=w963:refnum<queue>)  [unwired: 2 in, 6 out]
      }
      event "Instrument Sequence - Pause": Value Change {
        n451 = event-data() -> ()  [unwired: 3 out]
        n452 = case shown="True" "Instrument Sequence - Pause" {
          tunnel: [w969 w973] -> w967
          tunnel: [errorcluster {"status"=FALSE, "code"=0, "source"=""} ("error out") w972] -> w966
          tunnel: w965 -> [w969 w971]
          frame False {
          }
          frame True {
            n453 = call "Enqueue Message (Single).vi"("Message"="Instrument Sequence - Pause Sequence", "Message Queue"=w971) -> ("error out"=w972:errorcluster, "dup Message Queue"=w973:refnum<queue>)  [unwired: 2 in, 6 out]
          }
        }
      }
      event "Strain Measurement - Stress Sequence Parameters": Value Change {
        n454 = event-data() -> ()  [unwired: 2 out]
        n455 = call "Enqueue Message (Single).vi"("Message Data"="Strain Measurement - Stress Sequence Parameters", "Message"="Strain Measurement - Update Strain Sequence", "Message Queue"=w976) -> ("error out"=w978:errorcluster, "dup Message Queue"=w977:refnum<queue>)  [unwired: 1 in, 6 out]
      }
      event "Strain Measurement - Start": Value Change {
        n456 = event-data() -> ()  [unwired: 3 out]
        n457 = call "Enqueue Message (Single).vi"("Message"="Strain Measurement - Start", "Message Queue"=w980) -> ("error out"=w982:errorcluster, "dup Message Queue"=w981:refnum<queue>)  [unwired: 2 in, 6 out]
      }
      event "Strain Measurement - Pause": Value Change {
        n458 = event-data() -> ()  [unwired: 3 out]
        n459 = call "Enqueue Message (Single).vi"("Message"="Strain Measurement - Pause", "Message Queue"=w984) -> ("error out"=w986:errorcluster, "dup Message Queue"=w985:refnum<queue>)  [unwired: 2 in, 6 out]
      }
      event "Strain Measurement - Stop": Value Change {
        n460 = event-data() -> ()  [unwired: 3 out]
        n461 = call "Enqueue Message (Single).vi"("Message"="Strain Measurement - Stop", "Message Queue"=w988) -> ("error out"=w990:errorcluster, "dup Message Queue"=w989:refnum<queue>)  [unwired: 2 in, 6 out]
      }
      event "Strain Measurement - New Sequence": Value Change {
        n462 = event-data() -> ()  [unwired: 3 out]
        n463 = call "Enqueue Message (Single).vi"("Message"="Strain Measurement - New Sequence", "Message Queue"=w992) -> ("error out"=w994:errorcluster, "dup Message Queue"=w993:refnum<queue>)  [unwired: 2 in, 6 out]
      }
      event "Strain Measurement - Add Step": Value Change {
        n464 = event-data() -> ()  [unwired: 3 out]
        n465 = call "Enqueue Message (Single).vi"("Message"="Strain Measurement - Add Step", "Message Queue"=w996) -> ("error out"=w998:errorcluster, "dup Message Queue"=w997:refnum<queue>)  [unwired: 2 in, 6 out]
      }
      event "Strain Measurement - Delete Step": Value Change {
        n466 = event-data() -> ()  [unwired: 3 out]
        n467 = call "Enqueue Message (Single).vi"("Message"="Strain Measurement - Delete Step", "Message Queue"=w1000) -> ("error out"=w1002:errorcluster, "dup Message Queue"=w1001:refnum<queue>)  [unwired: 2 in, 6 out]
      }
      event "Strain Measurement - Save Sequence": Value Change {
        n468 = event-data() -> ()  [unwired: 3 out]
        n469 = call "Enqueue Message (Single).vi"("Message"="Strain Measurement - Save Sequence", "Message Queue"=w1004) -> ("error out"=w1006:errorcluster, "dup Message Queue"=w1005:refnum<queue>)  [unwired: 2 in, 6 out]
      }
      event "Strain Measurement - Load Sequence": Value Change {
        n470 = event-data() -> ()  [unwired: 3 out]
        n471 = call "Enqueue Message (Single).vi"("Message"="Strain Measurement - Load Sequence", "Message Queue"=w1008) -> ("error out"=w1010:errorcluster, "dup Message Queue"=w1009:refnum<queue>)  [unwired: 2 in, 6 out]
      }
      event "PlotData - Instrument Sequence", "PlotData - Strain Sequence": Value Change {
        n472 = event-data() -> ()  [unwired: 3 out]
        n473 = Bundle("PlotData - Instrument Sequence"="PlotData - Instrument Sequence", "PlotData - Strain Sequence"="PlotData - Strain Sequence") -> (w1011:T83)  [unwired: 1 out]
        n474 = call "Enqueue Message (Single).vi"("Message Data"=w1011, "Message"="PlotData - Update Plots", "Message Queue"=w1015) -> ("error out"=w1017:errorcluster, "dup Message Queue"=w1016:refnum<queue>)  [unwired: 1 in, 6 out]
      }
    }
    n475 = call "Event Handling Loop.vi"("error in (no error)"=w843, "Message Queue"=w841) -> ("dup error in"=w844:errorcluster)  [unwired: 9 out]
  }
  n476 = Unregister For Events(event registration refnum=w28, error in=w30) -> (error out=w22:errorcluster)
  n477 = Merge Errors(w22, w21, w20, w1, w18, w17, w16, w15, w19) -> (w14:errorcluster)
  n478 = call "Destroy User Event - Stop.vi"("error in (no error)"=w14, "User Event - Stop"=w25) -> ("error out"=w12:errorcluster)  [unwired: 9 out]
  n479 = call "Close Notifiers.vi"("error in"=w14, "Notifiers"=w4) -> ("error out"=w11:errorcluster)  [unwired: 9 out]
  n480 = Merge Errors(w12, w11) -> (w13:errorcluster)
  n481 = property class="App"(error in=w13) -> (error out=w26:errorcluster, "App.Kind"=w27:T88)  [unwired: 1 in, 1 out]
  n482 = case shown="\"Development System\"" w27 {
    tunnel: w26 -> [w1018 w1019 _ _ _ _ _]
    frame "invalid app kind", Default {
      n483 = call <vilib>:"Simple Error Handler.vi"("error in (no error)"=w1018) -> ()  [unwired: 1 in, 8 out]
    }
    frame "Development System" {
      n484 = call <vilib>:"Simple Error Handler.vi"("error in (no error)"=w1019) -> ()  [unwired: 1 in, 8 out]
    }
    frame "Run Time System" {
      n485 = Quit LabVIEW() -> ()  [unwired: 1 out]
    }
    frame "Student Edition" {
    }
    frame "Embedded LabVIEW" {
    }
    frame "Evaluation" {
    }
    frame "Custom" {
    }
  }
